vi "Q14070-Z060A.vi"() -> ()   [LabVIEW 2013]
uses:
  <vilib>/Utility/error.llb/whitespace.ctl
  <vilib>/Utility/file.llb/Read From Spreadsheet File (string).vi
  <vilib>/express/express arith-compare/Formula/XNode/ExpressFormulaBlockNode.xnode
  PCI8622_32.dll
  <vilib>/printing/EasyPrintingControls.llb/contents.ctl
  <vilib>/Utility/NIReport.llb/NI_ReportGenerationCore.lvlib
  <vilib>/printing/EasyPrintingControls.llb/report_type.ctl
  <vilib>/printing/EasyPrinting.llb/Easy Print VI Panel or Documentation (path).vi
  <vilib>/Utility/NIReport.llb/NI_report.lvclass
panel:
  out "齿条跑和右极限":dbl=10000.0 format="%#.3f"
  out "齿条跑和左极限":dbl=10000.0 format="%#.3f"
  in  "确定按钮 3":bool
  in  "确定按钮 2":bool
  in  "密码":string
  in  "确定按钮":bool
  in  "电动缸快速":dbl=15.0
  in  "电动缸慢速":dbl=1.0
  out "左轴向力数组大小":i32
  out "循环退出":bool
  in  "截取百分比":dbl=0.05
  in  "半行程":dbl=70.0
  in  "是否取消放行按钮":bool
  in  "齿条传动比":dbl=47.34 format="%#_13g"
  in  "机械间隙值":dbl=3.5
  out "最大轴向力标准(N)":dbl=200.0 caption="L+Lmax(mm)" format="%#.3f"
  out "右平均轴向力(N)":dbl caption="L+Lmax(mm)" format="%#.3f"
  out "左平均轴向力(N)":dbl caption="最大位移偏离Lmax(mm)" format="%#.3f"
  out "员工ID":string
  out "急停":bool
  out "报警":dbl
  out "报警提示":string
  out "DeviceHandle":u32
  in  "设定轴向力调整次数":dbl=6.0
  out "出支线工步号":u32
  in  "最小间隙(mm)":dbl=0.001 format="%#.3f"
  in  "测头气缸右移":bool
  in  "测头气缸左移":bool
  in  "轴向力已做次数":dbl
  out "全行程间隙及轴向力合格":bool
  out "轴向力启动":bool
  out "间隙启动":bool
  in  "夹头松开":bool
  in  "夹头夹紧":bool
  out "找帽扭矩":dbl=10.0 caption="压力传感器" format="%#.2f"
  out "error out":errorcluster
  out "型号数量":i32
  out "error out 4":errorcluster
  in  "设定间隙调整次数":dbl=6.0
  out "读取产品ID":string
  out "下工位备料":bool
  out "下工位测试":bool
  out "下工位自动":bool
  out "下工位备料H":bool
  out "下工位测试H":bool
  out "下工位自动H":bool
  out "FGCS":string
  out "KSJJ":string
  out "Z060ARFID":string
  out "轴向力Y":dbl[](array[numeric])
  out "轴向力X":dbl[](array[numeric])
  out "间隙X数组":dbl[](array[numeric])
  out "间隙Y数组":dbl[](array[numeric])
  out "error out 3":errorcluster caption="错误输出"
  out "rfid工步号":u32
  out "芯片ID":string="201209190001"
  out "rfid完成":bool
  out "rfid触发":bool
  out "本序已做":bool
  in  "回零完成":bool
  in  "电动缸回零":bool
  in  "已调试次数":dbl
  in  "需调整角度(度)":dbl
  in  "转向器中心":dbl
  out "扭矩到达":bool
  out "黄灯":bool
  out "红灯":bool
  in  "基准位移":dbl caption="压力传感器" format="%#.3f"
  out "上序不合格":bool
  out "单点间隙合格":bool
  out "上序合格":bool
  out "测头机构电机":u32
  out "复位":bool
  in  "型号选择":u16(ring)=2 items=["J709", "J728", "J706"]
  in  "联线按钮":bool
  in  "工步号":u32
  in  "产品ID":string="201209190001"
  out "间隙位移(mm)":dbl caption="压力传感器" format="%#.3f"
  out "齿条推拉力(N)":dbl format="%#.2f"
  out "齿条扭矩(Nm)":dbl format="%#.2f"
  out "通讯状态":bool
  out "员工姓名":string
  out "工步提示":string
  out "ADODB._Connection Out 2":refnum<k7>
  out "旋转齿条电机":u32
  out "电动缸电机":u32
  in  "停止":bool
  in  "参数加载":bool
  in  "选项卡控件":T1(tab)
  out "扭动曲线":cluster{"Y":dbl[], "Y":dbl[]}[](graph) caption="压球涨堵头1"
  out "中间位置间隙":dbl caption="间隙值L(mm)" format="%_2f"
  out "中间间隙标准(mm)":dbl=0.07 format="%#.3f"
  in  "找帽OK":bool
  out "全行程180°外间隙标准(mm)":dbl=0.1 format="%#.3f"
  out "右180°外全行程间隙":dbl caption="正向最大间隙L1(mm)" format="%_2f"
  out "左180°外全行程间隙":dbl caption="正向最大间隙L1(mm)" format="%_2f"
  out "右180°内全行程间隙":dbl caption="正向最大间隙L1(mm)" format="%_2f"
  out "左180°内全行程间隙":dbl caption="正向最大间隙L1(mm)" format="%_2f"
  out "全行程180°内间隙标准(mm)":dbl=0.07 format="%_1f"
  out "左全行程间隙":dbl caption="正向最大间隙L1(mm)" format="%#.3f"
  out "右全行程间隙":dbl caption="正向最大间隙L1(mm)" format="%#.3f"
  out "总圈数最大值":dbl format="%_3g"
  out "总圈数标准":dbl format="%_3g"
  out "总行程最大值":dbl
  out "总行程标准(mm)":dbl
  out "平均轴向力MAX(N)":dbl=200.0 caption="L+Lmax(mm)" format="%#.3f"
  out "力波动标准(N)":dbl=60.0 caption="L+Lmax(mm)" format="%#.3f"
  out "轴向力标准(N)":dbl=100.0 caption="L+Lmax(mm)" format="%#.3f"
  out "右最大轴向力(N)":dbl caption="L+Lmax(mm)" format="%#_5f"
  out "左轴向力波动(N)":dbl caption="最大位移偏离Lmax(mm)" format="%#_4f"
  out "左最大轴向力(N)":dbl caption="最大位移偏离Lmax(mm)" format="%#_5f"
  out "行程跳动曲线":cluster{"Y":dbl[], "Y":dbl[]}[](graph) caption="压球涨堵头1"
  out "右轴向力波动(N)":dbl format="%#_4f"
  out "总行程(mm)":dbl format="%#_5f"
  out "总圈数":dbl format="%.3g"
  in  "不合格品":bool
  in  "扭矩停止值":dbl=16.0
  in  "齿条右极限":dbl=-70.0 caption="压力传感器" format="%#.2f"
  in  "齿条左极限":dbl=-262.0 caption="压力传感器" format="%#.2f"
  in  "齿条移动速度":dbl=5.0 caption="压力传感器" format="%#.2f"
  in  "旋转伺服找帽转速":dbl=5.0 caption="压力传感器" format="%#.2f"
  in  "测量点扭矩":dbl=4.0 caption="压力传感器" format="%#.2f"
  in  "旋转伺服测量转速":dbl caption="压力传感器" format="%#.2f"
  in  "测头机构轴后退位":dbl=30.0 caption="压力传感器" format="%#.2f"
  in  "测头机构轴待检位":dbl caption="压力传感器" format="%#.2f"
  in  "测头机构轴检测位":dbl caption="压力传感器" format="%#.2f"
  in  "测头机构轴移动速度":dbl caption="压力传感器" format="%#.2f"
  out "点胶":bool
  in  "夹头松开":bool
  in  "夹头夹紧":bool
  in  "测头气缸右移":bool
  in  "测头气缸左移":bool
  in  "支线下降":bool
  in  "支线顶升":bool
  in  "出支线":bool
  in  "进支线":bool
  in  "主线下降":bool
  in  "主线顶升":bool
  in  "下阻挡器放行":bool
  in  "上阻挡器放行":bool
  out "夹头夹紧位":bool
  out "测头左位":bool
  out "测头右位":bool
  out "夹头松开":bool
  out "记号笔":bool
  in  "测头机构轴使能":bool
  in  "测头机构轴后退":bool
  in  "测头机构轴前进":bool
  in  "电动缸速度(mm/s)":dbl=10.0 format="%#.3f"
  out "电动缸位置(mm)":dbl=10000.0 format="%#.3f"
  in  "旋转伺服速度(°/s)":dbl=10.0 format="%#.3f"
  out "旋转伺服位置(°)":dbl=10000.0 format="%#.3f"
  in  "测头机构轴速度(mm/s)":dbl=10.0 format="%#.3f"
  out "测头机构轴位置(mm)":dbl=10000.0 format="%#.3f"
  in  "旋转齿条轴右转":bool
  in  "旋转齿条轴左转":bool
  in  "旋转齿条轴使能":bool
  in  "电动缸后退":bool
  in  "电动缸使能":bool
  in  "电动缸前进":bool
  in  "齿条扭矩比例偏移":dbl=1.0 format="%#.2f"
  in  "齿条扭矩零点偏移":dbl format="%#.2f"
  in  "齿条推拉力比例偏移":dbl=1.0 format="%#.2f"
  in  "齿条推拉力零点偏移":dbl format="%#.2f"
  in  "间隙位移比例偏移":dbl=1.0 format="%#.2f"
  in  "间隙位移零点偏移":dbl format="%#.2f"
  in  "传感器参数保存":bool
  in  "参数修改":bool
  in  "参数查询":bool
  in  "参数浏览表":string[][](table)
  # "芜湖机械转向器装配线"
  # "间隙及轴向力检测"
  # "Q14070机械转向器装配线"
  # "湖北唯思凌科装备制造有限公司 设计开发 (C)2015"
  # "≤"
  # "间隙测量判定值"
  # "间隙测量结果"
  # "≤"
  # "≤"
  # "≤"
  # "轴向力测量结果"
  # "轴向力测量标准"
  # "≤"
  # "≥"
  # "≤"
  # "≥"
  # "≤"
  # "≥"
  # "≤"
  # "不得大于20NM"
  # "传感器校验区"
  # "关于传感器校验：\n1、传感器校验需要由具备资质的单位或部门进行校验。\n2、具备权限的用户才能够修改传感器校验参数和试验参数。\n3、修改校验参数方法：先将比例偏移置为1，修改零点偏移，使零点值与校验的传感器一致；然后根据增幅调整比例偏移。"
  # "注意：\n具备权限的用户才能够修改传感器校验参数和试验参数！"
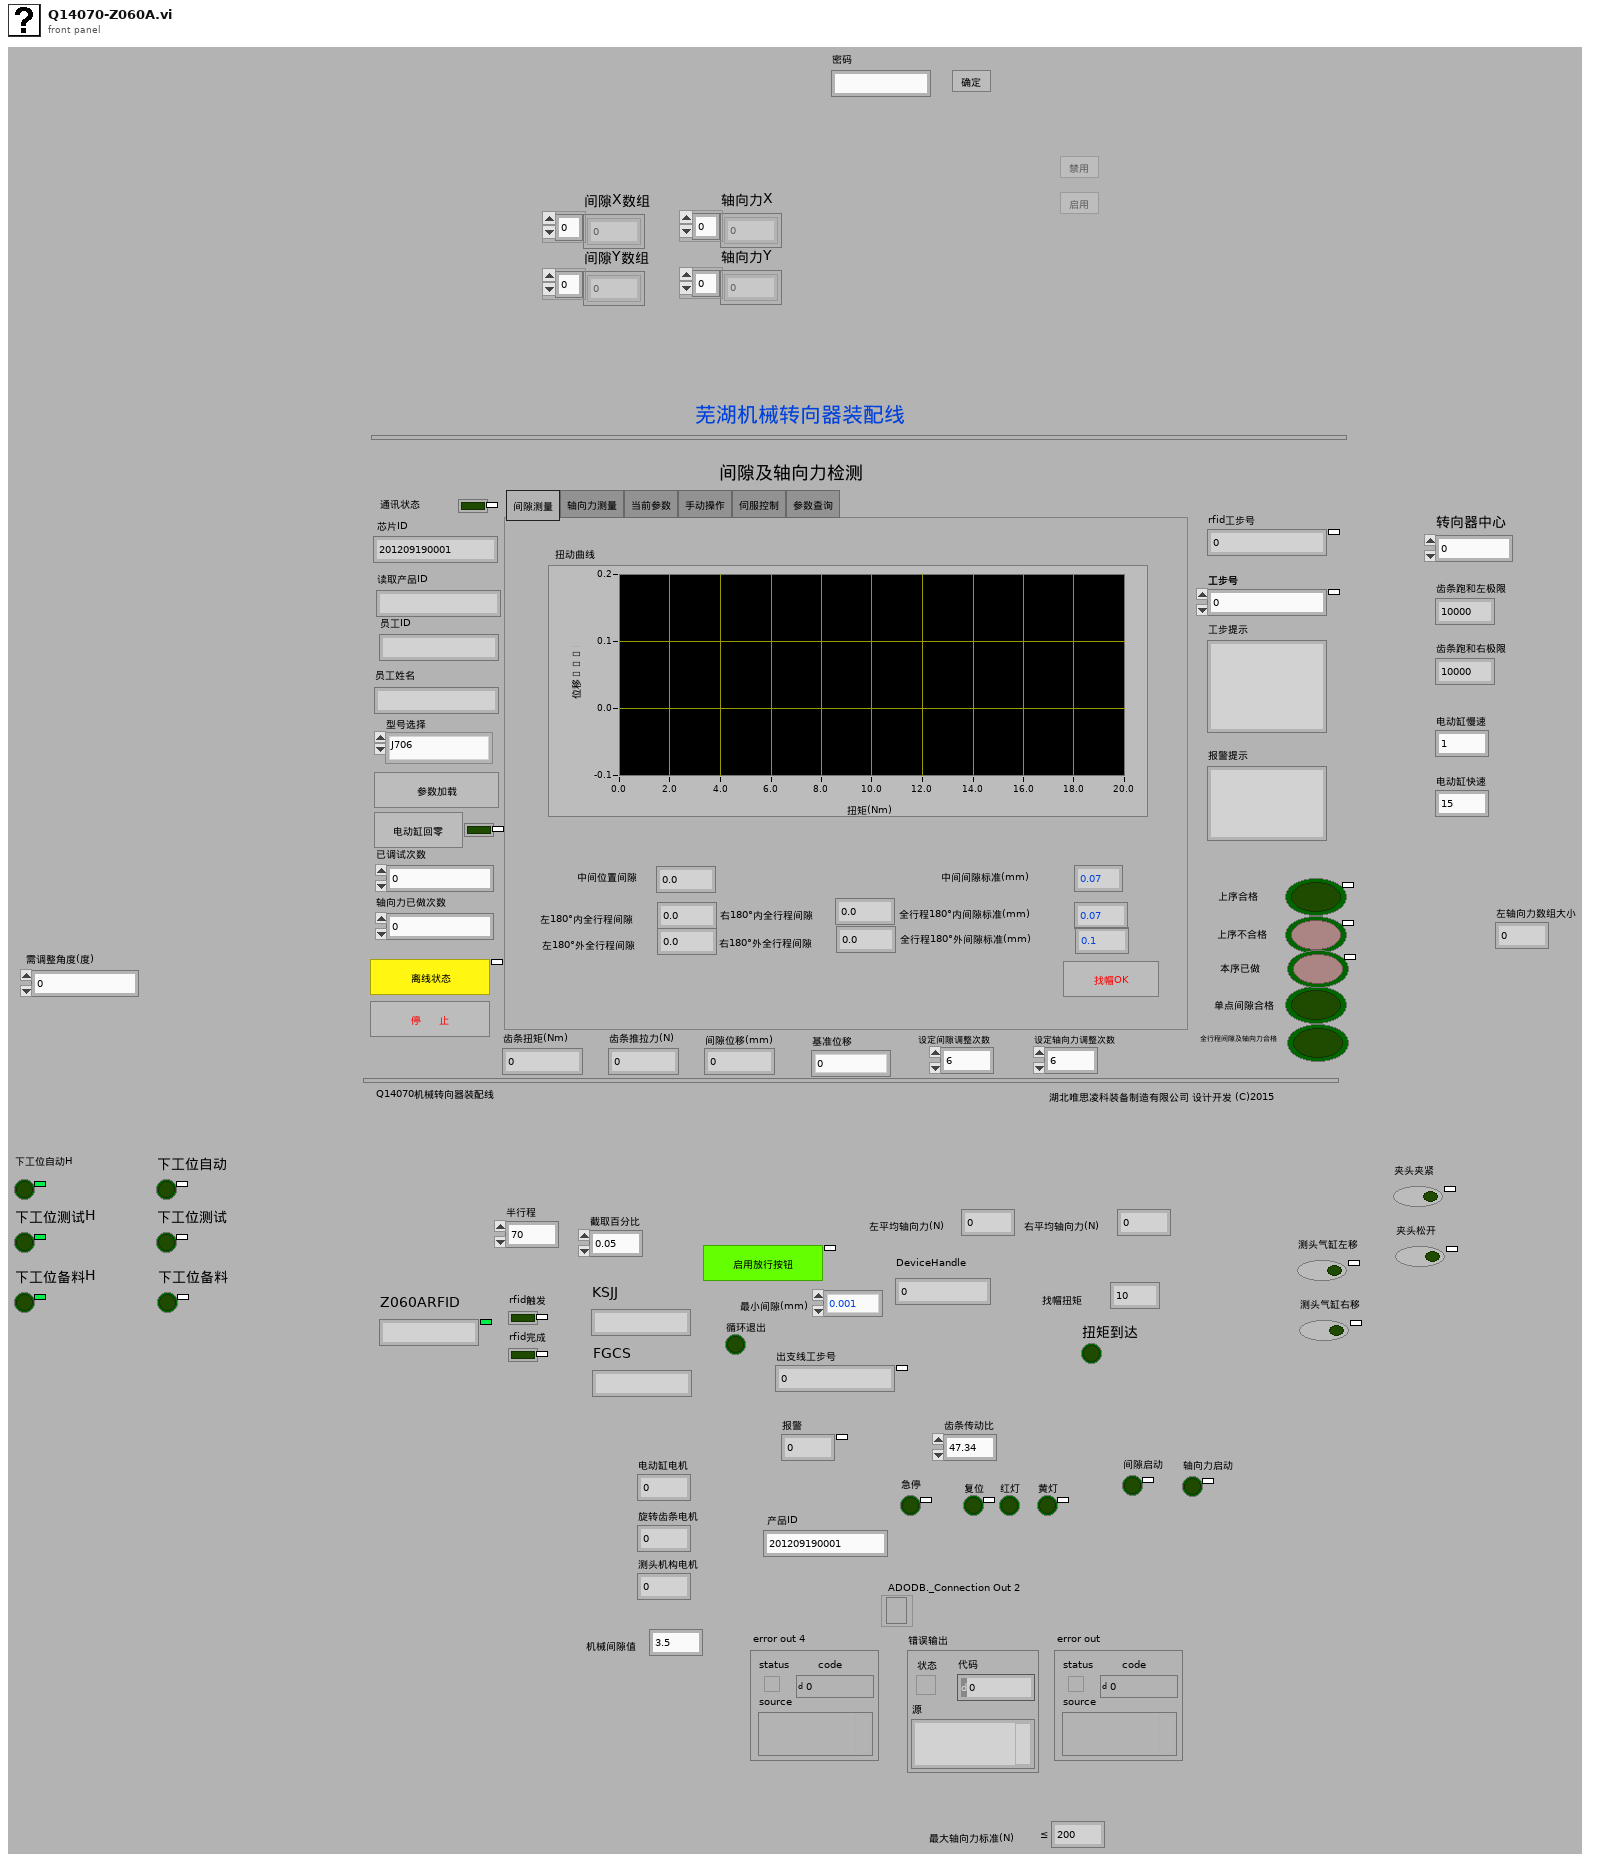
[diagram p1: front panel]
types:
  T1 = enum32{"间隙测量", "轴向力测量", "当前参数", "手动操作", "伺服控制", "传感器校验", "参数查询"}
  T2 = enum8{"Enabled", "Disabled", "Disabled and Grayed Out"}
  T3 = typedef "NI_ReportGenerationCore.lvlib/report_type.ctl" = u16
  T4 = typedef "NI_ReportGenerationCore.lvlib/contents.ctl" = u16
  T5 = typedef "imagedata.ctl" = cluster{"image type":i32, "image depth":i32, "image":u8[], "mask":u8[], "colors":u32[], "Rectangle":cluster{"left":i16, "top":i16, "right":i16, "bottom":i16}}
  T6 = typedef "whitespace.ctl" = u16
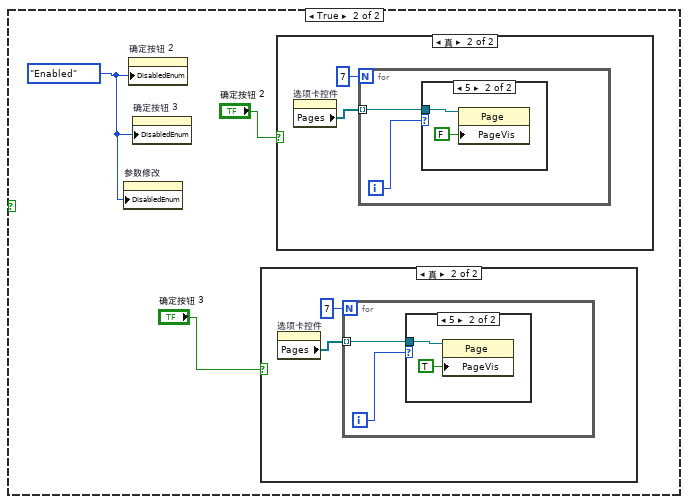
[diagram p2: hidden frame]
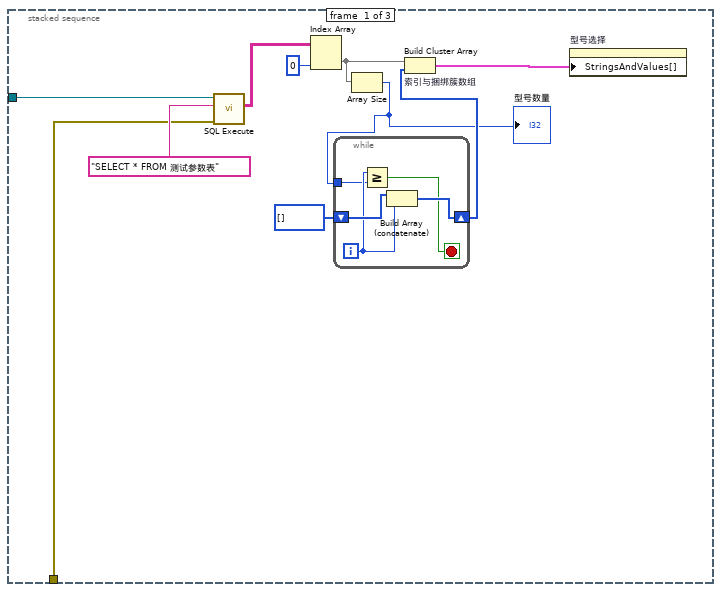
[diagram p9: hidden frame]
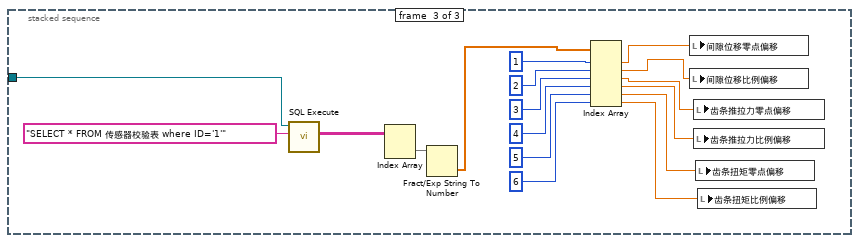
[diagram p10: hidden frame]
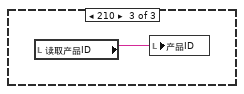
[diagram p12: hidden frame]
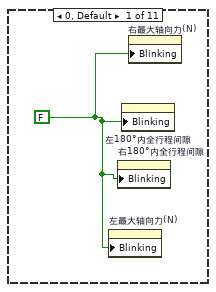
[diagram p13: hidden frame]
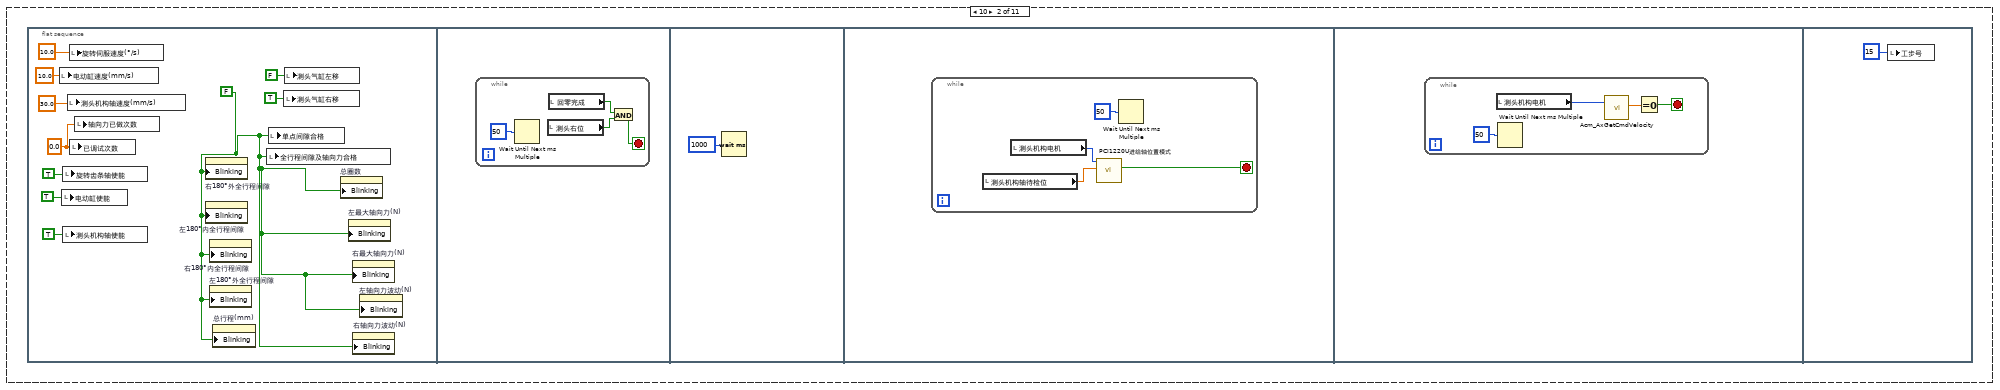
[diagram p14: hidden frame]
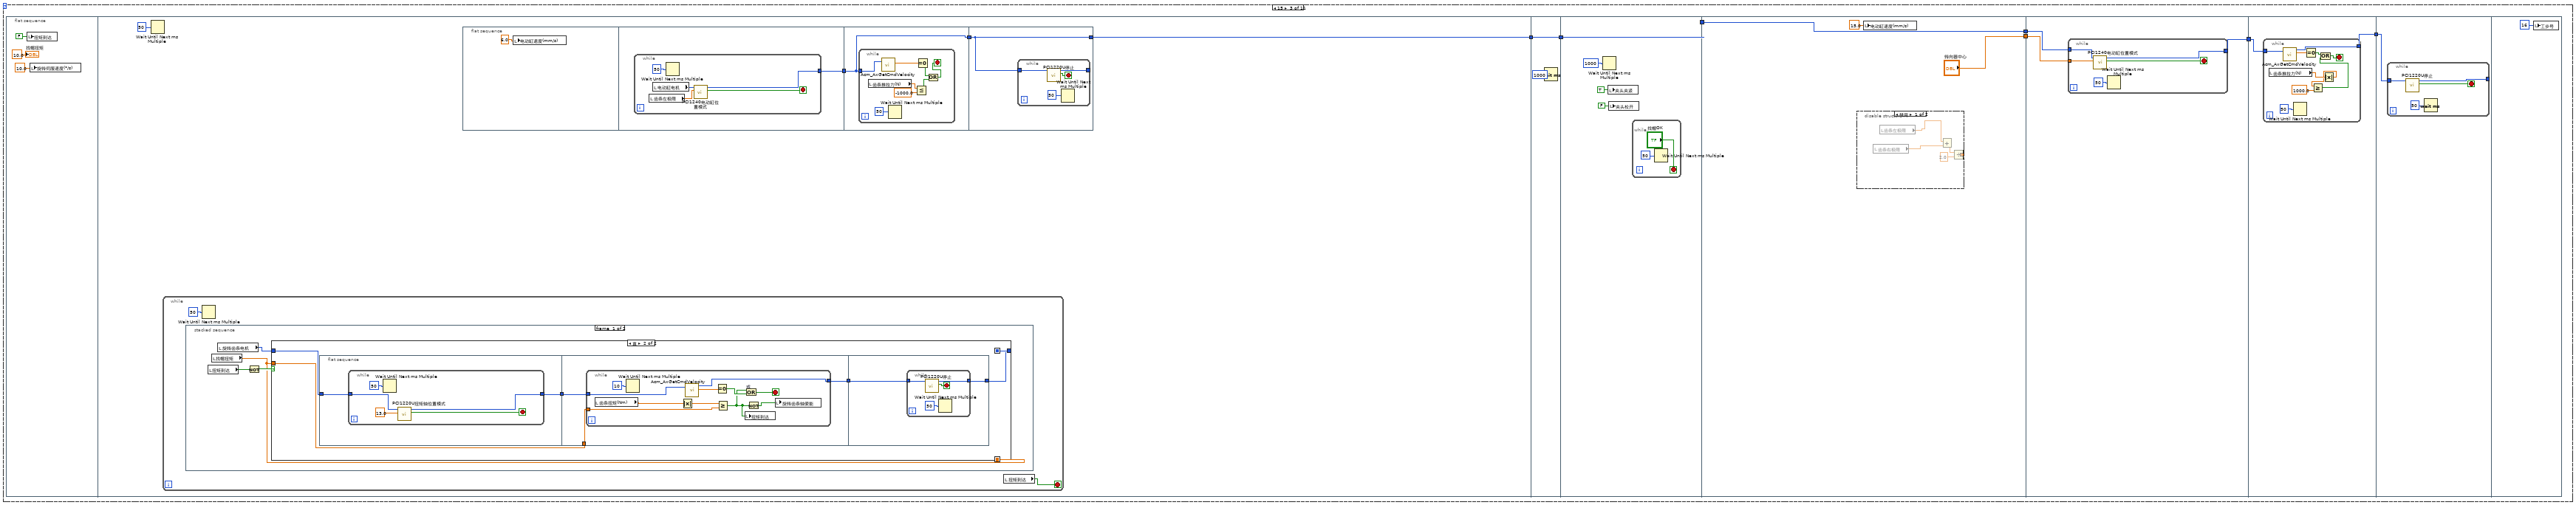
[diagram p15: hidden frame]
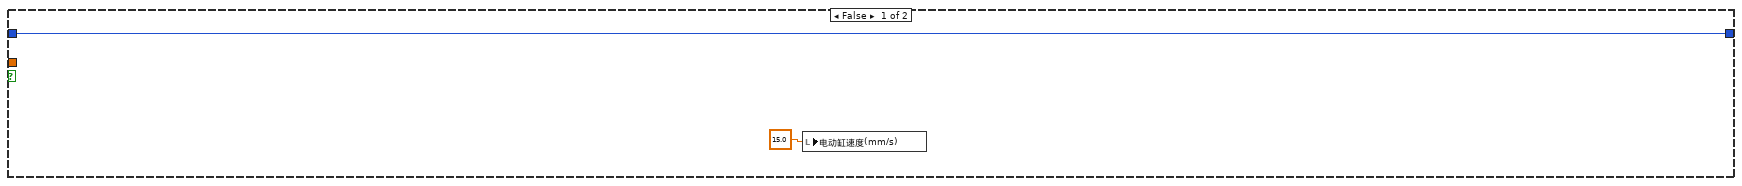
[diagram p16: hidden frame]
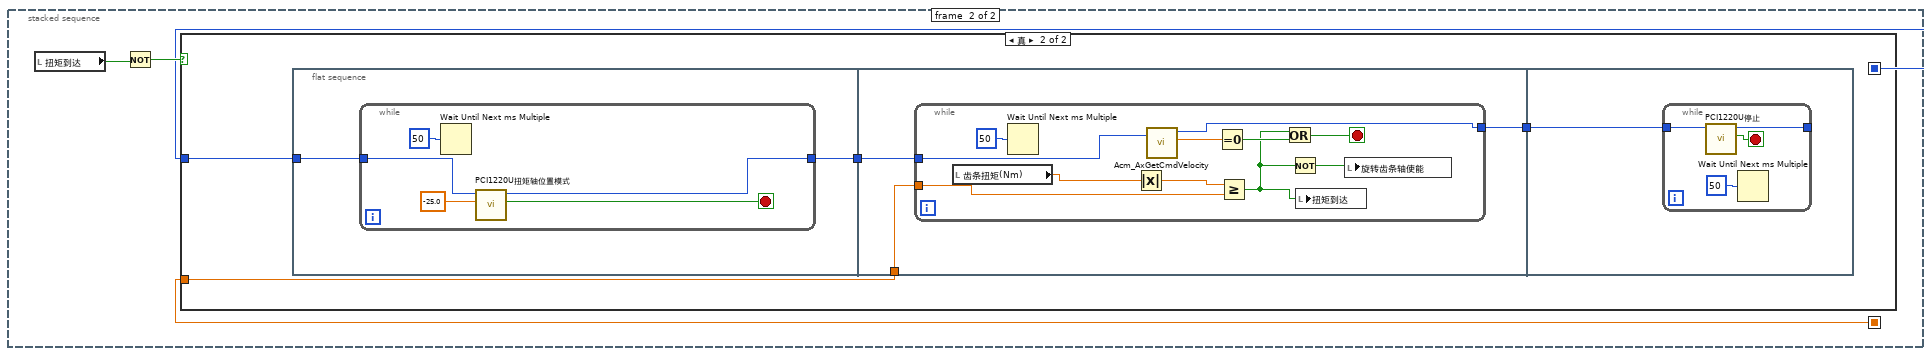
[diagram p17: hidden frame]
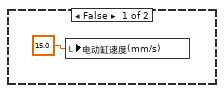
[diagram p18: hidden frame]
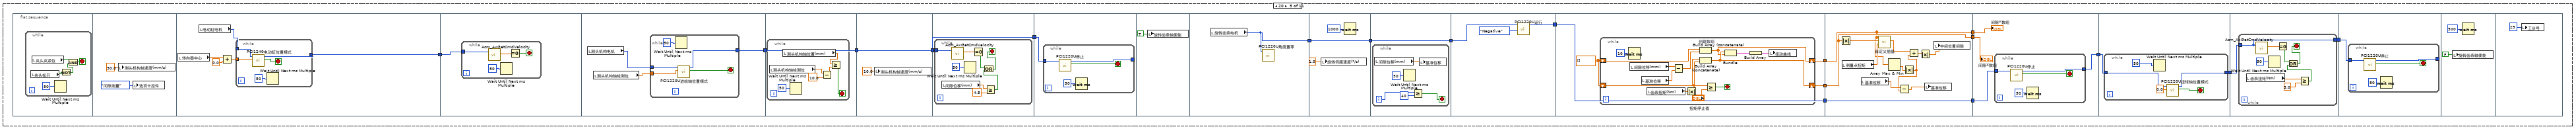
[diagram p20: hidden frame]
diagram:
  n1 = while {
    stop <- w5 stop-if-true
    n2 = event shown="[2] \"参数修改\": 值改变" {
      selector: _ -> [_ _ _ _ _ _]
      dyn-events: _ -> [_ _ _ _ _ _]
      timeout: 500 -> [_ _ _ _ _ _]
      event Timeout {
        n3 = event-data() -> ()  [unwired: 3 out]
      }
      event "停止": Value Change {
        n4 = event-data() -> ()  [unwired: 6 out]
        n5 = flat-sequence {
          frame #0 {
            n6 = Wait (ms)(milliseconds to wait=u32 1000 ("毫秒倍数")) -> ()  [unwired: 1 out]
          }
          frame #1 {
            n7 = Quit LabVIEW(quit? (T)=TRUE ("停止？(T)")) -> ()
          }
        }
      }
      event "参数修改": Value Change {
        n8 = event-data() -> ()  [unwired: 6 out]
        n9 = while {
          i -> [w63]
          stop <- w62 stop-if-true
          n10 = local read "型号数量"() -> (w64:i32)
          n11 = local read "参数浏览表"() -> (w65:string[][])
          n12 = Greater Or Equal?(x=w63, y=w64) -> (x >= y?=w62:bool)
          n13 = Wait Until Next ms Multiple(millisecond multiple=u32 50 ("毫秒倍数")) -> ()  [unwired: 1 out]
          n14 = Index Array(array=w65, index (col)=w63) -> (element=w50:string[])  [unwired: 1 in]
          n15 = Index Array(array=w50, index #1=0 ("索引"), index #2=2 ("索引"), index #3=3 ("索引"), index #4=4 ("索引"), index #5=5 ("索引"), index #6=6 ("索引"), index #7=7 ("索引"), index #8=8 ("索引"), index #9=9 ("索引"), index #10=10 ("索引"), index #11=11 ("索引"), index #12=12 ("索引"), index #13=13 ("索引"), index #14=14 ("索引"), index #15=15 ("索引"), index #16=16 ("索引"), index #17=17 ("索引"), index #18=18 ("索引"), index #19=19 ("索引"), index #20=20 ("索引"), index #21=21 ("索引"), index #22=22 ("索引"), index #23=23 ("索引")) -> (element #1=w16:string, element #2=w46:string, element #3=w45:string, element #4=w44:string, element #5=w43:string, element #6=w42:string, element #7=w41:string, element #8=w40:string, element #9=w39:string, element #10=w38:string, element #11=w37:string, element #12=w32:string, element #13=w31:string, element #14=w30:string, element #15=w29:string, element #16=w28:string, element #17=w23:string, element #18=w22:string, element #19=w21:string, element #20=w17:string, element #21=w15:string, element #22=w14:string, element #23=w13:string)
          n16 = call "创建文本"("测头机构轴移动速度"=w46, "测头机构轴检测位"=w45, "测头机构轴待检位"=w44, "测头机构轴后退位"=w43, "齿条移动速度"=w42, "齿条左极限"=w41, "齿条右极限"=w40, "旋转齿条轴找帽转速"=w39, "旋转齿条轴测量转速"=w38, "测量点扭矩"=w37, "总行程最大值"=w31, "总行程最小值"=w32, "最大轴向力"=w30, "轴向力波动"=w29, "平均轴向力最小值"=w28, "平均轴向力最大值"=w23, "总圈数最小值"=w22, "总圈数最大值"=w21, "中间位置"=w17, "中间间隙标准"=w15, "180内间隙标准"=w14, "180外间隙标准"=w13, "产品型号"=w16) -> ("Result"=w36:string)  [unwired: 3 in, 1 out]
          n17 = local read "ADODB._Connection Out 2"() -> (w35:refnum<k7>)
          n18 = call "SQL Execute.vi"("Command Text"=w36, "ADODB._Connection In"=w35) -> ("error out"=w48:errorcluster, "ADODB._Connection Out"=w49:refnum<k7>)  [unwired: 6 in, 2 out]
          n19 = call "ADO Connection Close.vi"("error in (no error)"=w48, "ADODB._Connection In"=w49) -> ("error out"=→"error out":errorcluster)  [unwired: 8 in, 1 out]
        }
      }
      event "参数查询": Value Change {
        n20 = event-data() -> ()  [unwired: 6 out]
        n21 = flat-sequence {
          tunnel: [w78] -> w71
          tunnel: [w77] -> w70
          tunnel: [w76] -> w67
          tunnel: w71 -> [w82]
          tunnel: w70 -> [w84]
          tunnel: [w84] -> w69
          tunnel: [w83] -> w68
          tunnel: w67 -> [w83]
          tunnel: w69 -> [_]
          tunnel: w68 -> [_]
          frame #0 {
            n22 = call-poly <vilib>:"Read From Spreadsheet File.vi"("file path (dialog if empty)"=path "D:/Q14070-Z060人机界面/参数/参数项.txt") -> ("first row"=w72:string[])  [unwired: 6 in, 4 out]
            n23 = property on="参数浏览表" class="Tbl (严格)"("Row Headers[]"=w72) -> ()  [unwired: 2 in, 2 out]
          }
          frame #1 {
            n24 = local read "ADODB._Connection Out 2"() -> (w75:refnum<k7>)
            n25 = call "SQL Execute.vi"("Command Text"="SELECT * FROM 测试参数表;", "ADODB._Connection In"=w75) -> ("error out"=w76:errorcluster, "Data"=w80:string[][], "ADODB._Connection Out"=w77:refnum<k7>)  [unwired: 6 in, 1 out]
            n26 = Transpose 2D Array(2D array=w80) -> (transposed array=w78:string[][])
            n27 = Index Array(array=w78, index (row)=0 ("索引 (行)")) -> (element=w79:string[])  [unwired: 1 in]
            n28 = property on="参数浏览表" class="Tbl (严格)"("Column Headers[]"=w79) -> ()  [unwired: 2 in, 2 out]
          }
          frame #2 {
            n29 = local write "参数浏览表"(w82) -> ()
          }
          frame #3 {
          }
        }
      }
      event "传感器参数保存": Value Change {
        n30 = event-data() -> ()  [unwired: 6 out]
        n31 = flat-sequence {
          tunnel: [w110] -> w107
          tunnel: [w109] -> w106
          tunnel: [w108] -> w105
          tunnel: [w116] -> w104
          tunnel: w107 -> [w116]
          tunnel: [w115] -> w103
          tunnel: w106 -> [w115]
          tunnel: [w114] -> w102
          tunnel: w105 -> [w114]
          tunnel: [w113] -> w101
          tunnel: [w112] -> w100
          tunnel: [w111] -> w99
          tunnel: [w117] -> w98
          tunnel: [w123] -> w97
          tunnel: w104 -> [w123]
          tunnel: [w122] -> w96
          tunnel: w103 -> [w122]
          tunnel: w102 -> [w121]
          tunnel: [w121] -> w95
          tunnel: [w120] -> w94
          tunnel: w101 -> [w120]
          tunnel: [w119] -> w93
          tunnel: w100 -> [w119]
          tunnel: [w118] -> w92
          tunnel: w99 -> [w118]
          tunnel: w98 -> [w142]
          tunnel: [w142] -> w91
          tunnel: w97 -> [w141]
          tunnel: w96 -> [w134]
          tunnel: w95 -> [w133]
          tunnel: w94 -> [w127]
          tunnel: w93 -> [w126]
          tunnel: w92 -> [w132]
          tunnel: [w131] -> w90
          tunnel: [w130] -> w89
          tunnel: [w129] -> w88
          tunnel: [w125] -> w87
          tunnel: [w124] -> w86
          tunnel: [w128] -> w85
          tunnel: w91 -> [w150]
          tunnel: w90 -> [w149]
          tunnel: w89 -> [w148]
          tunnel: w88 -> [w147]
          tunnel: w87 -> [w146]
          tunnel: w86 -> [w145]
          tunnel: w85 -> [w144]
          frame #0 {
            n32 = local read "齿条推拉力零点偏移"() -> (w109:dbl)
            n33 = local read "间隙位移零点偏移"() -> (w110:dbl)
            n34 = local read "齿条扭矩零点偏移"() -> (w108:dbl)
          }
          frame #1 {
            n35 = local read "齿条推拉力比例偏移"() -> (w112:dbl)
            n36 = local read "间隙位移比例偏移"() -> (w113:dbl)
            n37 = local read "齿条扭矩比例偏移"() -> (w111:dbl)
          }
          frame #2 {
            n38 = local read "ADODB._Connection Out 2"() -> (w117:refnum<k7>)
          }
          frame #3 {
            n39 = Number To Fractional String(number=w141, precision (6)=i16 2 ("精度(6)")) -> (F-format string=w131:string)  [unwired: 2 in]
            n40 = Number To Fractional String(number=w133, precision (6)=i16 2 ("精度(6)")) -> (F-format string=w129:string)  [unwired: 2 in]
            n41 = Number To Fractional String(number=w132, precision (6)=i16 2 ("精度(6)")) -> (F-format string=w128:string)  [unwired: 2 in]
            n42 = Number To Fractional String(number=w134, precision (6)=i16 2 ("精度(6)")) -> (F-format string=w130:string)  [unwired: 2 in]
            n43 = Number To Fractional String(number=w127, precision (6)=i16 2 ("精度(6)")) -> (F-format string=w125:string)  [unwired: 2 in]
            n44 = Number To Fractional String(number=w126, precision (6)=i16 2 ("精度(6)")) -> (F-format string=w124:string)  [unwired: 2 in]
          }
          frame #4 {
            n45 = call "创建文本3"("4"=w146, "6"=w144, "1"=w149, "2"=w148, "3"=w147, "5"=w145) -> ("Result"=w151:string)  [unwired: 8 in, 1 out]
            n46 = call "SQL Execute.vi"("Command Text"=w151, "ADODB._Connection In"=w150) -> ("error out"=→"error out 4":errorcluster)  [unwired: 6 in, 3 out]
          }
        }
      }
      event "产品ID": Value Change {
        n47 = event-data() -> ()  [unwired: 7 out]
        n48 = Format Date/Time String(time format string (%c)="%Y%m%d%H%M" ("时间格式字符串(%c)")) -> (date/time string=w152:string)  [unwired: 2 in]
        n49 = local write "KSJJ"(w152) -> ()
      }
    }
    n50 = Wait (ms)(milliseconds to wait=u32 50 ("毫秒倍数")) -> ()  [unwired: 1 out]
    n51 = local read "停止"() -> (w5:bool)
  }
  n52 = while {
    stop <- FALSE stop-if-true
    n53 = Equal?(x="密码", y="jizhuan") -> (x = y?=w157:bool)
    n54 = Compound Arithmetic op=AND(w157, "确定按钮") -> (w155:bool)
    n55 = case shown="假" w155 {
      frame False {
        w160 = T2."Disabled and Grayed Out" ("禁用")
        n56 = property on="确定按钮 2" class="Bool"("DisabledEnum"=w160) -> ()  [unwired: 2 in, 2 out]
        n57 = property on="确定按钮 3" class="Bool"("DisabledEnum"=w160) -> ()  [unwired: 2 in, 2 out]
        n58 = property on="参数修改" class="Bool"("DisabledEnum"=w160) -> ()  [unwired: 2 in, 2 out]
      }
      frame True {
        w161 = T2."Enabled" ("禁用")
        n59 = property on="参数修改" class="Bool"("DisabledEnum"=w161) -> ()  [unwired: 2 in, 2 out]
        n60 = property on="确定按钮 2" class="Bool"("DisabledEnum"=w161) -> ()  [unwired: 2 in, 2 out]
        n61 = property on="确定按钮 3" class="Bool"("DisabledEnum"=w161) -> ()  [unwired: 2 in, 2 out]
        n62 = case shown="真" "确定按钮 3" {
          frame False {
          }
          frame True {
            n63 = property on="选项卡控件" class="TabCtl (严格)"() -> ("Pages"=w164:refnum<vi>[])  [unwired: 2 in, 2 out]
            n64 = for {
              N: 7 -> [_]
              tunnel: w164 -> [w166] mode=indexing
              i -> [w167]
              n65 = case shown="5" w167 {
                tunnel: w166 -> [_ w169]
                frame 0, Default {
                }
                frame 5 {
                  n66 = property class="Page"(reference=w169, "PageVis"=TRUE ("选项卡可见")) -> ()  [unwired: 1 in, 2 out]
                }
              }
            }
          }
        }
        n67 = case shown="真" "确定按钮 2" {
          frame False {
          }
          frame True {
            n68 = property on="选项卡控件" class="TabCtl (严格)"() -> ("Pages"=w170:refnum<vi>[])  [unwired: 2 in, 2 out]
            n69 = for {
              N: 7 -> [_]
              tunnel: w170 -> [w172] mode=indexing
              i -> [w173]
              n70 = case shown="5" w173 {
                tunnel: w172 -> [_ w175]
                frame 0, Default {
                }
                frame 5 {
                  n71 = property class="Page"(reference=w175, "PageVis"=FALSE ("选项卡可见")) -> ()  [unwired: 1 in, 2 out]
                }
              }
            }
          }
        }
      }
    }
  }
  n72 = while {
    stop <- w178 stop-if-true
    n73 = local read "工步号"() -> (w176:u32)
    n74 = case shown="16" w176 {
      frame 0, Default {
        w179 = FALSE ("闪烁")
        n75 = property on="左最大轴向力(N)" class="DigNum (严格)"("Blinking"=w179) -> ()  [unwired: 2 in, 2 out]
        n76 = property on="右180°内全行程间隙" class="DigNum (严格)"("Blinking"=w179) -> ()  [unwired: 2 in, 2 out]
        n77 = property on="左180°内全行程间隙" class="DigNum (严格)"("Blinking"=w179) -> ()  [unwired: 2 in, 2 out]
        n78 = property on="右最大轴向力(N)" class="DigNum (严格)"("Blinking"=w179) -> ()  [unwired: 2 in, 2 out]
      }
      frame 10 {
        n79 = flat-sequence {
          frame #0 {
            w180 = FALSE ("单点间隙合格")
            w181 = 0.0 ("已调试次数")
            n80 = local write "电动缸速度(mm/s)"(10.0 ("电动缸速度(mm/s)")) -> ()
            n81 = local write "电动缸使能"(TRUE ("电动缸使能")) -> ()
            n82 = local write "旋转齿条轴使能"(TRUE ("旋转齿条轴使能")) -> ()
            n83 = local write "测头机构轴使能"(TRUE ("调整机构轴使能")) -> ()
            n84 = local write "测头机构轴速度(mm/s)"(30.0 ("调整机构轴速度(mm/s)")) -> ()
            n85 = local write "旋转伺服速度(°/s)"(10.0 ("旋转齿条轴速度(°/s)")) -> ()
            n86 = local write "已调试次数"(w181) -> ()
            n87 = local write "轴向力已做次数"(w181) -> ()
            n88 = property on="右180°外全行程间隙" class="DigNum (严格)"("Blinking"=w180) -> ()  [unwired: 2 in, 2 out]
            n89 = property on="左180°内全行程间隙" class="DigNum (严格)"("Blinking"=w180) -> ()  [unwired: 2 in, 2 out]
            n90 = property on="右180°内全行程间隙" class="DigNum (严格)"("Blinking"=w180) -> ()  [unwired: 2 in, 2 out]
            n91 = property on="左180°外全行程间隙" class="DigNum (严格)"("Blinking"=w180) -> ()  [unwired: 2 in, 2 out]
            n92 = property on="总行程(mm)" class="DigNum (严格)"("Blinking"=w180) -> ()  [unwired: 2 in, 2 out]
            n93 = local write "全行程间隙及轴向力合格"(w180) -> ()
            n94 = local write "单点间隙合格"(w180) -> ()
            n95 = local write "测头气缸右移"(TRUE ("测头气缸右移")) -> ()
            n96 = local write "测头气缸左移"(FALSE ("测头气缸左移")) -> ()
            n97 = property on="总圈数" class="DigNum (严格)"("Blinking"=w180) -> ()  [unwired: 2 in, 2 out]
            n98 = property on="左最大轴向力(N)" class="DigNum (严格)"("Blinking"=w180) -> ()  [unwired: 2 in, 2 out]
            n99 = property on="右最大轴向力(N)" class="DigNum (严格)"("Blinking"=w180) -> ()  [unwired: 2 in, 2 out]
            n100 = property on="右轴向力波动(N)" class="DigNum (严格)"("Blinking"=w180) -> ()  [unwired: 2 in, 2 out]
            n101 = property on="左轴向力波动(N)" class="DigNum (严格)"("Blinking"=w180) -> ()  [unwired: 2 in, 2 out]
          }
          frame #1 {
            n102 = while {
              stop <- w190 stop-if-true
              n103 = Wait Until Next ms Multiple(millisecond multiple=u32 50 ("毫秒倍数")) -> ()  [unwired: 1 out]
              n104 = local read "测头右位"() -> (w191:bool)
              n105 = local read "回零完成"() -> (w192:bool)
              n106 = And(x=w192, y=w191) -> (x .and. y?=w190:bool)
            }
          }
          frame #2 {
            n107 = Wait (ms)(milliseconds to wait=u32 1000 ("等待时间（毫秒）")) -> ()  [unwired: 1 out]
          }
          frame #3 {
            n108 = while {
              stop <- w198 stop-if-true
              n109 = local read "测头机构轴待检位"() -> (w195:dbl)
              n110 = local read "测头机构电机"() -> (w196:u32)
              n111 = call "PCI1220U进给轴位置模式.vi"("Distance"=w195, "AxisHandle IN"=w196) -> ("AbsSuccess"=w198:bool)  [unwired: 8 in, 1 out]
              n112 = Wait Until Next ms Multiple(millisecond multiple=u32 50 ("毫秒倍数")) -> ()  [unwired: 1 out]
            }
          }
          frame #4 {
            n113 = while {
              stop <- w201 stop-if-true
              n114 = local read "测头机构电机"() -> (w199:u32)
              n115 = Wait Until Next ms Multiple(millisecond multiple=u32 50 ("毫秒倍数")) -> ()  [unwired: 1 out]
              n116 = call <userlib>:"Acm_AxGetCmdVelocity.vi"("AxisHandle"=w199) -> ("Velocity"=w202:dbl)  [unwired: 1 in, 3 out]
              n117 = Equal To 0?(x=w202) -> (x = 0?=w201:bool)
            }
          }
          frame #5 {
            n118 = local write "工步号"(u32 15 ("工步号")) -> ()
          }
        }
      }
      frame 15 {
        n119 = flat-sequence {
          tunnel: [w215] -> w205
          tunnel: w205 -> [w316]
          tunnel: [w316] -> w204
          tunnel: w204 -> [w319]
          tunnel: [w319] -> w207
          tunnel: [w324] -> w210
          tunnel: ["转向器中心"] -> w209
          tunnel: w207 -> [w324]
          tunnel: w210 -> [w333]
          tunnel: w209 -> [w332]
          tunnel: [w331] -> w208
          tunnel: w208 -> [w340]
          tunnel: [w339] -> w206
          tunnel: w206 -> [w351]
          frame #0 {
            n120 = local write "扭矩到达"(FALSE ("扭矩到达")) -> ()
            n121 = local write "旋转伺服速度(°/s)"(10.0 ("旋转齿条轴速度(°/s)")) -> ()
            "找帽扭矩" <- 10.0 ("找帽扭矩")
          }
          frame #1 {
            n122 = Wait Until Next ms Multiple(millisecond multiple=u32 50 ("毫秒倍数")) -> ()  [unwired: 1 out]
            n123 = while {
              stop <- w218 stop-if-true
              n124 = stacked-sequence {
                seq-local: [w220 _] -> [_ w261]
                seq-local: [w224 _] -> [_ w260]
                frame #0 {
                  n125 = local read "扭矩到达"() -> (w222:bool)
                  n126 = local read "找帽扭矩"() -> (w220:dbl)
                  n127 = local read "旋转齿条电机"() -> (w221:u32)
                  n128 = Not(x=w222) -> (.not. x?=w223:bool)
                  n129 = case shown="真" w223 {
                    tunnel: [w226 w227] -> w224
                    tunnel: w221 -> [w226 w231]
                    tunnel: w220 -> [_ w229]
                    frame False {
                      n130 = local write "电动缸速度(mm/s)"(15.0 ("电动缸速度(mm/s)")) -> ()
                    }
                    frame True {
                      n131 = flat-sequence {
                        tunnel: w231 -> [w233]
                        tunnel: [w232] -> w230
                        tunnel: w230 -> [w241]
                        tunnel: w229 -> [w240]
                        tunnel: [w239] -> w228
                        tunnel: w228 -> [w254]
                        tunnel: [w253] -> w227
                        frame #0 {
                          n132 = while {
                            tunnel: [w237] -> w232
                            tunnel: w233 -> [w234]
                            stop <- w236 stop-if-true
                            n133 = Wait Until Next ms Multiple(millisecond multiple=u32 50 ("毫秒倍数")) -> ()  [unwired: 1 out]
                            n134 = call "PCI1220U扭矩轴位置模式.vi"("Distance"=13.0, "AxisHandle IN"=w234) -> ("AbsSuccess"=w236:bool, "AxisHandle OUT"=w237:u32)  [unwired: 8 in]
                          }
                        }
                        frame #1 {
                          n135 = while {
                            tunnel: w241 -> [w251]
                            tunnel: w240 -> [w246]
                            tunnel: [w245] -> w239
                            stop <- w247 stop-if-true
                            n136 = local read "齿条扭矩(Nm)"() -> (w244:dbl)
                            n137 = Wait Until Next ms Multiple(millisecond multiple=u32 10 ("毫秒倍数")) -> ()  [unwired: 1 out]
                            n138 = Absolute Value(x=w244) -> (abs(x)=w249:dbl)
                            n139 = call <userlib>:"Acm_AxGetCmdVelocity.vi"("AxisHandle"=w251) -> ("Velocity"=w250:dbl, "AxisHandle"=w245:u32)  [unwired: 1 in, 2 out]
                            n140 = Equal To 0?(x=w250) -> (x = 0?=w248:bool)
                            n141 = Greater Or Equal?(x=w249, y=w246) -> (x >= y?=w243:bool)
                            n142 = Or "或"(x=w243, y=w248) -> (x .or. y?=w247:bool)
                            n143 = local write "扭矩到达"(w243) -> ()
                            n144 = Not(x=w243) -> (.not. x?=w242:bool)
                            n145 = local write "旋转齿条轴使能"(w242) -> ()
                          }
                        }
                        frame #2 {
                          n146 = while {
                            tunnel: w254 -> [w258]
                            tunnel: [w255] -> w253
                            stop <- w257 stop-if-true
                            n147 = call "PCI1220U停止.vi"("AxisHandle IN"=w258) -> ("完成"=w257:bool, "AxisHandle OUT"=w255:u32)  [unwired: 9 in]
                            n148 = Wait Until Next ms Multiple(millisecond multiple=u32 50 ("毫秒倍数")) -> ()  [unwired: 1 out]
                          }
                        }
                      }
                    }
                  }
                }
                frame #1 {
                  n149 = local read "扭矩到达"() -> (w259:bool)
                  n150 = Not(x=w259) -> (.not. x?=w262:bool)
                  n151 = case shown="真" w262 {
                    tunnel: w260 -> [_ w267]
                    tunnel: w261 -> [_ w265]
                    frame False {
                      n152 = local write "电动缸速度(mm/s)"(15.0 ("电动缸速度(mm/s)")) -> ()
                    }
                    frame True {
                      n153 = flat-sequence {
                        tunnel: w267 -> [w268]
                        tunnel: [w269] -> w266
                        tunnel: w266 -> [w277]
                        tunnel: w265 -> [w276]
                        tunnel: [w275] -> w264
                        tunnel: w264 -> [w289]
                        frame #0 {
                          n154 = while {
                            tunnel: [w273] -> w269
                            tunnel: w268 -> [w270]
                            stop <- w272 stop-if-true
                            n155 = Wait Until Next ms Multiple(millisecond multiple=u32 50 ("毫秒倍数")) -> ()  [unwired: 1 out]
                            n156 = call "PCI1220U扭矩轴位置模式.vi"("Distance"=-25.0, "AxisHandle IN"=w270) -> ("AbsSuccess"=w272:bool, "AxisHandle OUT"=w273:u32)  [unwired: 8 in]
                          }
                        }
                        frame #1 {
                          n157 = while {
                            tunnel: w277 -> [w287]
                            tunnel: [w282] -> w275
                            tunnel: w276 -> [w281]
                            stop <- w283 stop-if-true
                            n158 = local read "齿条扭矩(Nm)"() -> (w280:dbl)
                            n159 = Wait Until Next ms Multiple(millisecond multiple=u32 50 ("毫秒倍数")) -> ()  [unwired: 1 out]
                            n160 = Absolute Value(x=w280) -> (abs(x)=w285:dbl)
                            n161 = call <userlib>:"Acm_AxGetCmdVelocity.vi"("AxisHandle"=w287) -> ("Velocity"=w286:dbl, "AxisHandle"=w282:u32)  [unwired: 1 in, 2 out]
                            n162 = Equal To 0?(x=w286) -> (x = 0?=w284:bool)
                            n163 = Greater Or Equal?(x=w285, y=w281) -> (x >= y?=w278:bool)
                            n164 = Or(x=w278, y=w284) -> (x .or. y?=w283:bool)
                            n165 = Not(x=w278) -> (.not. x?=w279:bool)
                            n166 = local write "扭矩到达"(w278) -> ()
                            n167 = local write "旋转齿条轴使能"(w279) -> ()
                          }
                        }
                        frame #2 {
                          n168 = while {
                            tunnel: w289 -> [w293]
                            tunnel: [w290] -> _
                            stop <- w292 stop-if-true
                            n169 = call "PCI1220U停止.vi"("AxisHandle IN"=w293) -> ("完成"=w292:bool, "AxisHandle OUT"=w290:u32)  [unwired: 9 in]
                            n170 = Wait Until Next ms Multiple(millisecond multiple=u32 50 ("毫秒倍数")) -> ()  [unwired: 1 out]
                          }
                        }
                      }
                    }
                  }
                }
              }
              n171 = Wait Until Next ms Multiple(millisecond multiple=u32 50 ("毫秒倍数")) -> ()  [unwired: 1 out]
              n172 = local read "扭矩到达"() -> (w218:bool)
            }
            n173 = flat-sequence {
              tunnel: [w295] -> w217
              tunnel: w217 -> [w301]
              tunnel: [w301] -> w214
              tunnel: [w310] -> w215
              tunnel: w214 -> [w310]
              frame #0 {
                n174 = local write "电动缸速度(mm/s)"(6.0 ("电动缸速度(mm/s)")) -> ()
              }
              frame #1 {
                n175 = while {
                  tunnel: [w299] -> w295
                  stop <- w298 stop-if-true
                  n176 = local read "齿条左极限"() -> (w296:dbl)
                  n177 = local read "电动缸电机"() -> (w300:u32)
                  n178 = Wait Until Next ms Multiple(millisecond multiple=u32 50 ("毫秒倍数")) -> ()  [unwired: 1 out]
                  n179 = call "PCI1240电动缸位置模式 .vi"("Distance"=w296, "AxisHandle IN"=w300) -> ("AbsSuccess"=w298:bool, "AxisHandle OUT"=w299:u32)  [unwired: 8 in]
                }
              }
              frame #2 {
                n180 = while {
                  tunnel: w301 -> [w308]
                  stop <- w305 stop-if-true
                  n181 = local read "齿条推拉力(N)"() -> (w304:dbl)
                  n182 = call <userlib>:"Acm_AxGetCmdVelocity.vi"("AxisHandle"=w308) -> ("Velocity"=w309:dbl)  [unwired: 1 in, 3 out]
                  n183 = Wait Until Next ms Multiple(millisecond multiple=u32 50 ("毫秒倍数")) -> ()  [unwired: 1 out]
                  n184 = Less Or Equal?(x=w304, y=-1000.0) -> (x <= y?=w302:bool)
                  n185 = Equal To 0?(x=w309) -> (x = 0?=w306:bool)
                  n186 = Or(x=w306, y=w302) -> (x .or. y?=w305:bool)
                }
              }
              frame #3 {
                n187 = while {
                  tunnel: w310 -> [w314]
                  tunnel: [w311] -> _
                  stop <- w313 stop-if-true
                  n188 = call "PCI1220U停止.vi"("AxisHandle IN"=w314) -> ("完成"=w313:bool, "AxisHandle OUT"=w311:u32)  [unwired: 9 in]
                  n189 = Wait Until Next ms Multiple(millisecond multiple=u32 50 ("毫秒倍数")) -> ()  [unwired: 1 out]
                }
              }
            }
          }
          frame #2 {
            n190 = Wait (ms)(milliseconds to wait=u32 1000 ("等待时间（毫秒）")) -> ()  [unwired: 1 out]
          }
          frame #3 {
            n191 = Wait Until Next ms Multiple(millisecond multiple=u32 1000 ("毫秒倍数")) -> ()  [unwired: 1 out]
            n192 = local write "夹头夹紧"(TRUE ("夹头夹紧")) -> ()
            n193 = local write "夹头松开"(FALSE ("夹头松开")) -> ()
            n194 = while {
              stop <- "找帽OK" stop-if-true
              n195 = Wait Until Next ms Multiple(millisecond multiple=u32 50 ("毫秒倍数")) -> ()  [unwired: 1 out]
            }
          }
          frame #4 {
            n196 = disable-structure shown="禁用" {
              disable-tunnel: [w328 _] -> _
              frame Disabled {
                n197 = local read "齿条右极限"() -> (w326:dbl)
                n198 = local read "齿条左极限"() -> (w327:dbl)
                n199 = Add(x=w327, y=w326) -> (x+y=w330:dbl)
                n200 = Divide(x=w330, y=2.0) -> (x/y=w328:dbl)
              }
              frame Enabled {
              }
            }
            n201 = local write "电动缸速度(mm/s)"(15.0 ("电动缸轴移动速度")) -> ()
          }
          frame #5 {
            n202 = while {
              tunnel: w333 -> [w338]
              tunnel: w332 -> [w337]
              tunnel: [w334] -> w331
              stop <- w336 stop-if-true
              n203 = call "PCI1240电动缸位置模式 .vi"("Distance"=w337, "AxisHandle IN"=w338) -> ("AbsSuccess"=w336:bool, "AxisHandle OUT"=w334:u32)  [unwired: 8 in]
              n204 = Wait Until Next ms Multiple(millisecond multiple=u32 50 ("毫秒倍数")) -> ()  [unwired: 1 out]
            }
          }
          frame #6 {
            n205 = while {
              tunnel: w340 -> [w350]
              tunnel: [w341] -> w339
              stop <- w342 stop-if-true
              n206 = local read "齿条推拉力(N)"() -> (w347:dbl)
              n207 = call <userlib>:"Acm_AxGetCmdVelocity.vi"("AxisHandle"=w350) -> ("Velocity"=w349:dbl, "AxisHandle"=w341:u32)  [unwired: 1 in, 2 out]
              n208 = Wait Until Next ms Multiple(millisecond multiple=u32 50 ("毫秒倍数")) -> ()  [unwired: 1 out]
              n209 = Equal To 0?(x=w349) -> (x = 0?=w344:bool)
              n210 = Absolute Value(x=w347) -> (abs(x)=w346:dbl)
              n211 = Greater Or Equal?(x=w346, y=1000.0) -> (x >= y?=w343:bool)
              n212 = Or(x=w344, y=w343) -> (x .or. y?=w342:bool)
            }
          }
          frame #7 {
            n213 = while {
              tunnel: w351 -> [w355]
              tunnel: [w354] -> _
              stop <- w353 stop-if-true
              n214 = call "PCI1220U停止.vi"("AxisHandle IN"=w355) -> ("完成"=w353:bool, "AxisHandle OUT"=w354:u32)  [unwired: 9 in]
              n215 = Wait (ms)(milliseconds to wait=u32 50 ("毫秒倍数")) -> ()  [unwired: 1 out]
            }
          }
          frame #8 {
            n216 = local write "工步号"(u32 16 ("工步号")) -> ()
          }
        }
      }
      frame 16 {
        n217 = flat-sequence {
          tunnel: [w371] -> w368
          tunnel: w368 -> [w378]
          tunnel: [w377] -> w367
          tunnel: w367 -> [w389]
          tunnel: [w391] -> w366
          tunnel: w366 -> [w400]
          tunnel: [w399] -> w365
          tunnel: w365 -> [w412]
          tunnel: [w414] -> w364
          tunnel: w364 -> [w420]
          tunnel: [w420] -> w363
          tunnel: w363 -> [w430]
          tunnel: [w432] -> w362
          tunnel: w362 -> [w441]
          tunnel: [w440] -> w361
          tunnel: w361 -> [w453]
          tunnel: [w452] -> w360
          tunnel: [w451] -> w359
          tunnel: w360 -> [w458]
          tunnel: w359 -> [w457]
          tunnel: [w460] -> w358
          tunnel: w358 -> [w466]
          tunnel: [w466] -> w357
          tunnel: w357 -> [w477]
          frame #0 {
            n218 = local write "电动缸速度(mm/s)"(30.0 ("电动缸速度(mm/s)")) -> ()
          }
          frame #1 {
            n219 = Wait (ms)(milliseconds to wait=u32 100 ("等待时间（毫秒）")) -> ()  [unwired: 1 out]
          }
          frame #2 {
            n220 = while {
              tunnel: [w375] -> w371
              stop <- w374 stop-if-true
              n221 = local read "电动缸电机"() -> (w376:u32)
              n222 = local read "齿条左极限"() -> (w372:dbl)
              n223 = Wait Until Next ms Multiple(millisecond multiple=u32 50 ("毫秒倍数")) -> ()  [unwired: 1 out]
              n224 = call "PCI1240电动缸位置模式 .vi"("Distance"=w372, "AxisHandle IN"=w376) -> ("AbsSuccess"=w374:bool, "AxisHandle OUT"=w375:u32)  [unwired: 8 in]
            }
          }
          frame #3 {
            n225 = while {
              tunnel: w378 -> [w386]
              tunnel: [w380] -> w377
              stop <- w383 stop-if-true
              n226 = local read "齿条推拉力(N)"() -> (w379:dbl)
              n227 = Wait Until Next ms Multiple(millisecond multiple=u32 50 ("毫秒倍数")) -> ()  [unwired: 1 out]
              n228 = call <userlib>:"Acm_AxGetCmdVelocity.vi"("AxisHandle"=w386) -> ("Velocity"=w387:dbl, "AxisHandle"=w380:u32)  [unwired: 1 in, 2 out]
              n229 = Less Or Equal?(x=w379, y=-500.0) -> (x <= y?=w381:bool)
              n230 = Equal To 0?(x=w387) -> (x = 0?=w384:bool)
              n231 = Or(x=w384, y=w381) -> (x .or. y?=w383:bool)
            }
          }
          frame #4 {
            n232 = call "PCI1220U停止.vi"("AxisHandle IN"=w389) -> ()  [unwired: 9 in, 2 out]
            n233 = local write "电动缸速度(mm/s)"(1.0 ("电动缸速度(mm/s)")) -> ()
          }
          frame #5 {
            n234 = Wait (ms)(milliseconds to wait=u32 100 ("等待时间（毫秒）")) -> ()  [unwired: 1 out]
          }
          frame #6 {
            n235 = while {
              tunnel: [w397] -> w391
              stop <- w396 stop-if-true
              n236 = local read "齿条左极限"() -> (w394:dbl)
              n237 = Wait Until Next ms Multiple(millisecond multiple=u32 50 ("毫秒倍数")) -> ()  [unwired: 1 out]
              n238 = local read "电动缸电机"() -> (w398:u32)
              n239 = Add(x=w394, y=30.0) -> (x+y=w393:dbl)
              n240 = call "PCI1240电动缸位置模式 .vi"("Distance"=w393, "AxisHandle IN"=w398) -> ("AbsSuccess"=w396:bool, "AxisHandle OUT"=w397:u32)  [unwired: 8 in]
            }
          }
          frame #7 {
            n241 = while {
              tunnel: w400 -> [w408]
              tunnel: [w402] -> w399
              stop <- w405 stop-if-true
              n242 = local read "齿条推拉力(N)"() -> (w401:dbl)
              n243 = Wait Until Next ms Multiple(millisecond multiple=u32 50 ("毫秒倍数")) -> ()  [unwired: 1 out]
              n244 = call <userlib>:"Acm_AxGetCmdVelocity.vi"("AxisHandle"=w408) -> ("Velocity"=w409:dbl, "AxisHandle"=w402:u32)  [unwired: 1 in, 2 out]
              n245 = Less Or Equal?(x=w401, y=-500.0) -> (x <= y?=w403:bool)
              n246 = Equal To 0?(x=w409) -> (x = 0?=w406:bool)
              n247 = Or(x=w406, y=w403) -> (x .or. y?=w405:bool)
            }
          }
          frame #8 {
            n248 = local read "电动缸位置(mm)"() -> (→"齿条跑和左极限":dbl)
            n249 = call "PCI1220U停止.vi"("AxisHandle IN"=w412) -> ()  [unwired: 9 in, 2 out]
            n250 = local write "电动缸速度(mm/s)"(30.0 ("电动缸速度(mm/s)")) -> ()
          }
          frame #9 {
            n251 = Wait (ms)(milliseconds to wait=u32 100 ("等待时间（毫秒）")) -> ()  [unwired: 1 out]
          }
          frame #10 {
            n252 = while {
              tunnel: [w418] -> w414
              stop <- w417 stop-if-true
              n253 = local read "电动缸电机"() -> (w419:u32)
              n254 = local read "齿条右极限"() -> (w415:dbl)
              n255 = Wait Until Next ms Multiple(millisecond multiple=u32 50 ("毫秒倍数")) -> ()  [unwired: 1 out]
              n256 = call "PCI1240电动缸位置模式 .vi"("Distance"=w415, "AxisHandle IN"=w419) -> ("AbsSuccess"=w417:bool, "AxisHandle OUT"=w418:u32)  [unwired: 8 in]
            }
          }
          frame #11 {
            n257 = while {
              tunnel: w420 -> [w427]
              stop <- w424 stop-if-true
              n258 = local read "齿条推拉力(N)"() -> (w421:dbl)
              n259 = Wait Until Next ms Multiple(millisecond multiple=u32 50 ("毫秒倍数")) -> ()  [unwired: 1 out]
              n260 = call <userlib>:"Acm_AxGetCmdVelocity.vi"("AxisHandle"=w427) -> ("Velocity"=w428:dbl)  [unwired: 1 in, 3 out]
              n261 = Equal To 0?(x=w428) -> (x = 0?=w425:bool)
              n262 = Greater Or Equal?(x=w421, y=500.0) -> (x >= y?=w422:bool)
              n263 = Or(x=w425, y=w422) -> (x .or. y?=w424:bool)
            }
          }
          frame #12 {
            n264 = call "PCI1220U停止.vi"("AxisHandle IN"=w430) -> ()  [unwired: 9 in, 2 out]
            n265 = local write "电动缸速度(mm/s)"(1.0 ("电动缸速度(mm/s)")) -> ()
          }
          frame #13 {
            n266 = Wait (ms)(milliseconds to wait=u32 100 ("毫秒倍数")) -> ()  [unwired: 1 out]
          }
          frame #14 {
            n267 = while {
              tunnel: [w438] -> w432
              stop <- w437 stop-if-true
              n268 = local read "齿条右极限"() -> (w435:dbl)
              n269 = Wait Until Next ms Multiple(millisecond multiple=u32 50 ("毫秒倍数")) -> ()  [unwired: 1 out]
              n270 = local read "电动缸电机"() -> (w439:u32)
              n271 = Subtract(x=w435, y=30.0) -> (x-y=w433:dbl)
              n272 = call "PCI1240电动缸位置模式 .vi"("Distance"=w433, "AxisHandle IN"=w439) -> ("AbsSuccess"=w437:bool, "AxisHandle OUT"=w438:u32)  [unwired: 8 in]
            }
          }
          frame #15 {
            n273 = while {
              tunnel: w441 -> [w443]
              tunnel: [w442] -> w440
              stop <- w447 stop-if-true
              n274 = local read "齿条推拉力(N)"() -> (w444:dbl)
              n275 = Wait Until Next ms Multiple(millisecond multiple=u32 50 ("毫秒倍数")) -> ()  [unwired: 1 out]
              n276 = call <userlib>:"Acm_AxGetCmdVelocity.vi"("AxisHandle"=w443) -> ("Velocity"=w450:dbl, "AxisHandle"=w442:u32)  [unwired: 1 in, 2 out]
              n277 = Equal To 0?(x=w450) -> (x = 0?=w448:bool)
              n278 = Greater Or Equal?(x=w444, y=500.0) -> (x >= y?=w445:bool)
              n279 = Or(x=w448, y=w445) -> (x .or. y?=w447:bool)
            }
          }
          frame #16 {
            n280 = local read "电动缸位置(mm)"() -> (w451:dbl)
            "齿条跑和右极限" <- w451
            n281 = call "PCI1220U停止.vi"("AxisHandle IN"=w453) -> ()  [unwired: 9 in, 2 out]
            n282 = local read "齿条跑和左极限"() -> (w452:dbl)
          }
          frame #17 {
            n283 = Add(x=w458, y=w457) -> (x+y=w456:dbl)
            n284 = Divide(x=w456, y=2.0) -> (x/y=w454:dbl)
            n285 = local write "转向器中心"(w454) -> ()
          }
          frame #18 {
            n286 = Wait (ms)(milliseconds to wait=u32 100 ("等待时间（毫秒）")) -> ()  [unwired: 1 out]
          }
          frame #19 {
            n287 = while {
              tunnel: [w464] -> w460
              stop <- w463 stop-if-true
              n288 = local read "电动缸电机"() -> (w465:u32)
              n289 = local read "转向器中心"() -> (w461:dbl)
              n290 = Wait Until Next ms Multiple(millisecond multiple=u32 50 ("毫秒倍数")) -> ()  [unwired: 1 out]
              n291 = call "PCI1240电动缸位置模式 .vi"("Distance"=w461, "AxisHandle IN"=w465) -> ("AbsSuccess"=w463:bool, "AxisHandle OUT"=w464:u32)  [unwired: 8 in]
            }
          }
          frame #20 {
            n292 = while {
              tunnel: w466 -> [w474]
              stop <- w471 stop-if-true
              n293 = local read "齿条推拉力(N)"() -> (w470:dbl)
              n294 = Wait Until Next ms Multiple(millisecond multiple=u32 50 ("毫秒倍数")) -> ()  [unwired: 1 out]
              n295 = call <userlib>:"Acm_AxGetCmdVelocity.vi"("AxisHandle"=w474) -> ("Velocity"=w475:dbl)  [unwired: 1 in, 3 out]
              n296 = Absolute Value(x=w470) -> (abs(x)=w469:dbl)
              n297 = Equal To 0?(x=w475) -> (x = 0?=w472:bool)
              n298 = Greater Or Equal?(x=w469, y=500.0) -> (x >= y?=w467:bool)
              n299 = Or(x=w472, y=w467) -> (x .or. y?=w471:bool)
            }
          }
          frame #21 {
            n300 = call "PCI1220U停止.vi"("AxisHandle IN"=w477) -> ()  [unwired: 9 in, 2 out]
            n301 = local write "电动缸速度(mm/s)"(30.0 ("电动缸速度(mm/s)")) -> ()
          }
          frame #22 {
            n302 = Wait (ms)(milliseconds to wait=u32 150 ("等待时间（毫秒）")) -> ()  [unwired: 1 out]
          }
          frame #23 {
            n303 = local write "工步号"(u32 20 ("工步号")) -> ()
          }
        }
      }
      frame 20 {
        n304 = flat-sequence {
          tunnel: [w509] -> w490
          tunnel: w490 -> [w515]
          tunnel: [w521] -> w482
          tunnel: w482 -> [w528]
          tunnel: [w528] -> w481
          tunnel: w481 -> [w536]
          tunnel: [w536] -> w480
          tunnel: w480 -> [w537]
          tunnel: [w537] -> w489
          tunnel: w489 -> [w546]
          tunnel: [w552] -> w487
          tunnel: [w554] -> w488
          tunnel: w487 -> [w554]
          tunnel: [w556] -> w483
          tunnel: w488 -> [w556]
          tunnel: w483 -> [w563]
          tunnel: [w562] -> w494
          tunnel: [w567] -> w493
          tunnel: [w566] -> w492
          tunnel: w494 -> [w565]
          tunnel: [w565] -> w491
          tunnel: [w594] -> w497
          tunnel: [w591] -> w496
          tunnel: w493 -> [w591]
          tunnel: [w590] -> w495
          tunnel: w492 -> [w590]
          tunnel: w491 -> [w594]
          tunnel: w497 -> [w598]
          tunnel: [w597] -> w486
          tunnel: w496 -> [w595]
          tunnel: w495 -> [w596]
          tunnel: w486 -> [w604]
          tunnel: [w603] -> w485
          tunnel: w485 -> [w611]
          tunnel: [w610] -> w484
          tunnel: w484 -> [w620]
          frame #0 {
            n305 = while {
              stop <- w500 stop-if-true
              n306 = local read "夹头松开"() -> (w501:bool)
              n307 = local read "夹头夹紧位"() -> (w499:bool)
              n308 = Wait Until Next ms Multiple(millisecond multiple=u32 50 ("毫秒倍数")) -> ()  [unwired: 1 out]
              n309 = Not(x=w501) -> (.not. x?=w498:bool)
              n310 = And(x=w499, y=w498) -> (x .and. y?=w500:bool)
            }
          }
          frame #1 {
            n311 = local write "测头机构轴速度(mm/s)"(30.0 ("测头机构轴速度(mm/s)")) -> ()
            n312 = local write "选项卡控件"(T1."间隙测量" ("选项卡控件")) -> ()
          }
          frame #2 {
            n313 = local read "转向器中心"() -> (w507:dbl)
            n314 = local read "电动缸电机"() -> (w508:u32)
            n315 = Add(x=w507, y=0.0) -> (x+y=w506:dbl)
            n316 = while {
              tunnel: w508 -> [w514]
              tunnel: w506 -> [w513]
              tunnel: [w510] -> w509
              stop <- w512 stop-if-true
              n317 = call "PCI1240电动缸位置模式 .vi"("Distance"=w513, "AxisHandle IN"=w514) -> ("AbsSuccess"=w512:bool, "AxisHandle OUT"=w510:u32)  [unwired: 8 in]
              n318 = Wait Until Next ms Multiple(millisecond multiple=u32 50 ("毫秒倍数")) -> ()  [unwired: 1 out]
            }
          }
          frame #3 {
            n319 = while {
              tunnel: w515 -> [w519]
              stop <- w517 stop-if-true
              n320 = call <userlib>:"Acm_AxGetCmdVelocity.vi"("AxisHandle"=w519) -> ("Velocity"=w518:dbl)  [unwired: 1 in, 3 out]
              n321 = Wait Until Next ms Multiple(millisecond multiple=u32 50 ("毫秒倍数")) -> ()  [unwired: 1 out]
              n322 = Equal To 0?(x=w518) -> (x = 0?=w517:bool)
            }
          }
          frame #4 {
            n323 = local read "测头机构电机"() -> (w522:u32)
            n324 = local read "测头机构轴检测位"() -> (w520:dbl)
            n325 = while {
              tunnel: w522 -> [w525]
              tunnel: w520 -> [w524]
              tunnel: [w523] -> w521
              stop <- w527 stop-if-true
              n326 = Wait Until Next ms Multiple(millisecond multiple=u32 50 ("毫秒倍数")) -> ()  [unwired: 1 out]
              n327 = call "PCI1220U进给轴位置模式.vi"("Distance"=w524, "AxisHandle IN"=w525) -> ("AbsSuccess"=w527:bool, "AxisHandle OUT"=w523:u32)  [unwired: 8 in]
            }
          }
          frame #5 {
            n328 = while {
              stop <- w529 stop-if-true
              n329 = local read "测头机构轴检测位"() -> (w533:dbl)
              n330 = local read "测头机构轴位置(mm)"() -> (w532:dbl)
              n331 = Wait Until Next ms Multiple(millisecond multiple=u32 50 ("毫秒倍数")) -> ()  [unwired: 1 out]
              n332 = Subtract(x=w533, y=10.0) -> (x-y=w530:dbl)
              n333 = Greater Or Equal?(x=w532, y=w530) -> (x >= y?=w529:bool)
            }
          }
          frame #6 {
            n334 = local write "测头机构轴速度(mm/s)"(10.0 ("测头机构轴速度(mm/s)")) -> ()
          }
          frame #7 {
            n335 = while {
              tunnel: w537 -> [w545]
              stop <- w539 stop-if-true
              n336 = local read "间隙位移(mm)"() -> (w542:dbl)
              n337 = call <userlib>:"Acm_AxGetCmdVelocity.vi"("AxisHandle"=w545) -> ("Velocity"=w544:dbl)  [unwired: 1 in, 3 out]
              n338 = Wait Until Next ms Multiple(millisecond multiple=u32 50 ("毫秒倍数")) -> ()  [unwired: 1 out]
              n339 = Equal To 0?(x=w544) -> (x = 0?=w540:bool)
              n340 = Greater Or Equal?(x=w542, y=4.5) -> (x >= y?=w538:bool)
              n341 = Or(x=w540, y=w538) -> (x .or. y?=w539:bool)
            }
          }
          frame #8 {
            n342 = while {
              tunnel: w546 -> [w550]
              tunnel: [w549] -> _
              stop <- w548 stop-if-true
              n343 = call "PCI1220U停止.vi"("AxisHandle IN"=w550) -> ("完成"=w548:bool, "AxisHandle OUT"=w549:u32)  [unwired: 9 in]
              n344 = Wait (ms)(milliseconds to wait=u32 50 ("毫秒倍数")) -> ()  [unwired: 1 out]
            }
          }
          frame #9 {
            n345 = local write "旋转齿条轴使能"(TRUE ("旋转齿条轴使能")) -> ()
          }
          frame #10 {
            n346 = local read "旋转齿条电机"() -> (w552:u32)
            n347 = call "PCI1220U角度置零.vi"("AxisHandle IN"=w552) -> ()  [unwired: 10 in, 1 out]
          }
          frame #11 {
            n348 = local write "旋转伺服速度(°/s)"(1.0 ("旋转齿条轴速度(°/s)")) -> ()
            n349 = Wait (ms)(milliseconds to wait=u32 1000 ("毫秒倍数")) -> ()  [unwired: 1 out]
          }
          frame #12 {
            n350 = while {
              i -> [w560]
              stop <- w557 stop-if-true
              n351 = local read "间隙位移(mm)"() -> (w561:dbl)
              n352 = Wait Until Next ms Multiple(millisecond multiple=u32 50 ("毫秒倍数")) -> ()  [unwired: 1 out]
              n353 = Greater Or Equal?(x=w560, y=40) -> (x >= y?=w557:bool)
              n354 = local write "基准位移"(w561) -> ()
            }
          }
          frame #13 {
            n355 = call "PCI1220U运行.vi"("方向"=enum32{"Negative", "Positive"}."Negative" ("Direction"), "AxisHandle IN"=w563) -> ("AxisHandle OUT"=w562:u32)  [unwired: 9 in]
          }
          frame #14 {
            w568 = dbl[] []
            n356 = while {
              shift-right: [w579] -> w567
              shift-left: w568 -> [w581]
              shift-right: [w578] -> w566
              shift-left: w568 -> [w580]
              stop <- w571 stop-if-true
              n357 = Wait (ms)(milliseconds to wait=u32 10 ("毫秒倍数")) -> ()  [unwired: 1 out]
              n358 = local read "间隙位移(mm)"() -> (w574:dbl)
              n359 = local read "基准位移"() -> (w572:dbl)
              n360 = local read "齿条扭矩(Nm)"() -> (w575:dbl)
              n361 = Subtract(x=w574, y=w572) -> (x-y=w573:dbl)
              n362 = Absolute Value(x=w575) -> (abs(x)=w570:dbl)
              n363 = Build Array (concatenate) "创建数组"(w580, w573) -> (w578:dbl[])
              n364 = Build Array (concatenate) ("创建数组")(w581, w570) -> (w579:dbl[])
              n365 = Greater Or Equal?(x=w570, y="扭矩停止值") -> (x >= y?=w571:bool)
              n366 = Bundle ("捆绑")(w579, w578) -> (w576:cluster{dbl[], dbl[]})  [unwired: 1 in]
              n367 = Build Array ("创建数组")(w576) -> (w577:cluster{dbl[], dbl[]}[])
              n368 = local write "扭动曲线"(w577) -> ()
            }
          }
          frame #15 {
            n369 = Absolute Value(x=w591) -> (abs(x)=w592:dbl[])
            n370 = local read "测量点扭矩"() -> (w593:dbl)
            n371 = local read "基准位移"() -> (w587:dbl)
            n372 = call "自定义插值.vi"("压力"=w593, "扭矩数组"=w592, "位移数组"=w590) -> ("扭矩值"=w588:dbl)  [unwired: 8 in]
            n373 = Array Max & Min(array=w590) -> (min value=w589:dbl)  [unwired: 3 out]
            n374 = Absolute Value(x=w589) -> (abs(x)=w586:dbl)
            n375 = Subtract(x=w587, y=w586) -> (x-y=w585:dbl)
            n376 = Add(x=w588, y=w586) -> (x+y=w584:dbl)
            n377 = Absolute Value(x=w584) -> (abs(x)=w583:dbl)
            n378 = local write "基准位移"(w585) -> ()
            n379 = local write "中间位置间隙"(w583) -> ()
          }
          frame #16 {
            n380 = while {
              tunnel: w598 -> [w602]
              tunnel: [w601] -> w597
              stop <- w600 stop-if-true
              n381 = call "PCI1220U停止.vi"("AxisHandle IN"=w602) -> ("完成"=w600:bool, "AxisHandle OUT"=w601:u32)  [unwired: 9 in]
              n382 = Wait (ms)(milliseconds to wait=u32 50 ("毫秒倍数")) -> ()  [unwired: 1 out]
            }
            "间隙Y数组" <- w596
            "间隙X数组" <- w595
          }
          frame #17 {
            n383 = while {
              tunnel: [w609] -> w603
              tunnel: w604 -> [w606]
              stop <- w608 stop-if-true
              n384 = Wait Until Next ms Multiple(millisecond multiple=u32 50 ("毫秒倍数")) -> ()  [unwired: 1 out]
              n385 = call "PCI1220U扭矩轴位置模式.vi"("Distance"=0.0, "AxisHandle IN"=w606) -> ("AbsSuccess"=w608:bool, "AxisHandle OUT"=w609:u32)  [unwired: 8 in]
            }
          }
          frame #18 {
            n386 = while {
              tunnel: w611 -> [w613]
              tunnel: [w613] -> w610
              stop <- w616 stop-if-true
              n387 = local read "齿条扭矩(Nm)"() -> (w612:dbl)
              n388 = call <userlib>:"Acm_AxGetCmdVelocity.vi"("AxisHandle"=w613) -> ("Velocity"=w619:dbl)  [unwired: 1 in, 3 out]
              n389 = Wait Until Next ms Multiple(millisecond multiple=u32 50 ("毫秒倍数")) -> ()  [unwired: 1 out]
              n390 = Equal To 0?(x=w619) -> (x = 0?=w617:bool)
              n391 = Greater Or Equal?(x=w612, y=3.0) -> (x >= y?=w614:bool)
              n392 = Or(x=w617, y=w614) -> (x .or. y?=w616:bool)
            }
          }
          frame #19 {
            n393 = while {
              tunnel: w620 -> [w624]
              tunnel: [w623] -> _
              stop <- w622 stop-if-true
              n394 = call "PCI1220U停止.vi"("AxisHandle IN"=w624) -> ("完成"=w622:bool, "AxisHandle OUT"=w623:u32)  [unwired: 9 in]
              n395 = Wait (ms)(milliseconds to wait=u32 50 ("毫秒倍数")) -> ()  [unwired: 1 out]
            }
          }
          frame #20 {
            n396 = local write "旋转齿条轴使能"(FALSE ("旋转齿条轴使能")) -> ()
            n397 = Wait (ms)(milliseconds to wait=u32 500 ("毫秒倍数")) -> ()  [unwired: 1 out]
          }
          frame #21 {
            n398 = local write "工步号"(u32 25 ("工步号")) -> ()
          }
        }
      }
      frame 25 {
        n399 = flat-sequence {
          frame #0 {
            n400 = local read "中间间隙标准(mm)"() -> (w629:dbl)
            n401 = local read "最小间隙(mm)"() -> (w628:dbl)
            n402 = local read "中间位置间隙"() -> (w630:dbl)
            n403 = In Range and Coerce(upper limit=w629, x=w630, lower limit=w628) -> (In Range?=w633:bool)  [unwired: 1 out]
            n404 = case shown="假" w633 {
              tunnel: [FALSE ("本序合格") TRUE ("本序合格")] -> w632
              tunnel: [w638 0.0 ("需调整角度(度)")] -> w631
              tunnel: w630 -> [w636 _]
              tunnel: w629 -> [w635 _]
              tunnel: w628 -> [w634 _]
              frame False {
                n405 = xnode "公式"("X"=w636, "Xmax"=w635, "Xmin"=w634) -> ("结果"=w638:dbl)  [unwired: 1 in, 1 out]
              }
              frame True {
              }
            }
            n406 = local write "单点间隙合格"(w632) -> ()
            n407 = local write "需调整角度(度)"(w631) -> ()
          }
          frame #1 {
            n408 = local read "单点间隙合格"() -> (w653:bool)
            n409 = case shown="假" w653 {
              frame False {
                n410 = local read "已调试次数"() -> (w656:dbl)
                n411 = Less?(x=w656, y="设定间隙调整次数") -> (x < y?=w655:bool)
                n412 = case shown="真" w655 {
                  frame False {
                    n413 = local write "工步号"(u32 45 ("变更工步号")) -> ()
                  }
                  frame True {
                    n414 = local write "工步号"(u32 30 ("变更工步号")) -> ()
                  }
                }
              }
              frame True {
                n415 = local write "工步号"(u32 40 ("变更工步号")) -> ()
              }
            }
          }
        }
      }
      frame 30 {
        # "人工调整"
        n416 = flat-sequence {
          tunnel: [w662] -> w660
          tunnel: w660 -> [w669]
          frame #0 {
            n417 = local write "测头机构轴速度(mm/s)"(30.0 ("测头机构轴速度(mm/s)")) -> ()
          }
          frame #1 {
            n418 = local read "测头机构电机"() -> (w663:u32)
            n419 = while {
              tunnel: w663 -> [w666]
              tunnel: [w665] -> w662
              stop <- w668 stop-if-true
              n420 = local read "测头机构轴待检位"() -> (w664:dbl)
              n421 = call "PCI1220U进给轴位置模式.vi"("Distance"=w664, "AxisHandle IN"=w666) -> ("AbsSuccess"=w668:bool, "AxisHandle OUT"=w665:u32)  [unwired: 8 in]
              n422 = Wait Until Next ms Multiple(millisecond multiple=u32 50 ("毫秒倍数")) -> ()  [unwired: 1 out]
            }
          }
          frame #2 {
            n423 = while {
              tunnel: w669 -> [w673]
              stop <- w671 stop-if-true
              n424 = call <userlib>:"Acm_AxGetCmdVelocity.vi"("AxisHandle"=w673) -> ("Velocity"=w672:dbl)  [unwired: 1 in, 3 out]
              n425 = Wait Until Next ms Multiple(millisecond multiple=u32 50 ("毫秒倍数")) -> ()  [unwired: 1 out]
              n426 = Equal To 0?(x=w672) -> (x = 0?=w671:bool)
            }
          }
          frame #3 {
            n427 = while {
              stop <- w675 stop-if-true
              n428 = local read "测头机构轴位置(mm)"() -> (w677:dbl)
              n429 = Wait Until Next ms Multiple(millisecond multiple=u32 50 ("毫秒倍数")) -> ()  [unwired: 1 out]
              n430 = Less Or Equal?(x=w677, y=35.0) -> (x <= y?=w675:bool)
            }
          }
          frame #4 {
            n431 = local write "测头气缸左移"(TRUE ("测头气缸左移")) -> ()
            n432 = local write "测头气缸右移"(FALSE ("测头气缸右移")) -> ()
          }
          frame #5 {
            n433 = while {
              stop <- w680 stop-if-true
              # "等待启动"
              n434 = local read "间隙启动"() -> (w680:bool)
              n435 = Wait Until Next ms Multiple(millisecond multiple=u32 50 ("毫秒倍数")) -> ()  [unwired: 1 out]
            }
          }
          frame #6 {
            n436 = local read "不合格品"() -> (w682:bool)
            n437 = case shown="假" w682 {
              frame False {
                n438 = flat-sequence {
                  frame #0 {
                    n439 = local read "已调试次数"() -> (w685:dbl)
                    n440 = local write "测头气缸左移"(FALSE ("测头气缸左移")) -> ()
                    n441 = local write "测头气缸右移"(TRUE ("测头气缸左移")) -> ()
                    n442 = Add(x=w685, y=1.0 ("已调试次数")) -> (x+y=w687:dbl)
                    n443 = local write "已调试次数"(w687) -> ()
                  }
                  frame #1 {
                    n444 = while {
                      stop <- w688 stop-if-true
                      n445 = Wait Until Next ms Multiple(millisecond multiple=u32 50 ("毫秒倍数")) -> ()  [unwired: 1 out]
                      n446 = local read "测头右位"() -> (w688:bool)
                    }
                  }
                  frame #2 {
                    n447 = local write "工步号"(u32 20 ("工步号")) -> ()
                  }
                }
              }
              frame True {
                n448 = local write "工步号"(u32 45 ("工步号")) -> ()
              }
            }
          }
        }
      }
      frame 40 {
        n449 = flat-sequence {
          tunnel: [w816] -> w812
          tunnel: w812 -> [w818]
          tunnel: [w817] -> w811
          tunnel: w811 -> [w826]
          tunnel: [w826] -> w810
          tunnel: w810 -> [w838]
          tunnel: [w838] -> w809
          tunnel: w809 -> [w839]
          tunnel: [w840] -> w808
          tunnel: w808 -> [w848]
          tunnel: [w848] -> w807
          tunnel: w807 -> [w858]
          tunnel: [w858] -> w806
          tunnel: w806 -> [w866]
          tunnel: [w866] -> w805
          tunnel: w805 -> [w868]
          tunnel: [w869] -> w804
          tunnel: [w867] -> w803
          tunnel: w804 -> [w880]
          tunnel: w803 -> [w881]
          tunnel: [w881] -> w802
          tunnel: [w879] -> w801
          tunnel: [w878] -> w800
          tunnel: [w877] -> w799
          tunnel: w802 -> [w921]
          tunnel: [w921] -> w798
          tunnel: [w920] -> w797
          tunnel: w801 -> [w920]
          tunnel: [w919] -> w796
          tunnel: w800 -> [w919]
          tunnel: [w918] -> w795
          tunnel: w799 -> [w918]
          tunnel: w798 -> [w923]
          tunnel: [w922] -> w794
          tunnel: [w926] -> w793
          tunnel: w797 -> [w926]
          tunnel: [w925] -> w792
          tunnel: w796 -> [w925]
          tunnel: [w924] -> w791
          tunnel: w795 -> [w924]
          tunnel: [w941] -> w787
          tunnel: [w940] -> w788
          tunnel: [w939] -> w790
          tunnel: w794 -> [w934]
          tunnel: w793 -> [w938]
          tunnel: w792 -> [w937]
          tunnel: w791 -> [w936]
          tunnel: [w934] -> w789
          tunnel: [w995] -> w786
          tunnel: [w979] -> w785
          tunnel: [w977] -> w784
          tunnel: [w993] -> w783
          tunnel: [w992] -> w782
          tunnel: [w991] -> w781
          tunnel: [w990] -> w780
          tunnel: [w983] -> w779
          tunnel: [w982] -> w778
          tunnel: w790 -> [w993]
          tunnel: w789 -> [w994]
          tunnel: w788 -> [w979]
          tunnel: w787 -> [w995]
          tunnel: w786 -> [w1018]
          tunnel: [w1018] -> w777
          tunnel: w785 -> [w1017]
          tunnel: [w1017] -> w776
          tunnel: w784 -> [w1016]
          tunnel: [w1016] -> w775
          tunnel: [w1002] -> w774
          tunnel: [w1015] -> w773
          tunnel: w783 -> [w1015]
          tunnel: w782 -> [w1012]
          tunnel: w781 -> [w1014]
          tunnel: w780 -> [w1013]
          tunnel: [w1006] -> w772
          tunnel: [w1005] -> w771
          tunnel: w779 -> [w1004]
          tunnel: [w1004] -> w770
          tunnel: [w1003] -> w769
          tunnel: w778 -> [w1003]
          tunnel: w777 -> [w1034]
          tunnel: w776 -> [w1033]
          tunnel: w775 -> [w1025]
          tunnel: w774 -> [w1029]
          tunnel: w773 -> [w1032]
          tunnel: w772 -> [w1036]
          tunnel: [w1036] -> w768
          tunnel: w771 -> [w1035]
          tunnel: [w1035] -> w767
          tunnel: [w1031] -> w766
          tunnel: [w1030] -> w765
          tunnel: [w1028] -> w764
          tunnel: w770 -> [w1027]
          tunnel: [w1027] -> w763
          tunnel: [w1026] -> w762
          tunnel: w769 -> [w1026]
          tunnel: [w1025] -> w761
          tunnel: w768 -> [w1081]
          tunnel: [w1081] -> w760
          tunnel: w767 -> [w1080]
          tunnel: [w1080] -> w759
          tunnel: [w1074] -> w758
          tunnel: [w1079] -> w757
          tunnel: w766 -> [w1079]
          tunnel: [w1078] -> w756
          tunnel: w765 -> [w1078]
          tunnel: [w1077] -> w755
          tunnel: w764 -> [w1077]
          tunnel: w763 -> [w1076]
          tunnel: [w1076] -> w754
          tunnel: [w1075] -> w753
          tunnel: w762 -> [w1075]
          tunnel: w761 -> [w1074]
          tunnel: w760 -> [w1090]
          tunnel: [w1090] -> w752
          tunnel: w759 -> [w1089]
          tunnel: [w1089] -> w751
          tunnel: w758 -> [w1082]
          tunnel: [w1088] -> w750
          tunnel: w757 -> [w1088]
          tunnel: [w1087] -> w749
          tunnel: w756 -> [w1087]
          tunnel: [w1082] -> w748
          tunnel: [w1083] -> w747
          tunnel: [w1086] -> w746
          tunnel: w755 -> [w1086]
          tunnel: w754 -> [w1085]
          tunnel: [w1085] -> w745
          tunnel: [w1084] -> w744
          tunnel: w753 -> [w1084]
          tunnel: [w1108] -> w743
          tunnel: [w1107] -> w742
          tunnel: [w1106] -> w741
          tunnel: w752 -> [w1105]
          tunnel: w751 -> [w1104]
          tunnel: [w1105] -> w740
          tunnel: [w1104] -> w739
          tunnel: w750 -> [w1103]
          tunnel: w749 -> [w1102]
          tunnel: w748 -> [w1097]
          tunnel: w747 -> [w1101]
          tunnel: w746 -> [w1100]
          tunnel: w745 -> [w1099]
          tunnel: [w1099] -> w738
          tunnel: [w1098] -> w737
          tunnel: w744 -> [w1098]
          tunnel: [w1097] -> w736
          tunnel: w743 -> [w1151]
          tunnel: w742 -> [w1157]
          tunnel: [w1157] -> w735
          tunnel: [w1145] -> w734
          tunnel: w741 -> [w1156]
          tunnel: [w1156] -> w733
          tunnel: [w1153] -> w732
          tunnel: [w1152] -> w731
          tunnel: [w1151] -> w730
          tunnel: w740 -> [w1150]
          tunnel: w739 -> [w1149]
          tunnel: [w1150] -> w729
          tunnel: [w1149] -> w728
          tunnel: w738 -> [w1148]
          tunnel: [w1148] -> w727
          tunnel: [w1147] -> w726
          tunnel: w737 -> [w1147]
          tunnel: [w1146] -> w725
          tunnel: w736 -> [w1145]
          tunnel: w735 -> [w1166]
          tunnel: [w1209] -> w724
          tunnel: w734 -> [w1209]
          tunnel: w733 -> [w1208]
          tunnel: [w1207] -> w723
          tunnel: w732 -> [w1206]
          tunnel: w731 -> [w1205]
          tunnel: w730 -> [w1189]
          tunnel: [w1197] -> w722
          tunnel: [w1196] -> w721
          tunnel: [w1195] -> w720
          tunnel: w729 -> [w1195]
          tunnel: [w1194] -> w719
          tunnel: w728 -> [w1194]
          tunnel: [w1193] -> w718
          tunnel: [w1192] -> w717
          tunnel: [w1176] -> w716
          tunnel: [w1177] -> w715
          tunnel: [w1175] -> w714
          tunnel: [w1174] -> w713
          tunnel: w727 -> [w1172]
          tunnel: [w1172] -> w712
          tunnel: [w1171] -> w711
          tunnel: w726 -> [w1171]
          tunnel: [w1165] -> w710
          tunnel: w725 -> [w1164]
          tunnel: w724 -> [w1234]
          tunnel: [w1234] -> w709
          tunnel: [w1231] -> w708
          tunnel: w723 -> [w1233]
          tunnel: w722 -> [w1229]
          tunnel: [w1218] -> w707
          tunnel: [w1227] -> w706
          tunnel: w721 -> [w1226]
          tunnel: [w1222] -> w705
          tunnel: w720 -> [w1222]
          tunnel: [w1221] -> w704
          tunnel: w719 -> [w1221]
          tunnel: [w1220] -> w703
          tunnel: w718 -> [w1220]
          tunnel: [w1219] -> w702
          tunnel: w717 -> [w1219]
          tunnel: [w1217] -> w701
          tunnel: w716 -> [w1217]
          tunnel: [w1216] -> w700
          tunnel: w715 -> [w1216]
          tunnel: w714 -> [w1215]
          tunnel: [w1215] -> w699
          tunnel: w713 -> [w1214]
          tunnel: [w1214] -> w698
          tunnel: w712 -> [w1213]
          tunnel: [w1213] -> w697
          tunnel: [w1212] -> w696
          tunnel: w711 -> [w1212]
          tunnel: w710 -> [w1211]
          tunnel: w709 -> [w1250]
          tunnel: [w1250] -> w695
          tunnel: w708 -> [w1249]
          tunnel: [w1249] -> w694
          tunnel: w707 -> [w1245]
          tunnel: w706 -> [w1241]
          tunnel: w705 -> [w1244]
          tunnel: w704 -> [w1243]
          tunnel: w703 -> [w1247]
          tunnel: w702 -> [w1246]
          tunnel: w701 -> [w1240]
          tunnel: w700 -> [w1239]
          tunnel: w699 -> [w1238]
          tunnel: w698 -> [w1237]
          tunnel: w697 -> [w1236]
          tunnel: w696 -> [w1235]
          tunnel: w695 -> [w1253]
          tunnel: [w1252] -> w693
          tunnel: w694 -> [w1251]
          tunnel: w693 -> [w1259]
          tunnel: [w1259] -> w692
          tunnel: w692 -> [w1264]
          frame #0 {
            n450 = local write "电动缸速度(mm/s)"("电动缸快速") -> ()
            n451 = local write "已调试次数"(0.0 ("已调试次数")) -> ()
            n452 = local write "选项卡控件"(T1."轴向力测量" ("选项卡控件")) -> ()
            n453 = local read "电动缸电机"() -> (w816:u32)
          }
          frame #1 {
            n454 = while {
              tunnel: [w819] -> _
              tunnel: [w825] -> w817
              tunnel: w818 -> [w819]
              stop <- w820 stop-if-true
              n455 = local read "齿条左极限"() -> (w823:dbl)
              n456 = Wait (ms)(milliseconds to wait=u32 50 ("毫秒倍数")) -> ()  [unwired: 1 out]
              n457 = local read "循环退出"() -> (w822:bool)
              n458 = call "PCI1240电动缸位置模式 .vi"("Distance"=w823, "AxisHandle IN"=w819) -> ("AbsSuccess"=w821:bool, "AxisHandle OUT"=w825:u32)  [unwired: 8 in]
              n459 = Compound Arithmetic op=OR(w821, w822) -> (w820:bool)
            }
          }
          frame #2 {
            n460 = while {
              tunnel: w826 -> [w835]
              stop <- w828 stop-if-true
              n461 = local read "齿条推拉力(N)"() -> (w832:dbl)
              n462 = Wait (ms)(milliseconds to wait=u32 50 ("毫秒倍数")) -> ()  [unwired: 1 out]
              n463 = call <userlib>:"Acm_AxGetCmdVelocity.vi"("AxisHandle"=w835) -> ("Velocity"=w834:dbl)  [unwired: 1 in, 3 out]
              n464 = local read "循环退出"() -> (w827:bool)
              n465 = Less Or Equal?(x=w832, y=-500.0) -> (x <= y?=w829:bool)
              n466 = Equal To 0?(x=w834) -> (x = 0?=w830:bool)
              n467 = Compound Arithmetic op=OR(w830, w829, w827) -> (w828:bool)
            }
          }
          frame #3 {
            n468 = local read "电动缸慢速"() -> (w836:dbl)
            n469 = local write "电动缸速度(mm/s)"(w836) -> ()
            n470 = Wait (ms)(milliseconds to wait=100 ("毫秒倍数")) -> ()  [unwired: 1 out]
          }
          frame #4 {
            n471 = while {
              tunnel: [w847] -> w840
              tunnel: w839 -> [w846]
              stop <- w841 stop-if-true
              n472 = Wait (ms)(milliseconds to wait=u32 50 ("毫秒倍数")) -> ()  [unwired: 1 out]
              n473 = local read "循环退出"() -> (w843:bool)
              n474 = call "PCI1240电动缸位置模式 .vi"("Distance"=118.0, "AxisHandle IN"=w846) -> ("AbsSuccess"=w842:bool, "AxisHandle OUT"=w847:u32)  [unwired: 8 in]
              n475 = Compound Arithmetic op=OR(w842, w843) -> (w841:bool)
            }
          }
          frame #5 {
            n476 = while {
              tunnel: w848 -> [w857]
              stop <- w850 stop-if-true
              n477 = local read "齿条推拉力(N)"() -> (w854:dbl)
              n478 = Wait (ms)(milliseconds to wait=u32 50 ("毫秒倍数")) -> ()  [unwired: 1 out]
              n479 = call <userlib>:"Acm_AxGetCmdVelocity.vi"("AxisHandle"=w857) -> ("Velocity"=w856:dbl)  [unwired: 1 in, 3 out]
              n480 = local read "循环退出"() -> (w849:bool)
              n481 = Less Or Equal?(x=w854, y=-500.0) -> (x <= y?=w851:bool)
              n482 = Equal To 0?(x=w856) -> (x = 0?=w852:bool)
              n483 = Compound Arithmetic op=OR(w852, w851, w849) -> (w850:bool)
            }
          }
          frame #6 {
            n484 = while {
              tunnel: w858 -> [w863]
              stop <- w859 stop-if-true
              n485 = call "PCI1220U停止.vi"("AxisHandle IN"=w863) -> ("完成"=w860:bool)  [unwired: 9 in, 1 out]
              n486 = local read "循环退出"() -> (w861:bool)
              n487 = Wait (ms)(milliseconds to wait=u32 50 ("毫秒倍数")) -> ()  [unwired: 1 out]
              n488 = Compound Arithmetic op=OR(w860, w861) -> (w859:bool)
            }
          }
          frame #7 {
            n489 = local read "电动缸快速"() -> (w864:dbl)
            n490 = Wait (ms)(milliseconds to wait=u32 100 ("毫秒倍数")) -> ()  [unwired: 1 out]
            n491 = local write "电动缸速度(mm/s)"(w864) -> ()
          }
          frame #8 {
            n492 = while {
              tunnel: w868 -> [w876]
              tunnel: [w874] -> w867
              stop <- w870 stop-if-true
              n493 = local read "齿条右极限"() -> (w873:dbl)
              n494 = Wait (ms)(milliseconds to wait=u32 50 ("毫秒倍数")) -> ()  [unwired: 1 out]
              n495 = local read "循环退出"() -> (w872:bool)
              n496 = call "PCI1240电动缸位置模式 .vi"("Distance"=w873, "AxisHandle IN"=w876) -> ("AbsSuccess"=w871:bool, "AxisHandle OUT"=w874:u32)  [unwired: 8 in]
              n497 = Compound Arithmetic op=OR(w871, w872) -> (w870:bool)
            }
            n498 = local read "转向器中心"() -> (w869:dbl)
          }
          frame #9 {
            w882 = dbl[] []
            n499 = while {
              shift-right: [w906] -> w878
              shift-left: w882 -> [w915]
              shift-right: [w913] -> w879
              shift-left: w882 -> [w914]
              tunnel: w881 -> [w910]
              tunnel: w880 -> [w909]
              shift-right: [w905] -> w877
              shift-left: w882 -> [w907]
              stop <- w899 stop-if-true
              n500 = local read "中间位置间隙"() -> (w896:dbl)
              n501 = local read "基准位移"() -> (w911:dbl)
              n502 = local read "间隙位移(mm)"() -> (w895:dbl)
              n503 = local read "电动缸位置(mm)"() -> (w885:dbl)
              n504 = call <userlib>:"Acm_AxGetCmdVelocity.vi"("AxisHandle"=w910) -> ("Velocity"=w904:dbl)  [unwired: 1 in, 3 out]
              n505 = local read "齿条推拉力(N)"() -> (w902:dbl)
              n506 = Subtract(x=w895, y=w911) -> (x-y=w898:dbl)
              n507 = Less Or Equal?(x=w895, y=0.0) -> (x <= y?=w894:bool)
              n508 = Greater Or Equal?(x=w895, y=4.0) -> (x >= y?=w893:bool)
              n509 = Subtract(x=w898, y=w896) -> (x-y=w897:dbl)
              n510 = Subtract(x=w885, y=w909) -> (x-y=w889:dbl)
              n511 = Negate(x=w897) -> (-x=w883:dbl)
              n512 = Multiply(x=w889, y=1.0) -> (x*y=w887:dbl)
              n513 = Build Array (concatenate) ("创建数组")(w914, w883) -> (w913:dbl[])
              n514 = Build Array (concatenate) ("创建数组")(w915, w887) -> (w906:dbl[])
              n515 = Or(x=w893, y=w894) -> (x .or. y?=w892:bool)
              n516 = Build Array (concatenate) ("创建数组")(w907, w902) -> (w905:dbl[])
              n517 = Greater Or Equal?(x=w902, y=500.0) -> (x >= y?=w900:bool)
              n518 = Equal To 0?(x=w904) -> (x = 0?=w901:bool)
              n519 = local read "循环退出"() -> (w884:bool)
              n520 = property on="间隙位移(mm)" class="DigNum (严格)"("Blinking"=w892) -> ()  [unwired: 2 in, 2 out]
              n521 = Bundle ("捆绑")(w906, w913) -> (w886:cluster{dbl[], dbl[]})  [unwired: 1 in]
              n522 = Compound Arithmetic op=OR(w901, w900, w884) -> (w899:bool)
              n523 = Bundle ("捆绑")(w906, w905) -> (w908:cluster{dbl[], dbl[]})  [unwired: 1 in]
              n524 = Build Array ("创建数组")(w886, w908) -> (w912:cluster{dbl[], dbl[]}[])
              n525 = local write "行程跳动曲线"(w912) -> ()
              n526 = Wait (ms)(milliseconds to wait=u32 50 ("毫秒倍数")) -> ()  [unwired: 1 out]
            }
          }
          frame #10 {
            n527 = local read "电动缸慢速"() -> (w917:dbl)
            n528 = local write "电动缸速度(mm/s)"(w917) -> ()
          }
          frame #11 {
            n529 = while {
              tunnel: w923 -> [w932]
              tunnel: [w931] -> w922
              stop <- w927 stop-if-true
              n530 = Wait Until Next ms Multiple(millisecond multiple=u32 50 ("毫秒倍数")) -> ()  [unwired: 1 out]
              n531 = local read "循环退出"() -> (w929:bool)
              n532 = call "PCI1240电动缸位置模式 .vi"("Distance"=-50.0, "AxisHandle IN"=w932) -> ("AbsSuccess"=w928:bool, "AxisHandle OUT"=w931:u32)  [unwired: 8 in]
              n533 = Compound Arithmetic op=OR(w928, w929) -> (w927:bool)
            }
          }
          frame #12 {
            n534 = local read "转向器中心"() -> (w935:dbl)
            n535 = while {
              shift-right: [w965] -> w940
              shift-left: w937 -> [w974]
              shift-right: [w972] -> w941
              shift-left: w938 -> [w973]
              tunnel: w934 -> [w969]
              tunnel: w935 -> [w968]
              shift-right: [w964] -> w939
              shift-left: w936 -> [w966]
              stop <- w958 stop-if-true
              n536 = local read "中间位置间隙"() -> (w955:dbl)
              n537 = local read "基准位移"() -> (w970:dbl)
              n538 = local read "间隙位移(mm)"() -> (w954:dbl)
              n539 = call <userlib>:"Acm_AxGetCmdVelocity.vi"("AxisHandle"=w969) -> ("Velocity"=w963:dbl)  [unwired: 1 in, 3 out]
              n540 = local read "电动缸位置(mm)"() -> (w944:dbl)
              n541 = Wait (ms)(milliseconds to wait=u32 50 ("毫秒倍数")) -> ()  [unwired: 1 out]
              n542 = local read "齿条推拉力(N)"() -> (w961:dbl)
              n543 = Subtract(x=w954, y=w970) -> (x-y=w957:dbl)
              n544 = Less Or Equal?(x=w954, y=0.0) -> (x <= y?=w953:bool)
              n545 = Greater Or Equal?(x=w954, y=4.0) -> (x >= y?=w952:bool)
              n546 = Subtract(x=w957, y=w955) -> (x-y=w956:dbl)
              n547 = Subtract(x=w944, y=w968) -> (x-y=w948:dbl)
              n548 = Negate(x=w956) -> (-x=w942:dbl)
              n549 = Multiply(x=w948, y=1.0) -> (x*y=w946:dbl)
              n550 = Build Array (concatenate) ("创建数组")(w973, w942) -> (w972:dbl[])
              n551 = Build Array (concatenate) ("创建数组")(w974, w946) -> (w965:dbl[])
              n552 = Build Array (concatenate) ("创建数组")(w966, w961) -> (w964:dbl[])
              n553 = Greater Or Equal?(x=w961, y=500.0) -> (x >= y?=w959:bool)
              n554 = local read "循环退出"() -> (w943:bool)
              n555 = Or(x=w952, y=w953) -> (x .or. y?=w951:bool)
              n556 = Equal To 0?(x=w963) -> (x = 0?=w960:bool)
              n557 = property on="间隙位移(mm)" class="DigNum (严格)"("Blinking"=w951) -> ()  [unwired: 2 in, 2 out]
              n558 = Bundle ("捆绑")(w965, w972) -> (w945:cluster{dbl[], dbl[]})  [unwired: 1 in]
              n559 = Compound Arithmetic op=OR(w960, w959, w943) -> (w958:bool)
              n560 = Bundle ("捆绑")(w965, w964) -> (w967:cluster{dbl[], dbl[]})  [unwired: 1 in]
              n561 = Build Array ("创建数组")(w945, w967) -> (w971:cluster{dbl[], dbl[]}[])
              n562 = local write "行程跳动曲线"(w971) -> ()
            }
          }
          frame #13 {
            n563 = call "间隙计算.vi"("扭矩数组"=w995) -> ("峰值间隙1"=w987:dbl, "峰值间隙2"=w986:dbl)  [unwired: 6 in, 3 out]
            n564 = call "功能计算_何 截取位移左.vi"("位移数组"=w979, "拉压力数组"=w993, "半行程"="半行程", "截取百分比"="截取百分比") -> ("峰值扭矩"=w992:dbl, "平均扭矩"=w991:dbl, "扭差"=w990:dbl)  [unwired: 12 in, 1 out]
            "左最大轴向力(N)" <- w992
            "左轴向力波动(N)" <- w990
            "左平均轴向力(N)" <- w991
            n565 = while {
              tunnel: w994 -> [w1001]
              tunnel: [w1000] -> w977
              stop <- w996 stop-if-true
              n566 = local read "循环退出"() -> (w998:bool)
              n567 = call "PCI1220U停止.vi"("AxisHandle IN"=w1001) -> ("完成"=w997:bool, "AxisHandle OUT"=w1000:u32)  [unwired: 9 in]
              n568 = Wait (ms)(milliseconds to wait=u32 50 ("毫秒倍数")) -> ()  [unwired: 1 out]
              n569 = Compound Arithmetic op=OR(w997, w998) -> (w996:bool)
            }
            n570 = Array Size(array=w979) -> (size(s)=→"左轴向力数组大小":i32)
            n571 = local read "全行程180°外间隙标准(mm)"() -> (w984:dbl)
            n572 = local read "全行程180°内间隙标准(mm)"() -> (w985:dbl)
            n573 = local write "左180°内全行程间隙"(w987) -> ()
            n574 = local write "左180°外全行程间隙"(w986) -> ()
            n575 = local read "电动缸快速"() -> (w976:dbl)
            n576 = Less?(x=w986, y=w984) -> (x < y?=w988:bool)
            n577 = Less?(x=w987, y=w985) -> (x < y?=w989:bool)
            n578 = Not(x=w988) -> (.not. x?=w982:bool)
            n579 = local write "电动缸速度(mm/s)"(w976) -> ()
            n580 = Not(x=w989) -> (.not. x?=w983:bool)
            n581 = property on="左180°外全行程间隙" class="DigNum (严格)"("Blinking"=w982) -> ()  [unwired: 2 in, 2 out]
            n582 = property on="左180°内全行程间隙" class="DigNum (严格)"("Blinking"=w983) -> ()  [unwired: 2 in, 2 out]
          }
          frame #14 {
            n583 = local read "最大轴向力标准(N)"() -> (w1010:dbl)
            n584 = while {
              tunnel: w1016 -> [w1024]
              stop <- w1019 stop-if-true
              n585 = local read "齿条左极限"() -> (w1022:dbl)
              n586 = Wait Until Next ms Multiple(millisecond multiple=u32 50 ("毫秒倍数")) -> ()  [unwired: 1 out]
              n587 = local read "循环退出"() -> (w1021:bool)
              n588 = call "PCI1240电动缸位置模式 .vi"("Distance"=w1022, "AxisHandle IN"=w1024) -> ("AbsSuccess"=w1020:bool)  [unwired: 8 in, 1 out]
              n589 = Compound Arithmetic op=OR(w1020, w1021) -> (w1019:bool)
            }
            n590 = local read "轴向力标准(N)"() -> (w1009:dbl)
            n591 = local read "平均轴向力MAX(N)"() -> (w1008:dbl)
            n592 = local read "力波动标准(N)"() -> (w1007:dbl)
            n593 = call "判断.vi"("y 3"=w1007, "y2-2"=w1008, "y2-1"=w1009, "y"=w1010, "x 3"=w1013, "x 2"=w1014, "x"=w1012) -> ("非x? 3"=w1005:bool, "非x? 2"=w1011:bool, "非x?"=w1006:bool)  [unwired: 2 in]
            n594 = property on="左最大轴向力(N)" class="DigNum (严格)"("Blinking"=w1006) -> ()  [unwired: 2 in, 2 out]
            n595 = property on="左轴向力波动(N)" class="DigNum (严格)"("Blinking"=w1005) -> ()  [unwired: 2 in, 2 out]
            n596 = property on="左平均轴向力(N)" class="DigNum (严格)"("Blinking"=w1011) -> ()  [unwired: 2 in, 2 out]
            n597 = local read "转向器中心"() -> (w1002:dbl)
          }
          frame #15 {
            n598 = while {
              shift-right: [w1043] -> w1030
              shift-left: w1033 -> [w1071]
              shift-right: [w1069] -> w1031
              shift-left: w1034 -> [w1070]
              tunnel: w1025 -> [w1066]
              tunnel: w1029 -> [w1065]
              shift-right: [w1062] -> w1028
              shift-left: w1032 -> [w1063]
              stop <- w1057 stop-if-true
              n599 = local read "电动缸位置(mm)"() -> (w1039:dbl)
              n600 = local read "间隙位移(mm)"() -> (w1049:dbl)
              n601 = call <userlib>:"Acm_AxGetCmdVelocity.vi"("AxisHandle"=w1066) -> ("Velocity"=w1055:dbl)  [unwired: 1 in, 3 out]
              n602 = local read "基准位移"() -> (w1067:dbl)
              n603 = Wait (ms)(milliseconds to wait=u32 50 ("毫秒倍数")) -> ()  [unwired: 1 out]
              n604 = local read "中间位置间隙"() -> (w1054:dbl)
              n605 = local read "齿条推拉力(N)"() -> (w1061:dbl)
              n606 = Subtract(x=w1049, y=w1067) -> (x-y=w1068:dbl)
              n607 = local read "循环退出"() -> (w1038:bool)
              n608 = Subtract(x=w1039, y=2.7) -> (x-y=w1040:dbl)
              n609 = Subtract(x=w1040, y=w1065) -> (x-y=w1047:dbl)
              n610 = Subtract(x=w1068, y=w1054) -> (x-y=w1056:dbl)
              n611 = Negate(x=w1056) -> (-x=w1037:dbl)
              n612 = Less Or Equal?(x=w1061, y=-500.0) -> (x <= y?=w1058:bool)
              n613 = Equal To 0?(x=w1055) -> (x = 0?=w1059:bool)
              n614 = Multiply(x=w1047, y=1.0) -> (x*y=w1045:dbl)
              n615 = Build Array (concatenate) ("创建数组")(w1071, w1045) -> (w1043:dbl[])
              n616 = Build Array (concatenate) ("创建数组")(w1063, w1061) -> (w1062:dbl[])
              n617 = Build Array (concatenate) ("创建数组")(w1070, w1037) -> (w1069:dbl[])
              n618 = Compound Arithmetic op=OR(w1059, w1058, w1038) -> (w1057:bool)
              n619 = Bundle ("捆绑")(w1043, w1069) -> (w1044:cluster{dbl[], dbl[]})  [unwired: 1 in]
              n620 = Bundle ("捆绑")(w1043, w1062) -> (w1064:cluster{dbl[], dbl[]})  [unwired: 1 in]
              n621 = Build Array ("创建数组")(w1044, w1064) -> (w1042:cluster{dbl[], dbl[]}[])
              n622 = Less Or Equal?(x=w1049, y=0.0) -> (x <= y?=w1053:bool)
              n623 = Greater Or Equal?(x=w1049, y=4.0) -> (x >= y?=w1052:bool)
              n624 = Or(x=w1052, y=w1053) -> (x .or. y?=w1048:bool)
              n625 = local write "行程跳动曲线"(w1042) -> ()
              n626 = property on="间隙位移(mm)" class="DigNum (严格)"("Blinking"=w1048) -> ()  [unwired: 2 in, 2 out]
            }
          }
          frame #16 {
            n627 = local read "电动缸慢速"() -> (w1073:dbl)
            n628 = local write "电动缸速度(mm/s)"(w1073) -> ()
          }
          frame #17 {
            n629 = while {
              tunnel: w1082 -> [w1096]
              stop <- w1091 stop-if-true
              n630 = Wait Until Next ms Multiple(millisecond multiple=u32 50 ("毫秒倍数")) -> ()  [unwired: 1 out]
              n631 = call "PCI1240电动缸位置模式 .vi"("Distance"=130.0, "AxisHandle IN"=w1096) -> ("AbsSuccess"=w1092:bool)  [unwired: 8 in, 1 out]
              n632 = local read "循环退出"() -> (w1093:bool)
              n633 = Compound Arithmetic op=OR(w1092, w1093) -> (w1091:bool)
            }
            n634 = local read "转向器中心"() -> (w1083:dbl)
          }
          frame #18 {
            n635 = while {
              shift-right: [w1115] -> w1107
              shift-left: w1102 -> [w1143]
              shift-right: [w1141] -> w1108
              shift-left: w1103 -> [w1142]
              tunnel: w1097 -> [w1138]
              tunnel: w1101 -> [w1137]
              shift-right: [w1134] -> w1106
              shift-left: w1100 -> [w1135]
              stop <- w1129 stop-if-true
              n636 = local read "电动缸位置(mm)"() -> (w1111:dbl)
              n637 = local read "间隙位移(mm)"() -> (w1121:dbl)
              n638 = call <userlib>:"Acm_AxGetCmdVelocity.vi"("AxisHandle"=w1138) -> ("Velocity"=w1127:dbl)  [unwired: 1 in, 3 out]
              n639 = local read "基准位移"() -> (w1139:dbl)
              n640 = Wait (ms)(milliseconds to wait=u32 50 ("毫秒倍数")) -> ()  [unwired: 1 out]
              n641 = local read "中间位置间隙"() -> (w1126:dbl)
              n642 = local read "齿条推拉力(N)"() -> (w1133:dbl)
              n643 = local read "循环退出"() -> (w1110:bool)
              n644 = Subtract(x=w1121, y=w1139) -> (x-y=w1140:dbl)
              n645 = Subtract(x=w1111, y=2.7) -> (x-y=w1112:dbl)
              n646 = Subtract(x=w1112, y=w1137) -> (x-y=w1119:dbl)
              n647 = Subtract(x=w1140, y=w1126) -> (x-y=w1128:dbl)
              n648 = Negate(x=w1128) -> (-x=w1109:dbl)
              n649 = Multiply(x=w1119, y=1.0) -> (x*y=w1117:dbl)
              n650 = Less Or Equal?(x=w1133, y=-500.0) -> (x <= y?=w1130:bool)
              n651 = Build Array (concatenate) ("创建数组")(w1143, w1117) -> (w1115:dbl[])
              n652 = Build Array (concatenate) ("创建数组")(w1135, w1133) -> (w1134:dbl[])
              n653 = Equal To 0?(x=w1127) -> (x = 0?=w1131:bool)
              n654 = Build Array (concatenate) ("创建数组")(w1142, w1109) -> (w1141:dbl[])
              n655 = Bundle ("捆绑")(w1115, w1134) -> (w1136:cluster{dbl[], dbl[]})  [unwired: 1 in]
              n656 = Compound Arithmetic op=OR(w1131, w1130, w1110) -> (w1129:bool)
              n657 = Bundle ("捆绑")(w1115, w1141) -> (w1116:cluster{dbl[], dbl[]})  [unwired: 1 in]
              n658 = Build Array ("创建数组")(w1116, w1136) -> (w1114:cluster{dbl[], dbl[]}[])
              n659 = Less Or Equal?(x=w1121, y=0.0) -> (x <= y?=w1125:bool)
              n660 = Greater Or Equal?(x=w1121, y=4.0) -> (x >= y?=w1124:bool)
              n661 = Or(x=w1124, y=w1125) -> (x .or. y?=w1120:bool)
              n662 = local write "行程跳动曲线"(w1114) -> ()
              n663 = property on="间隙位移(mm)" class="DigNum (严格)"("Blinking"=w1120) -> ()  [unwired: 2 in, 2 out]
            }
          }
          frame #19 {
            n664 = while {
              tunnel: w1145 -> [w1163]
              tunnel: [w1162] -> _
              stop <- w1158 stop-if-true
              n665 = call "PCI1220U停止.vi"("AxisHandle IN"=w1163) -> ("完成"=w1159:bool, "AxisHandle OUT"=w1162:u32)  [unwired: 9 in]
              n666 = Wait (ms)(milliseconds to wait=u32 50 ("毫秒倍数")) -> ()  [unwired: 1 out]
              n667 = local read "循环退出"() -> (w1160:bool)
              n668 = Compound Arithmetic op=OR(w1159, w1160) -> (w1158:bool)
            }
            n669 = Array Max & Min(array=w1151) -> (max value=w1155:dbl, min value=w1154:dbl)  [unwired: 2 out]
            n670 = local read "左轴向力数组大小"() -> (w1146:i32)
            n671 = Absolute Value(x=w1155) -> (abs(x)=w1153:dbl)
            n672 = Absolute Value(x=w1154) -> (abs(x)=w1152:dbl)
            n673 = local write "右全行程间隙"(w1152) -> ()
            n674 = local write "左全行程间隙"(w1153) -> ()
          }
          frame #20 {
            (unwired) 46.996 ("y")
            n675 = local read "半行程"() -> (w1169:dbl)
            n676 = local read "全行程180°外间隙标准(mm)"() -> (w1204:dbl)
            n677 = Split 1D Array(array=w1166, index=w1164) -> (second subarray=w1167:dbl[])  [unwired: 1 out]
            n678 = local read "截取百分比"() -> (w1168:dbl)
            n679 = local read "全行程180°外间隙标准(mm)"() -> (w1186:dbl)
            n680 = Split 1D Array(array=w1208, index=w1164) -> (second subarray=w1170:dbl[])  [unwired: 1 out]
            n681 = local read "全行程180°内间隙标准(mm)"() -> (w1187:dbl)
            n682 = Array Max & Min(array=w1166) -> (max value=w1200:dbl, min value=w1199:dbl)  [unwired: 2 out]
            n683 = local read "总行程标准(mm)"() -> (w1181:dbl)
            n684 = call "功能计算_何 截取位移右.vi"("位移数组"=w1167, "拉压力数组"=w1170, "半行程"=w1169, "截取百分比"=w1168) -> ("峰值扭矩"=w1197:dbl, "平均扭矩"=w1207:dbl, "扭差"=w1196:dbl)  [unwired: 12 in, 1 out]
            n685 = Split 1D Array(array=w1189, index=w1164) -> (second subarray=w1188:dbl[])  [unwired: 1 out]
            n686 = Subtract(x=w1200, y=w1199) -> (x-y=w1191:dbl)
            n687 = Subtract(x=w1191, y="机械间隙值") -> (x-y=w1173:dbl)
            n688 = local write "总行程(mm)"(w1173) -> ()
            n689 = local write "右最大轴向力(N)"(w1197) -> ()
            n690 = Greater?(x=w1206, y=w1204) -> (0:w1193:bool)
            n691 = call "间隙计算.vi"("扭矩数组"=w1188) -> ("峰值间隙1"=w1203:dbl, "峰值间隙2"=w1202:dbl)  [unwired: 6 in, 3 out]
            n692 = Greater?(x=w1205, y=w1204) -> (0:w1192:bool)
            n693 = local write "右轴向力波动(N)"(w1196) -> ()
            n694 = local write "右平均轴向力(N)"(w1207) -> ()
            n695 = local read "总行程最大值"() -> (w1182:dbl)
            n696 = In Range and Coerce "判定范围并强制转换"(upper limit=w1182, x=w1173, lower limit=w1181) -> (In Range?=w1179:bool)  [unwired: 1 out]
            n697 = Less?(x=w1202, y=w1186) -> (x < y?=w1180:bool)
            n698 = Less?(x=w1203, y=w1187) -> (x < y?=w1201:bool)
            n699 = local write "右180°外全行程间隙"(w1202) -> ()
            n700 = local read "总圈数最大值"() -> (w1183:dbl)
            n701 = local write "右180°内全行程间隙"(w1203) -> ()
            n702 = property on="左全行程间隙" class="DigNum (严格)"("Blinking"=w1193) -> ()  [unwired: 2 in, 2 out]
            n703 = property on="右全行程间隙" class="DigNum (严格)"("Blinking"=w1192) -> ()  [unwired: 2 in, 2 out]
            n704 = Divide(x=w1173, y="齿条传动比") -> (x/y=w1185:dbl)
            n705 = Not(x=w1201) -> (.not. x?=w1175:bool)
            n706 = Not(x=w1180) -> (.not. x?=w1174:bool)
            n707 = property on="右180°外全行程间隙" class="DigNum (严格)"("Blinking"=w1174) -> ()  [unwired: 2 in, 2 out]
            n708 = local read "总圈数标准"() -> (w1184:dbl)
            n709 = In Range and Coerce(upper limit=w1183, x=w1185, lower limit=w1184) -> (In Range?=w1178:bool)  [unwired: 1 out]
            n710 = Not(x=w1179) -> (.not. x?=w1177:bool)
            n711 = local read "最大轴向力标准(N)"() -> (w1165:dbl)
            n712 = local write "总圈数"(w1185) -> ()
            n713 = Not(x=w1178) -> (.not. x?=w1176:bool)
            n714 = property on="总行程(mm)" class="DigNum (严格)"("Blinking"=w1177) -> ()  [unwired: 2 in, 2 out]
            n715 = property on="右180°内全行程间隙" class="DigNum (严格)"("Blinking"=w1175) -> ()  [unwired: 2 in, 2 out]
            n716 = property on="总圈数" class="DigNum (严格)"("Blinking"=w1176) -> ()  [unwired: 2 in, 2 out]
            "轴向力X" <- w1166
            "轴向力Y" <- w1208
          }
          frame #21 {
            n717 = local read "电动缸快速"() -> (w1210:dbl)
            n718 = local read "转向器中心"() -> (w1230:dbl)
            n719 = local read "平均轴向力MAX(N)"() -> (w1224:dbl)
            n720 = local read "轴向力标准(N)"() -> (w1225:dbl)
            n721 = local read "力波动标准(N)"() -> (w1223:dbl)
            n722 = call "判断.vi"("y 3"=w1223, "y2-2"=w1224, "y2-1"=w1225, "y"=w1211, "x 3"=w1226, "x 2"=w1233, "x"=w1229) -> ("非x? 3"=w1227:bool, "非x? 2"=w1228:bool, "非x?"=w1218:bool)  [unwired: 2 in]
            n723 = local write "电动缸速度(mm/s)"(w1210) -> ()
            n724 = property on="右最大轴向力(N)" class="DigNum (严格)"("Blinking"=w1218) -> ()  [unwired: 2 in, 2 out]
            n725 = property on="右平均轴向力(N)" class="DigNum (严格)"("Blinking"=w1228) -> ()  [unwired: 2 in, 2 out]
            n726 = Add(x=w1230, y=0.0) -> (x+y=w1231:dbl)
          }
          frame #22 {
            n727 = Compound Arithmetic op=OR(w1240, w1247, w1246, w1245, w1238, w1237, w1241, w1244, w1243, w1239, w1236, w1235) -> (w1242:bool)
            n728 = property on="右轴向力波动(N)" class="DigNum (严格)"("Blinking"=w1241) -> ()  [unwired: 2 in, 2 out]
            n729 = Not(x=w1242) -> (.not. x?=w1248:bool)
            n730 = local write "全行程间隙及轴向力合格"(w1248) -> ()
          }
          frame #23 {
            n731 = while {
              tunnel: w1253 -> [w1257]
              tunnel: [w1255] -> w1252
              tunnel: w1251 -> [w1254]
              stop <- w1256 stop-if-true
              n732 = call "PCI1240电动缸位置模式 .vi"("Distance"=w1254, "AxisHandle IN"=w1257) -> ("AbsSuccess"=w1256:bool, "AxisHandle OUT"=w1255:u32)  [unwired: 8 in]
              n733 = Wait (ms)(milliseconds to wait=u32 50 ("毫秒倍数")) -> ()  [unwired: 1 out]
            }
          }
          frame #24 {
            n734 = while {
              tunnel: w1259 -> [w1263]
              stop <- w1261 stop-if-true
              n735 = call <userlib>:"Acm_AxGetCmdVelocity.vi"("AxisHandle"=w1263) -> ("Velocity"=w1262:dbl)  [unwired: 1 in, 3 out]
              n736 = Wait Until Next ms Multiple(millisecond multiple=u32 50 ("毫秒倍数")) -> ()  [unwired: 1 out]
              n737 = Equal To 0?(x=w1262) -> (x = 0?=w1261:bool)
            }
          }
          frame #25 {
            n738 = call "PCI1220U停止.vi"("AxisHandle IN"=w1264) -> ()  [unwired: 9 in, 2 out]
          }
          frame #26 {
            n739 = local read "轴向力已做次数"() -> (w1267:dbl)
            n740 = Add(x=w1267, y=1.0) -> (x+y=w1265:dbl)
            n741 = local write "轴向力已做次数"(w1265) -> ()
          }
          frame #27 {
            n742 = local read "全行程间隙及轴向力合格"() -> (w1268:bool)
            n743 = case shown="假" w1268 {
              frame False {
                n744 = Less?(x="轴向力已做次数", y="设定轴向力调整次数") -> (x < y?=w1270:bool)
                n745 = case shown="真" w1270 {
                  frame False {
                    n746 = local write "工步号"(u32 45 ("工步号")) -> ()
                  }
                  frame True {
                    n747 = local write "工步号"(u32 30 ("工步号")) -> ()
                  }
                }
              }
              frame True {
                n748 = local write "工步号"(u32 45 ("工步号")) -> ()
              }
            }
          }
        }
      }
      frame 45 {
        # "测头退回"
        n749 = flat-sequence {
          tunnel: [w1278] -> w1275
          tunnel: w1275 -> [w1285]
          frame #0 {
            n750 = local write "测头机构轴速度(mm/s)"(30.0 ("测头机构轴速度(mm/s)")) -> ()
          }
          frame #1 {
            n751 = local read "测头机构轴后退位"() -> (w1277:dbl)
            n752 = local read "测头机构电机"() -> (w1279:u32)
            n753 = while {
              tunnel: w1279 -> [w1283]
              tunnel: w1277 -> [w1282]
              tunnel: [w1281] -> w1278
              stop <- w1284 stop-if-true
              n754 = Wait Until Next ms Multiple(millisecond multiple=u32 50 ("毫秒倍数")) -> ()  [unwired: 1 out]
              n755 = call "PCI1220U进给轴位置模式.vi"("Distance"=w1282, "AxisHandle IN"=w1283) -> ("AbsSuccess"=w1284:bool, "AxisHandle OUT"=w1281:u32)  [unwired: 8 in]
            }
          }
          frame #2 {
            n756 = while {
              tunnel: w1285 -> [w1289]
              stop <- w1287 stop-if-true
              n757 = call <userlib>:"Acm_AxGetCmdVelocity.vi"("AxisHandle"=w1289) -> ("Velocity"=w1288:dbl)  [unwired: 1 in, 3 out]
              n758 = Wait Until Next ms Multiple(millisecond multiple=u32 50 ("毫秒倍数")) -> ()  [unwired: 1 out]
              n759 = Equal To 0?(x=w1288) -> (x = 0?=w1287:bool)
            }
          }
          frame #3 {
            n760 = while {
              stop <- w1290 stop-if-true
              n761 = local read "测头机构轴位置(mm)"() -> (w1292:dbl)
              n762 = Wait Until Next ms Multiple(millisecond multiple=u32 50 ("毫秒倍数")) -> ()  [unwired: 1 out]
              n763 = Less Or Equal?(x=w1292, y=35.0) -> (x <= y?=w1290:bool)
            }
          }
          frame #4 {
            n764 = local write "测头气缸左移"(TRUE ("测头气缸左移")) -> ()
            n765 = local write "测头气缸右移"(FALSE ("测头气缸右移")) -> ()
          }
          frame #5 {
            n766 = Wait Until Next ms Multiple(millisecond multiple=u32 500 ("毫秒倍数")) -> ()  [unwired: 1 out]
          }
          frame #6 {
            n767 = local write "工步号"(u32 50 ("工步号")) -> ()
          }
        }
      }
      frame 50 {
        n768 = flat-sequence {
          tunnel: [w1319] -> w1308
          tunnel: w1308 -> [w1326]
          tunnel: [w1325] -> w1306
          tunnel: w1306 -> [w1337]
          tunnel: [w1344] -> w1300
          tunnel: [w1348] -> w1301
          tunnel: w1300 -> [w1348]
          tunnel: [w1351] -> w1303
          tunnel: w1301 -> [w1350]
          tunnel: w1303 -> [w1358]
          tunnel: [w1357] -> w1302
          tunnel: w1302 -> [w1360]
          tunnel: [w1359] -> w1298
          tunnel: [w1365] -> w1299
          tunnel: w1298 -> [w1365]
          tunnel: [w1368] -> w1307
          tunnel: w1299 -> [w1367]
          tunnel: w1307 -> [w1374]
          tunnel: [w1375] -> w1305
          tunnel: w1305 -> [w1384]
          tunnel: [w1383] -> w1304
          tunnel: w1304 -> [w1394]
          frame #0 {
            n769 = local write "旋转伺服速度(°/s)"(15.0 ("调整螺塞轴速度(°/s)")) -> ()
            n770 = local write "测头机构轴速度(mm/s)"(15.0 ("调整机构轴速度(mm/s)")) -> ()
            n771 = local write "电动缸速度(mm/s)"(15.0 ("电动缸速度(mm/s)")) -> ()
            n772 = local write "夹头松开"(TRUE ("夹头松开")) -> ()
            n773 = local write "夹头夹紧"(FALSE ("夹头夹紧")) -> ()
          }
          frame #1 {
            n774 = while {
              stop <- w1314 stop-if-true
              n775 = local read "夹头夹紧位"() -> (w1317:bool)
              n776 = local read "夹头松开"() -> (w1315:bool)
              n777 = Wait Until Next ms Multiple(millisecond multiple=u32 50 ("毫秒倍数")) -> ()  [unwired: 1 out]
              n778 = Not(x=w1317) -> (.not. x?=w1316:bool)
              n779 = And(x=w1316, y=w1315) -> (x .and. y?=w1314:bool)
            }
          }
          frame #2 {
            n780 = while {
              tunnel: [w1322] -> w1319
              stop <- w1321 stop-if-true
              n781 = local read "电动缸电机"() -> (w1323:u32)
              n782 = Wait Until Next ms Multiple(millisecond multiple=u32 50 ("毫秒倍数")) -> ()  [unwired: 1 out]
              n783 = local read "齿条右极限"() -> (w1320:dbl)
              n784 = call "PCI1240电动缸位置模式 .vi"("Distance"=w1320, "AxisHandle IN"=w1323) -> ("AbsSuccess"=w1321:bool, "AxisHandle OUT"=w1322:u32)  [unwired: 8 in]
            }
          }
          frame #3 {
            n785 = while {
              tunnel: w1326 -> [w1335]
              tunnel: [w1327] -> w1325
              stop <- w1328 stop-if-true
              n786 = local read "齿条推拉力(N)"() -> (w1333:dbl)
              n787 = Wait Until Next ms Multiple(millisecond multiple=u32 50 ("毫秒倍数")) -> ()  [unwired: 1 out]
              n788 = call <userlib>:"Acm_AxGetCmdVelocity.vi"("AxisHandle"=w1335) -> ("Velocity"=w1336:dbl, "AxisHandle"=w1327:u32)  [unwired: 1 in, 2 out]
              n789 = Equal To 0?(x=w1336) -> (x = 0?=w1330:bool)
              n790 = Absolute Value(x=w1333) -> (abs(x)=w1332:dbl)
              n791 = Greater Or Equal?(x=w1332, y=1000.0) -> (x >= y?=w1329:bool)
              n792 = Or(x=w1330, y=w1329) -> (x .or. y?=w1328:bool)
            }
          }
          frame #4 {
            n793 = while {
              tunnel: w1337 -> [w1341]
              tunnel: [w1340] -> _
              stop <- w1339 stop-if-true
              n794 = call "PCI1220U停止.vi"("AxisHandle IN"=w1341) -> ("完成"=w1339:bool, "AxisHandle OUT"=w1340:u32)  [unwired: 9 in]
              n795 = Wait (ms)(milliseconds to wait=u32 50 ("毫秒倍数")) -> ()  [unwired: 1 out]
            }
          }
          frame #5 {
            n796 = local write "旋转齿条轴使能"(TRUE ("旋转齿条轴使能")) -> ()
          }
          frame #6 {
            n797 = Wait Until Next ms Multiple(millisecond multiple=u32 500 ("毫秒倍数")) -> ()  [unwired: 1 out]
          }
          frame #7 {
            n798 = local read "旋转齿条电机"() -> (w1345:u32)
            n799 = call <userlib>:"Acm_AxHome.vi"("DirMode"=u32 0, "HomeMode"=u32 11, "AxisHandle"=w1345) -> ("AxisHandle"=w1344:u32)  [unwired: 1 in, 2 out]
          }
          frame #8 {
            n800 = Wait Until Next ms Multiple(millisecond multiple=u32 100 ("毫秒倍数")) -> ()  [unwired: 1 out]
          }
          frame #9 {
            n801 = while {
              tunnel: w1350 -> [w1354]
              tunnel: [w1353] -> w1351
              stop <- w1352 stop-if-true
              n802 = call <userlib>:"Acm_AxGetCmdVelocity.vi"("AxisHandle"=w1354) -> ("Velocity"=w1356:dbl, "AxisHandle"=w1353:u32)  [unwired: 1 in, 2 out]
              n803 = Equal To 0?(x=w1356) -> (x = 0?=w1352:bool)
              n804 = Wait Until Next ms Multiple(millisecond multiple=u32 50 ("毫秒倍数")) -> ()  [unwired: 1 out]
            }
          }
          frame #10 {
            n805 = call "PCI1220U角度置零.vi"("AxisHandle IN"=w1358) -> ("AxisHandle OUT"=w1357:u32)  [unwired: 10 in]
          }
          frame #11 {
            n806 = while {
              tunnel: [w1361] -> w1359
              tunnel: w1360 -> [w1361]
              stop <- w1364 stop-if-true
              n807 = Wait Until Next ms Multiple(millisecond multiple=u32 50 ("毫秒倍数")) -> ()  [unwired: 1 out]
              n808 = call "PCI1220U扭矩轴位置模式.vi"("Distance"=15.0, "AxisHandle IN"=w1361) -> ("AbsSuccess"=w1364:bool)  [unwired: 8 in, 1 out]
            }
          }
          frame #12 {
            n809 = Wait Until Next ms Multiple(millisecond multiple=u32 100 ("毫秒倍数")) -> ()  [unwired: 1 out]
          }
          frame #13 {
            n810 = while {
              tunnel: w1367 -> [w1371]
              tunnel: [w1370] -> w1368
              stop <- w1369 stop-if-true
              n811 = call <userlib>:"Acm_AxGetCmdVelocity.vi"("AxisHandle"=w1371) -> ("Velocity"=w1373:dbl, "AxisHandle"=w1370:u32)  [unwired: 1 in, 2 out]
              n812 = Equal To 0?(x=w1373) -> (x = 0?=w1369:bool)
              n813 = Wait Until Next ms Multiple(millisecond multiple=u32 50 ("毫秒倍数")) -> ()  [unwired: 1 out]
            }
          }
          frame #14 {
            n814 = call "PCI1220U角度置零.vi"("AxisHandle IN"=w1374) -> ()  [unwired: 10 in, 1 out]
          }
          frame #15 {
            n815 = while {
              tunnel: [w1380] -> w1375
              stop <- w1379 stop-if-true
              n816 = local read "电动缸电机"() -> (w1381:u32)
              n817 = Wait Until Next ms Multiple(millisecond multiple=u32 50 ("毫秒倍数")) -> ()  [unwired: 1 out]
              n818 = local read "齿条右极限"() -> (w1378:dbl)
              n819 = Add(x=w1378, y=-10.0) -> (x+y=w1376:dbl)
              n820 = call "PCI1240电动缸位置模式 .vi"("Distance"=w1376, "AxisHandle IN"=w1381) -> ("AbsSuccess"=w1379:bool, "AxisHandle OUT"=w1380:u32)  [unwired: 8 in]
            }
          }
          frame #16 {
            n821 = while {
              tunnel: w1384 -> [w1392]
              tunnel: [w1390] -> w1383
              stop <- w1385 stop-if-true
              n822 = local read "齿条推拉力(N)"() -> (w1389:dbl)
              n823 = Wait Until Next ms Multiple(millisecond multiple=u32 50 ("毫秒倍数")) -> ()  [unwired: 1 out]
              n824 = call <userlib>:"Acm_AxGetCmdVelocity.vi"("AxisHandle"=w1392) -> ("Velocity"=w1393:dbl, "AxisHandle"=w1390:u32)  [unwired: 1 in, 2 out]
              n825 = Equal To 0?(x=w1393) -> (x = 0?=w1386:bool)
              n826 = Greater Or Equal?(x=w1389, y=300.0) -> (x >= y?=w1387:bool)
              n827 = Or(x=w1386, y=w1387) -> (x .or. y?=w1385:bool)
            }
          }
          frame #17 {
            n828 = while {
              tunnel: w1394 -> [w1398]
              tunnel: [w1397] -> _
              stop <- w1396 stop-if-true
              n829 = call "PCI1220U停止.vi"("AxisHandle IN"=w1398) -> ("完成"=w1396:bool, "AxisHandle OUT"=w1397:u32)  [unwired: 9 in]
              n830 = Wait (ms)(milliseconds to wait=u32 50 ("毫秒倍数")) -> ()  [unwired: 1 out]
            }
          }
          frame #18 {
            n831 = local write "工步号"(u32 100 ("工步号")) -> ()
          }
        }
      }
      frame 100 {
        n832 = flat-sequence {
          tunnel: [w1433] -> w1423
          tunnel: [w1431] -> w1422
          tunnel: [w1425] -> w1409
          tunnel: [w1424] -> w1407
          tunnel: w1423 -> [w1440]
          tunnel: w1422 -> [w1437]
          tunnel: ["F:\\报表存储\\" ("字符串")] -> w1421
          tunnel: [w1440] -> w1410
          tunnel: w1409 -> [w1439]
          tunnel: [w1439] -> w1408
          tunnel: w1407 -> [w1438]
          tunnel: [w1438] -> w1406
          tunnel: [w1437] -> w1405
          tunnel: w1421 -> [w1451]
          tunnel: [w1459] -> w1420
          tunnel: [w1456] -> w1419
          tunnel: [w1455] -> w1418
          tunnel: [w1454] -> w1417
          tunnel: w1410 -> [w1450]
          tunnel: w1408 -> [w1449]
          tunnel: w1406 -> [w1448]
          tunnel: w1405 -> [w1442]
          tunnel: [w1444] -> w1404
          tunnel: w1420 -> [w1466]
          tunnel: [w1467] -> w1416
          tunnel: w1419 -> [w1467]
          tunnel: w1418 -> [w1465]
          tunnel: w1417 -> [w1464]
          tunnel: [w1463] -> w1415
          tunnel: [w1462] -> w1414
          tunnel: w1404 -> [w1461]
          tunnel: [w1461] -> w1403
          tunnel: [w1474] -> w1413
          tunnel: w1416 -> [w1474]
          tunnel: w1415 -> [w1473]
          tunnel: [w1473] -> w1412
          tunnel: [w1472] -> w1411
          tunnel: w1414 -> [w1472]
          tunnel: w1403 -> [w1470]
          tunnel: [w1470] -> w1402
          tunnel: w1413 -> [w1477]
          tunnel: w1412 -> [w1485]
          tunnel: w1411 -> [w1484]
          tunnel: w1402 -> [w1476]
          tunnel: [w1476] -> w1401
          tunnel: w1401 -> [w1493]
          tunnel: [w1493] -> w1400
          tunnel: w1400 -> [w1495]
          frame #0 {
            n833 = local read "产品ID"() -> (w1432:string)
            n834 = Format Date/Time String(time format string (%c)="%Y%m%d" ("时间格式字符串(%c)")) -> (date/time string=w1426:string)  [unwired: 2 in]
            n835 = String Subset(string=w1426, offset (0)=4 ("偏移量(0)"), length (rest)=2 ("长度（剩余）")) -> (substring=w1425:string)
            n836 = String Subset(string=w1426, offset (0)=6 ("偏移量(0)"), length (rest)=2 ("长度（剩余）")) -> (substring=w1424:string)
            n837 = call <vilib>:"Trim Whitespace.vi"("string"=w1432) -> ("trimmed string"=w1431:string)  [unwired: 1 in]
            n838 = String Subset(string=w1426, offset (0)=0 ("偏移量(0)"), length (rest)=4 ("长度（剩余）")) -> (substring=w1433:string)
          }
          frame #1 {
          }
          frame #2 {
            w1443 = "\\" ("字符串")
            n839 = Concatenate Strings(w1451, w1450, w1443, w1449, w1443, w1448, w1443, w1442, w1443) -> (w1446:string)
            n840 = Concatenate Strings(w1451, w1450, w1443, w1449, w1443, w1448, w1443, w1442, w1443) -> (w1460:string)
            n841 = String To Path(string=w1460) -> (path=w1459:path)
            n842 = Concatenate Strings(w1446, w1442, "间隙曲线.JPG" ("字符串")) -> (w1457:string)
            n843 = Concatenate Strings(w1446, "轴向力曲线数组.txt" ("字符串")) -> (w1454:string)
            n844 = Concatenate Strings(w1446, "扭动曲线数组.txt" ("字符串")) -> (w1455:string)
            n845 = Concatenate Strings(w1446, w1442, "轴向力曲线.JPG" ("字符串")) -> (w1447:string)
            n846 = String To Path(string=w1457) -> (path=w1456:path)
            n847 = String To Path(string=w1447) -> (path=w1444:path)
          }
          frame #3 {
            n848 = call <vilib>:"Check if File or Folder Exists.vi"("path"=w1466) -> ("file or folder exists?"=w1468:bool)  [unwired: 8 in, 2 out]
            n849 = String To Path(string=w1464) -> (path=w1462:path)
            n850 = String To Path(string=w1465) -> (path=w1463:path)
            n851 = case shown="假" w1468 {
              tunnel: w1466 -> [w1469 _]
              frame False {
                n852 = Create Folder(path (use dialog)=w1469) -> ()  [unwired: 2 in, 3 out]
              }
              frame True {
              }
            }
          }
          frame #4 {
            n853 = local write "选项卡控件"(T1."间隙测量" ("选项卡控件")) -> ()
            n854 = Wait Until Next ms Multiple(millisecond multiple=u32 1000 ("毫秒倍数")) -> ()  [unwired: 1 out]
          }
          frame #5 {
            n855 = disable-structure shown="禁用" {
              disable-tunnel: w1477 -> [w1486 _]
              frame Disabled {
                w1490 = T3 2 items=["快速打印", "标准报表", "HTML", "双字节", "Excel"] ("report type (Quick Print)")
                w1489 = T4 1 items=["完整前面板", "前面板可见部分", "图标、说明、前面板和程序框图", "说明信息: 使用前面板", "说明信息: 作为子VI使用", "说明信息: 完整", "说明信息: 自定义"] ("contents (complete front panel)")
                n856 = Current VI's Path() -> (path=w1488:path)
                n857 = call-poly <vilib>:"Easy Print VI Panel or Documentation.vi"("report type (Quick Print)"=w1490, "contents (complete front panel)"=w1489, "VI path"=w1488) -> ("error out"=w1492:errorcluster, "report out"=w1491:refnum<class "NI_report.lvclass">)  [unwired: 1 in, 6 out]
                n858 = call-dynamic "Save Report to File.vi"("report in"=w1491, "report file path"=w1486, "error in (no error)"=w1492) -> ("error out"=→"error out 3":errorcluster)  [unwired: 2 in, 10 out]
              }
              frame Enabled {
              }
            }
            n859 = local read "间隙Y数组"() -> (w1482:dbl[])
            n860 = local read "间隙X数组"() -> (w1483:dbl[])
            n861 = local read "轴向力Y"() -> (w1480:dbl[])
            n862 = local read "轴向力X"() -> (w1481:dbl[])
            n863 = call "导出曲线数组.vi"("file path (dialog if empty)"=w1485, "数组 2"=w1482, "数组"=w1483) -> ()  [unwired: 9 in]
            n864 = call "导出曲线数组.vi"("file path (dialog if empty)"=w1484, "数组 2"=w1480, "数组"=w1481) -> ()  [unwired: 9 in]
            n865 = control-ref of="本VI"() -> (w1479:refnum<vi>)
            n866 = invoke class="VI" method="FP.Get Image"(reference=w1479) -> ("image data"=w1478:T5)  [unwired: 5 in, 5 out]
            n867 = call <vilib>:"Write JPEG File.vi"("image data"=w1478, "path to JPEG file"=w1477) -> ()  [unwired: 8 in, 2 out]
          }
          frame #6 {
            n868 = local write "选项卡控件"(T1."轴向力测量" ("选项卡控件")) -> ()
          }
          frame #7 {
            n869 = control-ref of="本VI"() -> (w1496:refnum<vi>)
            n870 = invoke class="VI" method="FP.Get Image"(reference=w1496) -> ("image data"=w1497:T5)  [unwired: 5 in, 5 out]
            n871 = call <vilib>:"Write JPEG File.vi"("image data"=w1497, "path to JPEG file"=w1495) -> ()  [unwired: 8 in, 2 out]
          }
          frame #8 {
            n872 = local read "联线按钮"() -> (w1498:bool)
            n873 = case shown="真" w1498 {
              frame False {
              }
              frame True {
                n874 = flat-sequence {
                  tunnel: [w1525] -> w1499
                  tunnel: w1499 -> [w1540]
                  frame #0 {
                    w1518 = i16 3 ("精度(6)")
                    n875 = local read "全行程间隙及轴向力合格"() -> (w1520:bool)
                    n876 = local read "左180°外全行程间隙"() -> (w1517:dbl)
                    n877 = local read "右180°内全行程间隙"() -> (w1519:dbl)
                    n878 = local read "右180°外全行程间隙"() -> (w1516:dbl)
                    n879 = local read "左最大轴向力(N)"() -> (w1515:dbl)
                    n880 = local read "右最大轴向力(N)"() -> (w1514:dbl)
                    n881 = local read "左轴向力波动(N)"() -> (w1513:dbl)
                    n882 = local read "单点间隙合格"() -> (w1521:bool)
                    n883 = local read "右轴向力波动(N)"() -> (w1512:dbl)
                    n884 = local read "左180°内全行程间隙"() -> (w1528:dbl)
                    n885 = local read "总行程(mm)"() -> (w1511:dbl)
                    n886 = local read "总圈数"() -> (w1510:dbl)
                    n887 = local read "员工ID"() -> (w1500:string)
                    n888 = local read "中间位置间隙"() -> (w1530:dbl)
                    n889 = local read "FGCS"() -> (w1532:string)
                    n890 = And(x=w1521, y=w1520) -> (x .and. y?=w1522:bool)
                    n891 = local read "KSJJ"() -> (w1534:string)
                    n892 = local read "产品ID"() -> (w1537:string)
                    n893 = Boolean To (0,1)(Boolean=w1522) -> (0, 1=w1536:i16)
                    n894 = Number To Fractional String(number=w1511, precision (6)=w1518) -> (F-format string=w1502:string)  [unwired: 2 in]
                    n895 = Number To Fractional String(number=w1513, precision (6)=w1518) -> (F-format string=w1504:string)  [unwired: 2 in]
                    n896 = Number To Fractional String(number=w1512, precision (6)=w1518) -> (F-format string=w1503:string)  [unwired: 2 in]
                    n897 = Number To Fractional String(number=w1519, precision (6)=w1518) -> (F-format string=w1509:string)  [unwired: 2 in]
                    n898 = Number To Fractional String(number=w1517, precision (6)=w1518) -> (F-format string=w1508:string)  [unwired: 2 in]
                    n899 = Number To Fractional String(number=w1510, precision (6)=w1518) -> (F-format string=w1501:string)  [unwired: 2 in]
                    n900 = Number To Fractional String(number=w1528, precision (6)=w1518) -> (F-format string=w1526:string)  [unwired: 2 in]
                    n901 = Number To Fractional String(number=w1514, precision (6)=w1518) -> (F-format string=w1505:string)  [unwired: 2 in]
                    n902 = Number To Fractional String(number=w1516, precision (6)=w1518) -> (F-format string=w1507:string)  [unwired: 2 in]
                    n903 = Number To Fractional String(number=w1515, precision (6)=w1518) -> (F-format string=w1506:string)  [unwired: 2 in]
                    n904 = Number To Fractional String(number=w1530, precision (6)=i16 3 ("精度(6)")) -> (F-format string=w1527:string)  [unwired: 2 in]
                    n905 = Format Date/Time String(time format string (%c)="%Y%m%d%H%M" ("时间格式字符串(%c)")) -> (date/time string=w1533:string)  [unwired: 2 in]
                    n906 = Number To Decimal String(number=w1536, width (-)=i16 1 ("宽度(-)")) -> (decimal integer string=w1523:string)
                    n907 = Build Array(w1537, w1500, "1", w1523, w1534, w1533, w1532, "Q14070-Z060A", w1527, w1526, w1509, w1508, w1507, w1506, w1505, w1504, w1503, w1502, w1501) -> (w1525:string[])
                  }
                  frame #1 {
                    n908 = Wait (ms)(milliseconds to wait=u32 500 ("等待时间（毫秒）")) -> ()  [unwired: 1 out]
                    n909 = call "数据库更新.vi"("设备号"="06", "数据"=w1540) -> ()  [unwired: 13 in, 1 out]
                  }
                  frame #2 {
                  }
                }
              }
            }
          }
          frame #9 {
            n910 = local write "产品ID"("") -> ()
            n911 = local write "工步号"(u32 0 ("工步号")) -> ()
          }
        }
      }
    }
    n912 = Wait (ms)(milliseconds to wait=u32 50 ("毫秒倍数")) -> ()  [unwired: 1 out]
    n913 = local read "停止"() -> (w178:bool)
  }
  n914 = call "PCI1240电动缸位置模式 .vi"() -> ()  [unwired: 10 in, 2 out]
  n915 = while {
    stop <- w1545 stop-if-true
    n916 = stacked-sequence {
      frame #0 {
        n917 = flat-sequence {
          frame #0 {
          }
          frame #1 {
            n918 = First Call?() -> (First Call?: T/F=w1546:bool)
            n919 = case shown="真" w1546 {
              frame False {
              }
              frame True {
                n920 = call "员工管理测试程序.vi"() -> ("员工姓名"=w1548:string, "员工ID"=w1547:string)  [unwired: 10 in]
                n921 = local write "员工ID"(w1547) -> ()
                n922 = local write "员工姓名"(w1548) -> ()
              }
            }
          }
          frame #2 {
          }
          frame #3 {
          }
          frame #4 {
          }
          frame #5 {
          }
          frame #6 {
          }
        }
      }
      frame #1 {
        n923 = flat-sequence {
          frame #0 {
            n924 = property on="型号选择" class="Ring (严格)"() -> ("RingText.Text"=w1552:string)  [unwired: 2 in, 2 out]
            n925 = case shown="\"J706\"" w1552 {
              frame "J706" {
                w1553 = FALSE ("可见")
                w1554 = TRUE ("可见")
                n926 = property on="左180°内全行程间隙" class="DigNum (严格)"("Visible"=w1554) -> ()  [unwired: 2 in, 2 out]
                n927 = property on="左180°外全行程间隙" class="DigNum (严格)"("Visible"=w1554) -> ()  [unwired: 2 in, 2 out]
                n928 = property on="右180°外全行程间隙" class="DigNum (严格)"("Visible"=w1554) -> ()  [unwired: 2 in, 2 out]
                n929 = property on="右180°内全行程间隙" class="DigNum (严格)"("Visible"=w1554) -> ()  [unwired: 2 in, 2 out]
                n930 = property on="左全行程间隙" class="DigNum (严格)"("Visible"=w1553) -> ()  [unwired: 2 in, 2 out]
                n931 = property on="右全行程间隙" class="DigNum (严格)"("Visible"=w1553) -> ()  [unwired: 2 in, 2 out]
              }
              frame "J728" {
                w1555 = FALSE ("可见")
                w1556 = TRUE ("可见")
                n932 = property on="左180°内全行程间隙" class="DigNum (严格)"("Visible"=w1556) -> ()  [unwired: 2 in, 2 out]
                n933 = property on="左180°外全行程间隙" class="DigNum (严格)"("Visible"=w1556) -> ()  [unwired: 2 in, 2 out]
                n934 = property on="右180°外全行程间隙" class="DigNum (严格)"("Visible"=w1556) -> ()  [unwired: 2 in, 2 out]
                n935 = property on="右180°内全行程间隙" class="DigNum (严格)"("Visible"=w1556) -> ()  [unwired: 2 in, 2 out]
                n936 = property on="左全行程间隙" class="DigNum (严格)"("Visible"=w1555) -> ()  [unwired: 2 in, 2 out]
                n937 = property on="右全行程间隙" class="DigNum (严格)"("Visible"=w1555) -> ()  [unwired: 2 in, 2 out]
              }
              frame "J709", Default {
                w1557 = TRUE ("可见")
                w1558 = FALSE ("可见")
                n938 = property on="左180°内全行程间隙" class="DigNum (严格)"("Visible"=w1558) -> ()  [unwired: 2 in, 2 out]
                n939 = property on="左180°外全行程间隙" class="DigNum (严格)"("Visible"=w1558) -> ()  [unwired: 2 in, 2 out]
                n940 = property on="右180°外全行程间隙" class="DigNum (严格)"("Visible"=w1558) -> ()  [unwired: 2 in, 2 out]
                n941 = property on="右180°内全行程间隙" class="DigNum (严格)"("Visible"=w1558) -> ()  [unwired: 2 in, 2 out]
                n942 = property on="左全行程间隙" class="DigNum (严格)"("Visible"=w1557) -> ()  [unwired: 2 in, 2 out]
                n943 = property on="右全行程间隙" class="DigNum (严格)"("Visible"=w1557) -> ()  [unwired: 2 in, 2 out]
              }
            }
          }
          frame #1 {
            (unwired) string[] ["I急停按钮", "I自动旋钮", "I启动按钮", "I备用按钮", "I复位按钮", "I上阻挡器放行", "I下阻挡器放行", "I进支线按钮"] ("I0说明")
            (unwired) string[] ["I出支线按钮", "I主线顶升按钮", "I主线下降按钮", "I支线顶升按钮", "I支线下降按钮", "I气压报警", "未使用", "未使用"] ("I0说明")
            n944 = local read "间隙位移(mm)"() -> (w1561:dbl)
            n945 = Greater Or Equal?(x=w1561, y=7.0) -> (x >= y?=w1559:bool)
            n946 = case shown="真" w1559 {
              frame False {
              }
              frame True {
                n947 = local write "测头机构轴使能"(FALSE ("测头机构轴使能")) -> ()
              }
            }
          }
          frame #2 {
            (unwired) string[] ["I电动缸SRDY", "I电动缸ZSPD", "I电动缸ALRM", "I间隙进给SRDY", "I间隙进给ZSPD", "I间隙进给ALRM", "I间隙旋转SRPD", "I间隙旋转ZSPD"] ("I0说明")
            n948 = local read "测头机构轴位置(mm)"() -> (w1565:dbl)
            n949 = Greater Or Equal?(x=w1565, y=90.0) -> (x >= y?=w1563:bool)
            n950 = case shown="假" w1563 {
              frame False {
                w1566 = T2."Enabled" ("禁用")
                n951 = property on="测头气缸左移" class="Bool (严格)"("DisabledEnum"=w1566) -> ()  [unwired: 2 in, 2 out]
                n952 = property on="测头气缸右移" class="Bool (严格)"("DisabledEnum"=w1566) -> ()  [unwired: 2 in, 2 out]
                n953 = property on="测头气缸左移" class="Bool"("DisabledEnum"=w1566) -> ()  [unwired: 2 in, 2 out]
                n954 = property on="测头气缸右移" class="Bool"("DisabledEnum"=w1566) -> ()  [unwired: 2 in, 2 out]
              }
              frame True {
                w1567 = T2."Disabled" ("禁用")
                w1568 = FALSE ("测头气缸右移")
                n955 = local write "测头气缸右移"(w1568) -> ()
                n956 = local write "测头气缸左移"(w1568) -> ()
                n957 = property on="测头气缸左移" class="Bool (严格)"("DisabledEnum"=w1567) -> ()  [unwired: 2 in, 2 out]
                n958 = property on="测头气缸右移" class="Bool (严格)"("DisabledEnum"=w1567) -> ()  [unwired: 2 in, 2 out]
                n959 = property on="测头气缸左移" class="Bool"("DisabledEnum"=w1567) -> ()  [unwired: 2 in, 2 out]
                n960 = property on="测头气缸右移" class="Bool"("DisabledEnum"=w1567) -> ()  [unwired: 2 in, 2 out]
              }
            }
          }
          frame #3 {
            (unwired) string[] ["I间隙旋转ALRM", "I扭矩旋转SRPD", "I扭矩旋转ZSPD", "I扭矩旋转ALRM", "I拧紧机合格", "I拧紧机不合格", "I拧紧机报警", "未使用"] ("I0说明")
          }
        }
        n961 = local read "急停"() -> (w1551:bool)
        n962 = local read "复位"() -> (w1550:bool)
        n963 = Compound Arithmetic op=OR(invert w1551, w1550) -> (→"循环退出":bool)
      }
      frame #2 {
        n964 = flat-sequence {
          frame #0 {
            (unwired) string[] ["I自制气缸进位", "I自制气缸原位", "I上工位检测", "I本工位检测", "I下工位检测", "I主线顶升上位", "I主线顶升下位", "I支线顶升上位"] ("I0说明")
          }
          frame #1 {
            (unwired) string[] ["I支线顶升下位", "I支线进到位", "I支线退到位", "I位移气缸原位", "I位移气缸进位", "I拧紧机在位", "I电动缸原位", "I电动缸进位"] ("I0说明")
          }
          frame #2 {
            (unwired) string[] ["未使用", "未使用", "未使用", "未使用", "未使用", "未使用", "未使用", "未使用"] ("I0说明")
          }
          frame #3 {
            (unwired) string[] ["未使用", "未使用", "未使用", "未使用", "未使用", "未使用", "未使用", "未使用"] ("I0说明")
          }
        }
        n965 = local read "下工位测试H"() -> (w1570:bool)
        n966 = local read "下工位备料H"() -> (w1569:bool)
        n967 = local read "下工位自动H"() -> (w1571:bool)
        n968 = local write "下工位备料"(w1569) -> ()
        n969 = local write "下工位测试"(w1570) -> ()
        n970 = local write "下工位自动"(w1571) -> ()
      }
      frame #3 {
        n971 = local read "工步号"() -> (w1575:u32)
        n972 = local read "报警"() -> (w1573:dbl)
        n973 = case shown="50" w1575 {
          tunnel: [w1586 "请取胶瓶" ("工步描述") "请取扳手加力" ("工步描述") "灵敏度测试中" ("工步描述") "有油刚度测试中" ("工步描述") "点击启动按钮进行测试" ("工步描述") "电动缸前进找中" ("工步描述") "气缸右移" ("工步描述") "电动缸前进找中" ("工步描述") "找中结束开始测间隙" ("工步描述") "力特性试验中" ("工步描述") "轴向力测试中" ("工步描述") "探头气缸左移，电动缸后退" ("工步描述") "等待放行" ("工步描述") "电动缸回零" ("工步描述") "力特性试验完成" ("工步描述") "套好输出轴把手，按启动按钮，做回正力试验" ("工步描述") "回正力试验中" ("工步描述") "试验完成，将把手拉回，取下油管，按顶升按钮" ("工步描述") "拆下锁紧螺母和输入轴万向节，按顶升按钮" ("工步描述")] -> w1574
          frame 0, Default {
            n974 = local read "联线按钮"() -> (w1585:bool)
            n975 = case shown="假" w1585 {
              tunnel: ["等待工件" ("工步描述") "等待扫描条码" ("工步描述")] -> w1586
              frame False {
              }
              frame True {
              }
            }
          }
          frame 1 {
          }
          frame 2 {
          }
          frame 3 {
          }
          frame 4 {
          }
          frame 6 {
          }
          frame 7 {
          }
          frame 10 {
          }
          frame 15 {
          }
          frame 20 {
          }
          frame 30 {
          }
          frame 40 {
          }
          frame 45 {
          }
          frame 100 {
          }
          frame 50 {
          }
          frame 55 {
          }
          frame 60 {
          }
          frame 70 {
          }
          frame 80 {
          }
          frame 56 {
          }
        }
        "工步提示" <- w1574
        n976 = case shown="9" w1573 {
          tunnel: [_ "探头气缸不在原位" "操作步骤错误请取胶瓶" "操作步骤错误请加力" "急停被按下" "气压报警" "电动缸伺服报警" "旋转伺服报警" "测头伺服报警" "操作步骤错误请点标后放行"] -> w1572
          frame 0, Default {
          }
          frame 1 {
          }
          frame 2 {
          }
          frame 3 {
          }
          frame 4 {
          }
          frame 5 {
          }
          frame 6 {
          }
          frame 7 {
          }
          frame 8 {
          }
          frame 9 {
          }
        }
        n977 = local write "报警提示"(w1572) -> ()
      }
      frame #4 {
        n978 = local read "急停"() -> (w1608:bool)
        n979 = local read "红灯"() -> (w1610:bool)
        n980 = local read "复位"() -> (w1611:bool)
        n981 = local read "复位"() -> (w1613:bool)
        n982 = local read "红灯"() -> (w1612:bool)
        n983 = case shown="真" w1608 {
          frame False {
            "红灯" <- TRUE ("红灯")
          }
          frame True {
            n984 = local write "红灯"(FALSE ("红灯")) -> ()
          }
        }
        n985 = Or(x=w1610, y=w1611) -> (x .or. y?=w1609:bool)
        n986 = case shown="真" w1609 {
          frame False {
          }
          frame True {
            n987 = local write "回零完成"(FALSE ("夹头夹紧控制")) -> ()
          }
        }
        n988 = local read "停止"() -> (w1615:bool)
        n989 = Compound Arithmetic op=OR(w1613, w1615, w1612) -> (w1614:bool)
        n990 = case shown="真" w1614 {
          frame False {
          }
          frame True {
            n991 = local read "测头机构电机"() -> (w1619:u32)
            n992 = local read "旋转齿条电机"() -> (w1620:u32)
            n993 = local read "电动缸电机"() -> (w1621:u32)
            n994 = call "PCI1220U停止.vi"("AxisHandle IN"=w1620) -> ()  [unwired: 9 in, 2 out]
            n995 = call "PCI1220U停止.vi"("AxisHandle IN"=w1621) -> ()  [unwired: 9 in, 2 out]
            n996 = call "PCI1220U停止.vi"("AxisHandle IN"=w1619) -> ()  [unwired: 9 in, 2 out]
          }
        }
      }
      frame #5 {
        n997 = local read "齿条扭矩(Nm)"() -> (w1624:dbl)
        n998 = local read "黄灯"() -> (w1622:bool)
        n999 = local read "旋转齿条轴左转"() -> (w1630:bool)
        n1000 = Absolute Value(x=w1624) -> (abs(x)=w1629:dbl)
        n1001 = local read "旋转齿条轴右转"() -> (w1625:bool)
        n1002 = Not(x=w1630) -> (.not. x?=w1626:bool)
        n1003 = Less?(x=w1629, y=20.0) -> (x < y?=w1627:bool)
        n1004 = Compound Arithmetic op=AND(w1625, w1626, w1627, w1622) -> (w1623:bool)
        n1005 = case shown="真" w1623 {
          frame False {
          }
          frame True {
            n1006 = flat-sequence {
              tunnel: [w1634] -> w1632
              tunnel: w1632 -> [w1636]
              tunnel: [w1636] -> w1631
              tunnel: w1631 -> [w1647]
              frame #0 {
                n1007 = local read "旋转齿条电机"() -> (w1633:u32)
                n1008 = call "PCI1220U运行.vi"("方向"=enum32{"Negative", "Positive"}."Negative" ("Direction"), "AxisHandle IN"=w1633) -> ("AxisHandle OUT"=w1634:u32)  [unwired: 9 in]
              }
              frame #1 {
                n1009 = while {
                  stop <- w1640 stop-if-true
                  n1010 = Wait (ms)(milliseconds to wait=u32 50 ("毫秒倍数")) -> ()  [unwired: 1 out]
                  n1011 = local read "齿条扭矩(Nm)"() -> (w1645:dbl)
                  n1012 = local read "旋转齿条轴右转"() -> (w1642:bool)
                  n1013 = local read "红灯"() -> (w1637:bool)
                  n1014 = local read "复位"() -> (w1638:bool)
                  n1015 = Absolute Value(x=w1645) -> (abs(x)=w1644:dbl)
                  n1016 = Not(x=w1642) -> (.not. x?=w1639:bool)
                  n1017 = Greater?(x=w1644, y=10.0) -> (0:w1641:bool)
                  n1018 = Compound Arithmetic op=OR(w1641, w1639, w1638, w1637) -> (w1640:bool)
                }
              }
              frame #2 {
                n1019 = call "PCI1220U停止.vi"("AxisHandle IN"=w1647) -> ()  [unwired: 9 in, 2 out]
              }
            }
          }
        }
      }
      frame #6 {
        n1020 = local read "齿条扭矩(Nm)"() -> (w1652:dbl)
        n1021 = local read "旋转齿条轴右转"() -> (w1656:bool)
        n1022 = Absolute Value(x=w1652) -> (abs(x)=w1651:dbl)
        n1023 = local read "旋转齿条轴左转"() -> (w1654:bool)
        n1024 = local read "黄灯"() -> (w1648:bool)
        n1025 = Not(x=w1656) -> (.not. x?=w1653:bool)
        n1026 = Less?(x=w1651, y=20.0) -> (x < y?=w1649:bool)
        n1027 = Compound Arithmetic op=AND(w1654, w1653, w1649, w1648) -> (w1655:bool)
        n1028 = case shown="真" w1655 {
          frame False {
          }
          frame True {
            n1029 = flat-sequence {
              tunnel: [w1660] -> w1658
              tunnel: w1658 -> [w1662]
              tunnel: [w1662] -> w1657
              tunnel: w1657 -> [w1673]
              frame #0 {
                n1030 = local read "旋转齿条电机"() -> (w1659:u32)
                n1031 = call "PCI1220U运行.vi"("方向"=enum32{"Negative", "Positive"}."Positive" ("Direction"), "AxisHandle IN"=w1659) -> ("AxisHandle OUT"=w1660:u32)  [unwired: 9 in]
              }
              frame #1 {
                n1032 = while {
                  stop <- w1665 stop-if-true
                  n1033 = Wait (ms)(milliseconds to wait=u32 50 ("毫秒倍数")) -> ()  [unwired: 1 out]
                  n1034 = local read "齿条扭矩(Nm)"() -> (w1671:dbl)
                  n1035 = local read "旋转齿条轴左转"() -> (w1668:bool)
                  n1036 = local read "红灯"() -> (w1663:bool)
                  n1037 = local read "复位"() -> (w1664:bool)
                  n1038 = Absolute Value(x=w1671) -> (abs(x)=w1670:dbl)
                  n1039 = Not(x=w1668) -> (.not. x?=w1666:bool)
                  n1040 = Greater?(x=w1670, y=10.0) -> (0:w1667:bool)
                  n1041 = Compound Arithmetic op=OR(w1664, w1663, w1667, w1666) -> (w1665:bool)
                }
              }
              frame #2 {
                n1042 = call "PCI1220U停止.vi"("AxisHandle IN"=w1673) -> ()  [unwired: 9 in, 2 out]
              }
            }
          }
        }
      }
      frame #7 {
        n1043 = local read "齿条推拉力(N)"() -> (w1678:dbl)
        n1044 = local read "电动缸前进"() -> (w1675:bool)
        n1045 = local read "电动缸后退"() -> (w1674:bool)
        n1046 = Absolute Value(x=w1678) -> (abs(x)=w1682:dbl)
        n1047 = local read "黄灯"() -> (w1676:bool)
        n1048 = Not(x=w1674) -> (.not. x?=w1679:bool)
        n1049 = Less?(x=w1682, y=1000.0) -> (x < y?=w1680:bool)
        n1050 = Compound Arithmetic op=AND(w1675, w1679, w1676, w1680) -> (w1677:bool)
        n1051 = case shown="真" w1677 {
          frame False {
          }
          frame True {
            n1052 = flat-sequence {
              tunnel: [w1686] -> w1684
              tunnel: w1684 -> [w1688]
              tunnel: [w1688] -> w1683
              tunnel: w1683 -> [w1699]
              frame #0 {
                n1053 = local read "电动缸电机"() -> (w1685:u32)
                n1054 = call "PCI1220U运行.vi"("方向"=enum32{"Negative", "Positive"}."Positive" ("Direction"), "AxisHandle IN"=w1685) -> ("AxisHandle OUT"=w1686:u32)  [unwired: 9 in]
              }
              frame #1 {
                n1055 = while {
                  stop <- w1696 stop-if-true
                  n1056 = local read "电动缸前进"() -> (w1693:bool)
                  n1057 = local read "齿条推拉力(N)"() -> (w1690:dbl)
                  n1058 = Wait (ms)(milliseconds to wait=u32 50 ("毫秒倍数")) -> ()  [unwired: 1 out]
                  n1059 = Absolute Value(x=w1690) -> (abs(x)=w1692:dbl)
                  n1060 = local read "红灯"() -> (w1694:bool)
                  n1061 = local read "复位"() -> (w1695:bool)
                  n1062 = Greater?(x=w1692, y=1000.0) -> (0:w1689:bool)
                  n1063 = Not(x=w1693) -> (.not. x?=w1697:bool)
                  n1064 = Compound Arithmetic op=OR(w1695, w1694, w1697, w1689) -> (w1696:bool)
                }
              }
              frame #2 {
                n1065 = call "PCI1220U停止.vi"("AxisHandle IN"=w1699) -> ()  [unwired: 9 in, 2 out]
              }
            }
          }
        }
      }
      frame #8 {
        n1066 = local read "电动缸前进"() -> (w1700:bool)
        n1067 = local read "齿条推拉力(N)"() -> (w1704:dbl)
        n1068 = local read "电动缸后退"() -> (w1701:bool)
        n1069 = Absolute Value(x=w1704) -> (abs(x)=w1708:dbl)
        n1070 = local read "黄灯"() -> (w1702:bool)
        n1071 = Not(x=w1700) -> (.not. x?=w1705:bool)
        n1072 = Less?(x=w1708, y=1000.0) -> (x < y?=w1706:bool)
        n1073 = Compound Arithmetic op=AND(w1701, w1705, w1702, w1706) -> (w1703:bool)
        n1074 = case shown="真" w1703 {
          frame False {
          }
          frame True {
            n1075 = flat-sequence {
              tunnel: [w1712] -> w1710
              tunnel: w1710 -> [w1714]
              tunnel: [w1714] -> w1709
              tunnel: w1709 -> [w1725]
              frame #0 {
                n1076 = local read "电动缸电机"() -> (w1711:u32)
                n1077 = call "PCI1220U运行.vi"("方向"=enum32{"Negative", "Positive"}."Negative" ("Direction"), "AxisHandle IN"=w1711) -> ("AxisHandle OUT"=w1712:u32)  [unwired: 9 in]
              }
              frame #1 {
                n1078 = while {
                  stop <- w1722 stop-if-true
                  n1079 = local read "电动缸后退"() -> (w1719:bool)
                  n1080 = local read "齿条推拉力(N)"() -> (w1718:dbl)
                  n1081 = Wait (ms)(milliseconds to wait=u32 50 ("毫秒倍数")) -> ()  [unwired: 1 out]
                  n1082 = Absolute Value(x=w1718) -> (abs(x)=w1716:dbl)
                  n1083 = local read "红灯"() -> (w1721:bool)
                  n1084 = local read "复位"() -> (w1720:bool)
                  n1085 = Greater?(x=w1716, y=1000.0) -> (0:w1715:bool)
                  n1086 = Not(x=w1719) -> (.not. x?=w1723:bool)
                  n1087 = Compound Arithmetic op=OR(w1720, w1721, w1723, w1715) -> (w1722:bool)
                }
              }
              frame #2 {
                n1088 = call "PCI1220U停止.vi"("AxisHandle IN"=w1725) -> ()  [unwired: 9 in, 2 out]
              }
            }
          }
        }
      }
      frame #9 {
        n1089 = local read "测头机构轴后退"() -> (w1726:bool)
        n1090 = local read "测头机构轴前进"() -> (w1727:bool)
        n1091 = local read "黄灯"() -> (w1728:bool)
        n1092 = Not(x=w1726) -> (.not. x?=w1730:bool)
        n1093 = Compound Arithmetic op=AND(w1727, w1730, w1728) -> (w1729:bool)
        n1094 = case shown="真" w1729 {
          frame False {
          }
          frame True {
            n1095 = flat-sequence {
              tunnel: [w1734] -> w1732
              tunnel: w1732 -> [w1736]
              tunnel: [w1736] -> w1731
              tunnel: w1731 -> [w1743]
              frame #0 {
                n1096 = local read "测头机构电机"() -> (w1733:u32)
                n1097 = call "PCI1220U运行.vi"("方向"=enum32{"Negative", "Positive"}."Positive" ("Direction"), "AxisHandle IN"=w1733) -> ("AxisHandle OUT"=w1734:u32)  [unwired: 9 in]
              }
              frame #1 {
                n1098 = while {
                  stop <- w1740 stop-if-true
                  n1099 = local read "测头机构轴前进"() -> (w1737:bool)
                  n1100 = Wait (ms)(milliseconds to wait=u32 50 ("毫秒倍数")) -> ()  [unwired: 1 out]
                  n1101 = local read "红灯"() -> (w1738:bool)
                  n1102 = local read "复位"() -> (w1739:bool)
                  n1103 = Not(x=w1737) -> (.not. x?=w1741:bool)
                  n1104 = Compound Arithmetic op=OR(w1739, w1738, w1741) -> (w1740:bool)
                }
              }
              frame #2 {
                n1105 = call "PCI1220U停止.vi"("AxisHandle IN"=w1743) -> ()  [unwired: 9 in, 2 out]
              }
            }
          }
        }
      }
      frame #10 {
        n1106 = local read "测头机构轴前进"() -> (w1744:bool)
        n1107 = local read "测头机构轴后退"() -> (w1745:bool)
        n1108 = local read "黄灯"() -> (w1746:bool)
        n1109 = Not(x=w1744) -> (.not. x?=w1748:bool)
        n1110 = Compound Arithmetic op=AND(w1745, w1748, w1746) -> (w1747:bool)
        n1111 = case shown="真" w1747 {
          frame False {
          }
          frame True {
            n1112 = flat-sequence {
              tunnel: [w1752] -> w1750
              tunnel: w1750 -> [w1754]
              tunnel: [w1754] -> w1749
              tunnel: w1749 -> [w1761]
              frame #0 {
                n1113 = local read "测头机构电机"() -> (w1751:u32)
                n1114 = call "PCI1220U运行.vi"("方向"=enum32{"Negative", "Positive"}."Negative" ("Direction"), "AxisHandle IN"=w1751) -> ("AxisHandle OUT"=w1752:u32)  [unwired: 9 in]
              }
              frame #1 {
                n1115 = while {
                  stop <- w1758 stop-if-true
                  n1116 = local read "测头机构轴后退"() -> (w1755:bool)
                  n1117 = Wait (ms)(milliseconds to wait=u32 50 ("毫秒倍数")) -> ()  [unwired: 1 out]
                  n1118 = local read "红灯"() -> (w1757:bool)
                  n1119 = local read "复位"() -> (w1756:bool)
                  n1120 = Not(x=w1755) -> (.not. x?=w1759:bool)
                  n1121 = Compound Arithmetic op=OR(w1756, w1757, w1759) -> (w1758:bool)
                }
              }
              frame #2 {
                n1122 = call "PCI1220U停止.vi"("AxisHandle IN"=w1761) -> ()  [unwired: 9 in, 2 out]
              }
            }
          }
        }
      }
      frame #11 {
        n1123 = local read "电动缸回零"() -> (w1762:bool)
        n1124 = case shown="真" w1762 {
          frame False {
          }
          frame True {
            n1125 = stacked-sequence {
              frame #0 {
                n1126 = flat-sequence {
                  tunnel: [w1780] -> w1769
                  tunnel: [w1773] -> w1766
                  tunnel: w1769 -> [w1783]
                  tunnel: [w1783] -> w1768
                  tunnel: [w1781] -> w1767
                  tunnel: w1766 -> [w1781]
                  tunnel: w1768 -> [w1785]
                  tunnel: [w1785] -> w1770
                  tunnel: w1767 -> [w1784]
                  tunnel: [w1784] -> w1765
                  tunnel: w1770 -> [w1796]
                  tunnel: w1765 -> [w1795]
                  tunnel: [w1794] -> w1764
                  tunnel: w1764 -> [w1798]
                  tunnel: [w1797] -> w1763
                  tunnel: w1763 -> [w1806]
                  frame #0 {
                    n1127 = local write "测头机构轴速度(mm/s)"(10.0 ("电动缸速度(mm/s)")) -> ()
                    n1128 = local write "电动缸速度(mm/s)"(15.0 ("电动缸速度(mm/s)")) -> ()
                  }
                  frame #1 {
                    n1129 = local read "测头机构电机"() -> (w1777:u32)
                    n1130 = local read "电动缸电机"() -> (w1774:u32)
                    n1131 = call <userlib>:"Acm_AxHome.vi"("DirMode"=u32 0, "HomeMode"=u32 11, "AxisHandle"=w1777) -> ("AxisHandle"=w1780:u32)  [unwired: 1 in, 2 out]
                    n1132 = call <userlib>:"Acm_AxHome.vi"("DirMode"=u32 1, "HomeMode"=u32 11, "AxisHandle"=w1774) -> ("AxisHandle"=w1773:u32)  [unwired: 1 in, 2 out]
                  }
                  frame #2 {
                    n1133 = Wait Until Next ms Multiple(millisecond multiple=u32 100 ("毫秒倍数")) -> ()  [unwired: 1 out]
                  }
                  frame #3 {
                    n1134 = while {
                      tunnel: w1785 -> [w1793]
                      stop <- w1791 stop-if-true
                      n1135 = call <userlib>:"Acm_AxGetCmdVelocity.vi"("AxisHandle"=w1793) -> ("Velocity"=w1792:dbl)  [unwired: 1 in, 3 out]
                      n1136 = Wait Until Next ms Multiple(millisecond multiple=u32 50 ("毫秒倍数")) -> ()  [unwired: 1 out]
                      n1137 = Equal To 0?(x=w1792) -> (x = 0?=w1791:bool)
                    }
                    n1138 = while {
                      tunnel: w1784 -> [w1789]
                      stop <- w1787 stop-if-true
                      n1139 = call <userlib>:"Acm_AxGetCmdVelocity.vi"("AxisHandle"=w1789) -> ("Velocity"=w1788:dbl)  [unwired: 1 in, 3 out]
                      n1140 = Wait Until Next ms Multiple(millisecond multiple=u32 50 ("毫秒倍数")) -> ()  [unwired: 1 out]
                      n1141 = Equal To 0?(x=w1788) -> (x = 0?=w1787:bool)
                    }
                  }
                  frame #4 {
                    n1142 = call "PCI1220U角度置零.vi"("AxisHandle IN"=w1796) -> ()  [unwired: 10 in, 1 out]
                    n1143 = call "PCI1220U角度置零.vi"("AxisHandle IN"=w1795) -> ("AxisHandle OUT"=w1794:u32)  [unwired: 10 in]
                  }
                  frame #5 {
                    n1144 = while {
                      tunnel: [w1804] -> w1797
                      tunnel: w1798 -> [w1799]
                      stop <- w1803 stop-if-true
                      n1145 = local read "齿条右极限"() -> (w1802:dbl)
                      n1146 = Wait Until Next ms Multiple(millisecond multiple=u32 50 ("毫秒倍数")) -> ()  [unwired: 1 out]
                      n1147 = Add(x=w1802, y=-10.0) -> (x+y=w1800:dbl)
                      n1148 = call "PCI1240电动缸位置模式 .vi"("Distance"=w1800, "AxisHandle IN"=w1799) -> ("AbsSuccess"=w1803:bool, "AxisHandle OUT"=w1804:u32)  [unwired: 8 in]
                    }
                  }
                  frame #6 {
                    n1149 = while {
                      tunnel: w1806 -> [w1810]
                      stop <- w1808 stop-if-true
                      n1150 = call <userlib>:"Acm_AxGetCmdVelocity.vi"("AxisHandle"=w1810) -> ("Velocity"=w1809:dbl)  [unwired: 1 in, 3 out]
                      n1151 = Wait Until Next ms Multiple(millisecond multiple=u32 50 ("毫秒倍数")) -> ()  [unwired: 1 out]
                      n1152 = Equal To 0?(x=w1809) -> (x = 0?=w1808:bool)
                    }
                  }
                }
              }
              frame #1 {
                n1153 = flat-sequence {
                  tunnel: [w1822] -> w1817
                  tunnel: w1817 -> [w1824]
                  tunnel: [w1824] -> w1816
                  tunnel: w1816 -> [w1825]
                  tunnel: [w1825] -> w1815
                  tunnel: w1815 -> [w1831]
                  tunnel: [w1830] -> w1812
                  tunnel: w1812 -> [w1833]
                  tunnel: [w1833] -> w1811
                  tunnel: w1811 -> [w1835]
                  tunnel: [w1834] -> w1814
                  tunnel: w1814 -> [w1841]
                  tunnel: [w1841] -> w1813
                  tunnel: w1813 -> [w1846]
                  frame #0 {
                    n1154 = local write "旋转伺服速度(°/s)"(5.0 ("电动缸速度(mm/s)")) -> ()
                  }
                  frame #1 {
                    n1155 = local read "旋转齿条电机"() -> (w1819:u32)
                    n1156 = call <userlib>:"Acm_AxHome.vi"("DirMode"=u32 0, "HomeMode"=u32 11, "AxisHandle"=w1819) -> ("AxisHandle"=w1822:u32)  [unwired: 1 in, 2 out]
                  }
                  frame #2 {
                    n1157 = Wait Until Next ms Multiple(millisecond multiple=u32 100 ("毫秒倍数")) -> ()  [unwired: 1 out]
                  }
                  frame #3 {
                    n1158 = while {
                      tunnel: w1825 -> [w1829]
                      stop <- w1827 stop-if-true
                      n1159 = call <userlib>:"Acm_AxGetCmdVelocity.vi"("AxisHandle"=w1829) -> ("Velocity"=w1828:dbl)  [unwired: 1 in, 3 out]
                      n1160 = Wait Until Next ms Multiple(millisecond multiple=u32 50 ("毫秒倍数")) -> ()  [unwired: 1 out]
                      n1161 = Equal To 0?(x=w1828) -> (x = 0?=w1827:bool)
                    }
                  }
                  frame #4 {
                    n1162 = call "PCI1220U角度置零.vi"("AxisHandle IN"=w1831) -> ("AxisHandle OUT"=w1830:u32)  [unwired: 10 in]
                  }
                  frame #5 {
                    n1163 = Wait (ms)(milliseconds to wait=u32 100 ("等待时间（毫秒）")) -> ()  [unwired: 1 out]
                  }
                  frame #6 {
                    n1164 = while {
                      tunnel: [w1839] -> w1834
                      tunnel: w1835 -> [w1836]
                      stop <- w1838 stop-if-true
                      n1165 = Wait Until Next ms Multiple(millisecond multiple=u32 50 ("毫秒倍数")) -> ()  [unwired: 1 out]
                      n1166 = call "PCI1220U扭矩轴位置模式.vi"("Distance"=15.0, "AxisHandle IN"=w1836) -> ("AbsSuccess"=w1838:bool, "AxisHandle OUT"=w1839:u32)  [unwired: 8 in]
                    }
                  }
                  frame #7 {
                    n1167 = while {
                      tunnel: w1841 -> [w1844]
                      stop <- w1842 stop-if-true
                      n1168 = call <userlib>:"Acm_AxGetCmdVelocity.vi"("AxisHandle"=w1844) -> ("Velocity"=w1845:dbl)  [unwired: 1 in, 3 out]
                      n1169 = Wait Until Next ms Multiple(millisecond multiple=u32 50 ("毫秒倍数")) -> ()  [unwired: 1 out]
                      n1170 = Equal To 0?(x=w1845) -> (x = 0?=w1842:bool)
                    }
                  }
                  frame #8 {
                    n1171 = call "PCI1220U角度置零.vi"("AxisHandle IN"=w1846) -> ()  [unwired: 10 in, 1 out]
                  }
                }
              }
              frame #2 {
                n1172 = flat-sequence {
                  frame #0 {
                    n1173 = while {
                      stop <- w1850 stop-if-true
                      n1174 = local read "电动缸回零"() -> (w1851:bool)
                      n1175 = local write "电动缸回零"(FALSE ("电动缸回零")) -> ()
                      n1176 = local write "回零完成"(TRUE ("回零完成")) -> ()
                      n1177 = Wait Until Next ms Multiple(millisecond multiple=u32 50 ("毫秒倍数")) -> ()  [unwired: 1 out]
                      n1178 = Not(x=w1851) -> (.not. x?=w1850:bool)
                    }
                  }
                }
              }
            }
          }
        }
      }
    }
    n1179 = Wait (ms)(milliseconds to wait=u32 50 ("毫秒倍数")) -> ()  [unwired: 1 out]
    n1180 = local read "停止"() -> (w1545:bool)
  }
  n1181 = flat-sequence {
    tunnel: [w1855] -> w2
    tunnel: [w1853] -> w1
    tunnel: w2 -> [w1865]
    tunnel: w1 -> [w1864]
    frame #0 {
      n1182 = First Call?() -> (First Call?: T/F=w1852:bool)
      n1183 = case shown="真" w1852 {
        frame False {
        }
        frame True {
          n1184 = while {
            i -> [w1859]
            stop <- w1860 stop-if-true
            w1863 = TRUE ("电动缸使能")
            n1185 = Wait Until Next ms Multiple(millisecond multiple=u32 50 ("毫秒倍数")) -> ()  [unwired: 1 out]
            n1186 = local write "回零完成"(FALSE ("回零完成")) -> ()
            n1187 = local write "测头机构轴使能"(w1863) -> ()
            n1188 = local write "旋转齿条轴使能"(w1863) -> ()
            n1189 = local write "电动缸使能"(w1863) -> ()
            n1190 = Greater Or Equal?(x=w1859, y=u32 30) -> (x >= y?=w1860:bool)
          }
        }
      }
      n1191 = call "ADO Connection Create.vi"() -> ("error out"=w1856:errorcluster, "ADODB._Connection Out"=w1857:refnum<k7>)  [unwired: 10 in]
      n1192 = call "ADO Connection Open.vi"("error in (no error)"=w1856, "ConnectionString"="Provider=Microsoft.Jet.OLEDB.4.0;Data Source=D:\\Q14070-Z060人机界面\\参数\\参数Z060.mdb;Persist Security Info=False;Jet OLEDB:Database Password=123;", "ADODB._Connection In"=w1857) -> ("error out"=w1853:errorcluster, "ADODB._Connection Out"=w1855:refnum<k7>)  [unwired: 7 in]
    }
    frame #1 {
      n1193 = while {
        tunnel: w1865 -> [w1867]
        tunnel: w1864 -> [w1866]
        stop <- w1871 stop-if-true
        n1194 = Wait (ms)(milliseconds to wait=u32 50 ("等待时间（毫秒）")) -> ()  [unwired: 1 out]
        n1195 = First Call?() -> (First Call?: T/F=w1870:bool)
        n1196 = Or(x=w1870, y="参数加载") -> (x .or. y?=w1869:bool)
        n1197 = case shown="真" w1869 {
          tunnel: w1867 -> [_ w1874]
          tunnel: w1866 -> [_ w1873]
          frame False {
          }
          frame True {
            n1198 = stacked-sequence {
              tunnel: w1874 -> [w1880 w1935 w1954]
              tunnel: w1873 -> [w1875 _ _]
              frame #0 {
                n1199 = call "SQL Execute.vi"("error in (no error)"=w1875, "Command Text"="SELECT * FROM 测试参数表", "ADODB._Connection In"=w1880) -> ("Data"=w1878:string[][])  [unwired: 5 in, 3 out]
                n1200 = Index Array(array=w1878, index (col)=0 ("索引 (行)")) -> (element=w1882:string[])  [unwired: 1 in]
                n1201 = Array Size(array=w1882) -> (size(s)=w1877:i32)
                "型号数量" <- w1877
                n1202 = while {
                  shift-right: [w1889] -> w1881
                  shift-left: i32[] [] -> [w1888]
                  tunnel: w1877 -> [w1886]
                  i -> [w1887]
                  stop <- w1885 stop-if-true
                  n1203 = Greater Or Equal?(x=w1887, y=w1886) -> (x >= y?=w1885:bool)
                  n1204 = Build Array (concatenate)(w1888, w1887) -> (w1889:i32[])
                }
                n1205 = Build Cluster Array "索引与捆绑簇数组"(w1882, w1881) -> (w1876:cluster{"String":string, i32}[])
                n1206 = property on="型号选择" class="Ring (严格)"("StringsAndValues[]"=w1876) -> ()  [unwired: 2 in, 2 out]
              }
              frame #1 {
                n1207 = property on="型号选择" class="Ring (严格)"() -> ("RingText.Text"=w1936:string)  [unwired: 2 in, 2 out]
                n1208 = call "创建文本2"("型号选择"=w1936) -> ("Result"=w1940:string)  [unwired: 13 in, 1 out]
                n1209 = call "SQL Execute.vi"("Command Text"=w1940, "ADODB._Connection In"=w1935) -> ("Data"=w1939:string[][])  [unwired: 6 in, 3 out]
                n1210 = Index Array(array=w1939, index (row)=0 ("索引 (行)")) -> (element=w1937:string[])  [unwired: 1 in]
                n1211 = Fract/Exp String To Number ("分数/指数字符串至数值转换")(string=w1937) -> (number=w1924:dbl[])  [unwired: 3 in, 1 out]
                n1212 = Index Array ("索引数组")(array=w1924, index #1=2 ("索引"), index #2=3 ("索引"), index #3=4 ("索引"), index #4=5 ("索引"), index #5=6 ("索引"), index #6=7 ("索引"), index #7=8 ("索引"), index #8=9 ("索引"), index #9=10 ("索引"), index #10=11 ("索引"), index #11=12 ("索引"), index #12=13 ("索引"), index #13=14 ("索引"), index #14=15 ("索引"), index #15=16 ("索引"), index #16=17 ("索引"), index #17=18 ("索引"), index #18=19 ("索引"), index #19=20 ("索引"), index #20=21 ("索引"), index #21=22 ("索引"), index #22=23 ("索引")) -> (element #1=w1923:dbl, element #2=w1922:dbl, element #3=w1921:dbl, element #4=w1920:dbl, element #5=w1919:dbl, element #6=w1918:dbl, element #7=w1917:dbl, element #8=w1916:dbl, element #9=w1915:dbl, element #10=w1914:dbl, element #11=w1913:dbl, element #12=w1912:dbl, element #13=w1896:dbl, element #14=w1906:dbl, element #15=w1905:dbl, element #16=w1904:dbl, element #17=w1900:dbl, element #18=w1899:dbl, element #19=w1897:dbl, element #20=w1895:dbl, element #21=w1891:dbl, element #22=w1890:dbl)
                n1213 = local write "全行程180°内间隙标准(mm)"(w1891) -> ()
                n1214 = local write "全行程180°外间隙标准(mm)"(w1890) -> ()
                n1215 = local write "中间间隙标准(mm)"(w1895) -> ()
                n1216 = local write "测头机构轴移动速度"(w1923) -> ()
                n1217 = local write "测头机构轴检测位"(w1922) -> ()
                n1218 = local write "测头机构轴后退位"(w1920) -> ()
                n1219 = local write "测头机构轴待检位"(w1921) -> ()
                n1220 = local write "旋转伺服找帽转速"(w1916) -> ()
                n1221 = local write "旋转伺服测量转速"(w1915) -> ()
                n1222 = local write "总行程标准(mm)"(w1913) -> ()
                n1223 = local write "齿条移动速度"(w1919) -> ()
                n1224 = local write "平均轴向力MAX(N)"(w1904) -> ()
                n1225 = local write "齿条左极限"(w1918) -> ()
                n1226 = local write "总行程最大值"(w1912) -> ()
                n1227 = local write "齿条右极限"(w1917) -> ()
                n1228 = local write "转向器中心"(w1897) -> ()
                n1229 = local write "总圈数标准"(w1900) -> ()
                n1230 = local write "总圈数最大值"(w1899) -> ()
                n1231 = local write "测量点扭矩"(w1914) -> ()
                n1232 = local write "力波动标准(N)"(w1906) -> ()
                n1233 = local write "轴向力标准(N)"(w1905) -> ()
                n1234 = local write "齿条传动比"(w1896) -> ()
              }
              frame #2 {
                n1235 = call "SQL Execute.vi"("Command Text"="SELECT * FROM 传感器校验表 where ID='1'", "ADODB._Connection In"=w1954) -> ("Data"=w1956:string[][])  [unwired: 6 in, 3 out]
                n1236 = Index Array(array=w1956) -> (element=w1957:string[])  [unwired: 2 in]
                n1237 = Fract/Exp String To Number ("分数/指数字符串至数值转换")(string=w1957) -> (number=w1947:dbl[])  [unwired: 3 in, 1 out]
                n1238 = Index Array(array=w1947, index #1=1 ("索引"), index #2=2 ("索引"), index #3=3 ("索引"), index #4=4 ("索引"), index #5=5 ("索引"), index #6=6 ("索引")) -> (element #1=w1946:dbl, element #2=w1945:dbl, element #3=w1944:dbl, element #4=w1943:dbl, element #5=w1942:dbl, element #6=w1941:dbl)
                n1239 = local write "间隙位移零点偏移"(w1946) -> ()
                n1240 = local write "间隙位移比例偏移"(w1945) -> ()
                n1241 = local write "齿条推拉力零点偏移"(w1944) -> ()
                n1242 = local write "齿条推拉力比例偏移"(w1943) -> ()
                n1243 = local write "齿条扭矩零点偏移"(w1942) -> ()
                n1244 = local write "齿条扭矩比例偏移"(w1941) -> ()
              }
            }
          }
        }
        n1245 = local read "停止"() -> (w1871:bool)
        "ADODB._Connection Out 2" <- w1867
      }
    }
  }
  n1246 = while {
    stop <- w1959 stop-if-true
    n1247 = local read "rfid工步号"() -> (w1958:u32)
    n1248 = case shown="10" w1958 {
      frame 0, Default {
      }
      frame 10 {
        n1249 = flat-sequence {
          tunnel: [w1969] -> w1963
          tunnel: w1963 -> [w1973]
          tunnel: [w1970] -> w1962
          tunnel: w1962 -> [w1975]
          tunnel: [w1975] -> w1961
          tunnel: w1961 -> [w1978]
          frame #0 {
            n1250 = while {
              stop <- w1964 stop-if-true
              n1251 = local read "rfid触发"() -> (w1964:bool)
              n1252 = Wait Until Next ms Multiple(millisecond multiple=u32 50 ("毫秒倍数")) -> ()  [unwired: 1 out]
            }
          }
          frame #1 {
            n1253 = local write "芯片ID"("" ("随行板ID")) -> ()
            n1254 = local write "rfid完成"(FALSE ("RFID完成")) -> ()
            n1255 = local write "rfid触发"(FALSE ("RFID读取触发")) -> ()
          }
          frame #2 {
            n1256 = local read "Z060ARFID"() -> (w1969:string)
            n1257 = local write "芯片ID"(w1969) -> ()
          }
          frame #3 {
            w1971 = T6 0 items=["两端", "字符串首端", "字符串末端"] ("location (both)")
            n1258 = call "查询产品ID.vi"("芯片编码"=w1973) -> ("产品ID"=w1972:string)  [unwired: 8 in, 2 out]
            "读取产品ID" <- w1972
            n1259 = call <vilib>:"Trim Whitespace.vi"("string"=w1972, "location (both)"=w1971) -> ("trimmed string"=w1970:string)
          }
          frame #4 {
            n1260 = Wait Until Next ms Multiple(millisecond multiple=u32 500 ("毫秒倍数")) -> ()  [unwired: 1 out]
          }
          frame #5 {
            n1261 = call "查询上序合格.vi"("产品ID"=w1978) -> ("本序已做"=w1976:bool, "上序合格"=w1977:bool)  [unwired: 8 in, 1 out]
            n1262 = Not(x=w1977) -> (.not. x?=w1979:bool)
            n1263 = local write "上序不合格"(w1979) -> ()
            n1264 = local write "上序合格"(w1977) -> ()
            n1265 = local write "本序已做"(w1976) -> ()
          }
          frame #6 {
            n1266 = local write "rfid完成"(TRUE ("RFID读取完成")) -> ()
            n1267 = Wait Until Next ms Multiple(millisecond multiple=u32 500 ("毫秒倍数")) -> ()  [unwired: 1 out]
          }
          frame #7 {
            "rfid工步号" <- 15.0 ("工步号")
          }
        }
      }
      frame 210 {
        n1268 = local read "读取产品ID"() -> (w1983:string)
        n1269 = local write "产品ID"(w1983) -> ()
      }
    }
    n1270 = Wait Until Next ms Multiple(millisecond multiple=u32 50 ("毫秒倍数")) -> ()  [unwired: 1 out]
    n1271 = local read "停止"() -> (w1959:bool)
  }
  n1272 = flat-sequence {
    tunnel: [w1984] -> w4
    tunnel: w4 -> [w1990]
    tunnel: [w1989] -> w3
    tunnel: w3 -> [w2060]
    frame #0 {
      n1273 = call "PCI1240U初始化.vi"() -> ("旋转电机"=→"旋转齿条电机":u32, "电动缸电机"=→"电动缸电机":u32, "DeviceHandle"=→"DeviceHandle":u32, "进给电机"=→"测头机构电机":u32)  [unwired: 6 in, 2 out]
      n1274 = call "PCI8622配置.vi"() -> ("DeviceID"=w1984:i32)  [unwired: 11 in]
    }
    frame #1 {
      n1275 = while {
        tunnel: w1990 -> [w1992]
        tunnel: [w1991] -> w1989
        stop <- "停止" stop-if-true
        n1276 = stacked-sequence {
          tunnel: w1992 -> [_ _ w2036]
          tunnel: [_ _ w2036] -> w1991
          frame #0 {
            n1277 = local read "测头机构电机"() -> (w2001:u32)
            n1278 = Boolean To (0,1)(Boolean="测头机构轴使能") -> (0, 1=w1999:i16)
            n1279 = call <userlib>:"Acm_AxSetSvOn.vi"("OnOff"=w1999, "AxisHandle"=w2001) -> ("AxisHandle"=w1998:u32)  [unwired: 1 in, 2 out]
            n1280 = call "PCI1220U进给轴速度设置.vi"("Change Velocity"="测头机构轴速度(mm/s)", "AxisHandle IN"=w1998) -> ("AxisHandle OUT"=w1996:u32)  [unwired: 9 in]
            n1281 = call "PCI1220U进给轴读取位置.vi"("AxisHandle IN"=w1996) -> ("位置"=→"测头机构轴位置(mm)":dbl)  [unwired: 9 in, 1 out]
          }
          frame #1 {
            n1282 = local read "电动缸电机"() -> (w2011:u32)
            n1283 = local read "旋转齿条电机"() -> (w2010:u32)
            n1284 = Boolean To (0,1)(Boolean="电动缸使能") -> (0, 1=w2015:i16)
            n1285 = Boolean To (0,1)(Boolean="旋转齿条轴使能") -> (0, 1=w2009:i16)
            n1286 = call <userlib>:"Acm_AxSetSvOn.vi"("OnOff"=w2009, "AxisHandle"=w2010) -> ("AxisHandle"=w2012:u32)  [unwired: 1 in, 2 out]
            n1287 = call <userlib>:"Acm_AxSetSvOn.vi"("OnOff"=w2015, "AxisHandle"=w2011) -> ("AxisHandle"=w2014:u32)  [unwired: 1 in, 2 out]
            n1288 = call "PCI1220U扭矩轴速度设置.vi"("Change Velocity"="旋转伺服速度(°/s)", "AxisHandle IN"=w2012) -> ("AxisHandle OUT"=w2013:u32)  [unwired: 9 in]
            n1289 = call "PCI1240电动缸速度设置.vi"("Change Velocity"="电动缸速度(mm/s)", "AxisHandle IN"=w2014) -> ("AxisHandle OUT"=w2002:u32)  [unwired: 9 in]
            n1290 = call "PCI1220U扭矩轴读取位置.vi"("AxisHandle IN"=w2013) -> ("位置"=→"旋转伺服位置(°)":dbl)  [unwired: 9 in, 1 out]
            n1291 = call "PCI1240电动缸读取位置.vi"("AxisHandle IN"=w2002) -> ("位置"=→"电动缸位置(mm)":dbl)  [unwired: 9 in, 1 out]
          }
          frame #2 {
            w2052 = 0  # nRetSizeWords
            w2053 = 2048  # nReadSizeWords
            # "hDevice"
            n1292 = Initialize Array(u16 0, 2048 ("dimension size")) -> (w2043:u16[])
            n1293 = dll-call lib="PCI8622_32.dll" fn="PCI8622_ReadDeviceProAD_Npt" label="ReadDeviceProAD_Npt"("hDevice"=w2036, "ADBuffer[]"=w2043, "nReadSizeWords"=w2053, "nRetSizeWords"=w2052) -> ("ADBuffer[]"=w2046:u16[])  [unwired: 7 in, 2 out]
            n1294 = Divide(x=w2046, y=65536.01) -> (x/y=w2047:dbl[])
            n1295 = Multiply(x=w2047, y=20) -> (x*y=w2050:dbl[])
            n1296 = Subtract(x=w2050, y=10) -> (x-y=w2042:dbl[])
            n1297 = Decimate 1D Array ("抽取一维数组")(w2042) -> (w2030:dbl[], w2031:dbl[], w2029:dbl[])  [unwired: 5 out]
            n1298 = Add Array Elements(numeric array=w2030) -> (sum=w2039:dbl)
            n1299 = Add Array Elements(numeric array=w2029) -> (sum=w2040:dbl)
            n1300 = Array Size(array=w2030) -> (size(s)=w2038:i32)
            n1301 = Add Array Elements(numeric array=w2031) -> (sum=w2035:dbl)
            n1302 = Array Size(array=w2029) -> (size(s)=w2041:i32)
            n1303 = Array Size(array=w2031) -> (size(s)=w2037:i32)
            n1304 = Divide(x=w2039, y=w2038) -> (x/y=w2028:dbl)
            n1305 = Divide(x=w2040, y=w2041) -> (x/y=w2020:dbl)
            n1306 = Divide(x=w2035, y=w2037) -> (x/y=w2025:dbl)
            n1307 = Subtract(x=w2020, y=2.371) -> (x-y=w2018:dbl)
            n1308 = Multiply(x=w2028, y=2.0) -> (x*y=w2023:dbl)
            n1309 = Multiply(x=w2025, y=200.0) -> (x*y=w2024:dbl)
            n1310 = Subtract(x=w2023, y=-1.0) -> (x-y=w2021:dbl)
            n1311 = Multiply(x=w2018, y=0.75) -> (x*y=w2016:dbl)
            n1312 = local read "间隙位移比例偏移"() -> (w2057:dbl)
            n1313 = local read "间隙位移零点偏移"() -> (w2056:dbl)
            n1314 = local read "齿条扭矩零点偏移"() -> (w2058:dbl)
            n1315 = local read "齿条扭矩比例偏移"() -> (w2059:dbl)
            n1316 = local read "齿条推拉力比例偏移"() -> (w2055:dbl)
            n1317 = local read "齿条推拉力零点偏移"() -> (w2054:dbl)
            n1318 = call "传感器校订.vi"("零点"=w2058, "比例"=w2059, "传感器"=w2021) -> ("示值"=→"齿条扭矩(Nm)":dbl)  [unwired: 8 in]
            n1319 = call "传感器校订.vi"("零点"=w2056, "比例"=w2057, "传感器"=w2016) -> ("示值"=→"间隙位移(mm)":dbl)  [unwired: 8 in]
            n1320 = call "传感器校订.vi"("零点"=w2054, "比例"=w2055, "传感器"=w2024) -> ("示值"=→"齿条推拉力(N)":dbl)  [unwired: 8 in]
          }
        }
        n1321 = Wait Until Next ms Multiple(millisecond multiple=u32 50 ("毫秒倍数")) -> ()  [unwired: 1 out]
      }
    }
    frame #2 {
      n1322 = dll-call lib="PCI8622_32.dll" fn="PCI8622_StopDeviceProAD" label="StopDeviceProAD"("hDevice"=w2060) -> ("hDevice"=w2061:i32)  [unwired: 4 in, 2 out]
      n1323 = dll-call lib="PCI8622_32.dll" fn="PCI8622_ReleaseDeviceProAD" label="ReleaseDeviceProAD"("hDevice"=w2061) -> ()  [unwired: 5 in, 2 out]
      n1324 = dll-call lib="PCI8622_32.dll" fn="PCI8622_ReleaseDevice" label="ReleaseDevice"("hDevice"=w2060) -> ()  [unwired: 5 in, 2 out]
    }
  }
